vi "ControlProgram5.2.vi"() -> ()   [LabVIEW 2016]
uses:
  <vilib>/Utility/error.llb/DialogType.ctl
  <vilib>/Utility/miscctls.llb/LVPoint32TypeDef.ctl
  <vilib>/DAQmx/write.llb/DAQmx Write (Digital Bool 1Line 1Point).vi
  <vilib>/DAQmx/create/channels.llb/DAQmx Create Channel (DO-Digital Output).vi
  <vilib>/platform/TimedLoop/XDataNode/XDataNode.xnode
  <vilib>/Platform/TimedLoop/XDataNode/nitl_modes.ctl
  <vilib>/Platform/TimedLoop/XDataNode/XDNodeRunTimeDep.lvlib
  <vilib>/Platform/TimedLoop/XDataNode/wakeup.ctl
  <vilib>/Platform/TimedLoop/XDataNode/timing_clust.ctl
  <vilib>/DAQmx/create/channels.llb/DAQmx Create Channel (AI-Voltage-Basic).vi
  <vilib>/DAQmx/create/channels.llb/DAQmx Create Channel (AO-Voltage-Basic).vi
  <vilib>/DAQmx/write.llb/DAQmx Write (Analog 1D DBL NChan 1Samp).vi
  <resource>/objmgr/daqmx.rc
  <vilib>/Analysis/NI_AALBase.lvlib
  <vilib>/Analysis/baseanly.llb/Mean (DBL).vi
  <vilib>/Instr/_visa.llb/VISA Configure Serial Port (Instr).vi
  <vilib>/DAQmx/read.llb/DAQmx Read (Analog 2D DBL NChan NSamp).vi
  <vilib>/Utility/inputDevices.llb/closeMouse.vi
  <vilib>/Utility/inputDevices.llb/mouseAcquire.vi
  <vilib>/DAQmx/configure/timing.llb/DAQmx Timing (Sample Clock).vi
panel:
  in  "dt":dbl
  out "Flush Sample Start Time":u32
  out "Sample flush time (s)":dbl=100.0
  in  "Inject Sample":bool
  out "Chart Freq (Hz)":dbl
  out "Waveform Chart 3":dbl[][](graph)
  out "Cal values":T1={"AX alpha"=672.9952101249002, "BX alpha"=822.8320399167465, "AX kappa"=0.3432739170419873, "BX kappa"=0.22087046979741862, "AX offset"=-0.002065833400375715, "BX offset"=0.010483360643544744, "AY alpha"=702.0654168010462, "BY alpha"=773.6701766674906, "AY kappa"=0.33643150106915, "BY kappa"=0.2444549177225145, "AY offset"=-0.1177594339643395, "BY offset"=0.06470506082263472}
  in  "Inject Pump 1":bool
  in  "Inject Pump 2":bool
  in  "Tab Control 2":T2(tab)
  in  "Force FB script":bool
  in  "Got ADig bead":bool
  in  "Move Cap. 2 (ADig Top)":bool
  in  "Dump beads":bool
  in  "Got DNA bead":bool
  in  "Flow on\ncap 2?":bool=TRUE
  in  "Flow on\ncap 1?":bool=TRUE
  in  "Flow on\ndump?":bool=TRUE
  in  "Delta after tether":dbl=3.1
  in  "TA Cancel Save?":bool
  in  "Min fish\ndelta (V)":dbl=2.8 min=0.0 max=10.0 step=0.1
  in  "Max fish\ndelta (V)":dbl=3.8 min=0.0 max=10.0 step=0.1
  in  "Fish Speed (ms)":i32=3000
  in  "Wait (ms)":i32=1500
  in  "# attempts":dbl=10.0
  in  "Cutoff force (pN)":dbl=5.0
  in  "Raster after\n tether?":bool=TRUE
  out "Tether":bool
  out "Attempt #":i32
  in  "Flow on\nwhile fish?":bool=TRUE
  in  "Flow on\nafter raster?":bool=TRUE
  in  "Cal @ Delta (V)":dbl=5.0
  in  "Cal stage position":i32=3
  in  "Conv Y (nm/V)":dbl=505.0
  in  "Conv X (nm/V)":dbl=892.0
  out "Cal Final Sampling Rate":dbl
  in  "Cal Averaging":i32=1
  in  "Wait before dip (s)":dbl=3.0
  in  "Start dipping after?":bool
  in  "Start trap delta (V)":dbl=3.85
  in  "Cancel dwell":bool
  in  "Pause dwell":bool
  in  "Return position":dbl=3.0
  in  "Dip duration":dbl=15.0
  in  "Dip position":dbl=4.0
  in  "Dip":bool
  out "Dip time":i32
  in  "Stop":bool=TRUE
  in  "?":T3(tab)=enum."Mouse control"
  in  "Save N sets":bool
  in  "N sets":i32=200
  in  "Cal sets to save":i32=500
  in  "Reset data stream":bool
  out "Buffer Overflow":bool
  out "Stage moving":bool
  in  "Comment":string="wtUvrD 0.5 uM ATP"
  in  "Raster scan":bool
  out "Saving":bool
  in  "Save cal":bool
  in  "Save Data":bool
  in  "Stop saving":bool
  out "Calibrating":bool
  out "Progress":dbl(slide) scale=0.0..100.0
  in  "Read Cal":bool
  in  "Fish":bool
  in  "Averaging Number":i32=1250
  out "Final Sampling Rate":dbl=100.0
  in  "Trap position":cluster{"X":dbl, "Y":dbl}={"X"=1.6, "Y"=4.95}
  in  "Trap delta":dbl=5.1 min=0.0 max=10.0 step=0.1
  in  "Fixed X":dbl=1.6
  in  "Fixed Y":dbl=0.7
  in  "Shutter 1 (B)":bool
  in  "Shutter 2 (A)":bool
  in  "Pulling direction":bool=TRUE
  out "Raster scanning...":bool
  out "Current file name":path
  in  "AX alpha":dbl format="%#_3p"
  in  "BX alpha":dbl format="%#_3g"
  in  "AX kappa":dbl format="%#_3g"
  in  "BX kappa":dbl format="%#_3g"
  in  "AX offset":dbl format="%#_3g"
  in  "BX offset":dbl format="%#_3g"
  in  "AY alpha":dbl format="%#_3g"
  in  "BY alpha":dbl format="%#_3g"
  in  "AY kappa":dbl format="%#_3g"
  in  "BY kappa":dbl format="%#_3g"
  in  "AY offset":dbl format="%#_3g"
  in  "BY offset":dbl format="%#_3g"
  out "Buffer status":u8(slide) scale=0.0..100.0
  in  "dump spot":string="Dump beads spot"
  in  "up flow spot":string="Upper flow spot"
  in  "low flow spot":string="Lower flow spot"
  in  "up cap":string="Upper capillary (ADig beads)"
  in  "bottom cap":string="Lower capillary (DNA beads)"
  in  "Move to Position 5":bool
  in  "Set Position 5":bool
  in  "Saved stage positions":dbl[][](array[numeric])=[[1.0, 0.0, 0.0, 0.0], [2.0, 0.28481, -2.63158, -0.02256], [3.0, 1.27978, -0.73974, 0.0], [4.0, 1.27978, -2.1978, 0.0], [5.0, 0.03306, -2.63158, -0.02256]]
  in  "Set Position 2":bool
  in  "Move to Position 2":bool
  in  "Set Position 1":bool
  in  "Move to Position 1":bool
  in  "Set Position 4":bool
  in  "Move to Position 4":bool
  in  "Set Position 3":bool
  in  "Move to Position 3":bool
  out "Stage error":errorcluster
  in  "Clear Volume":bool
  out "Sample Flush Meter":u8(slide) scale=0.0..100.0
  out "Flushing Sample":bool
  in  "Flush Sample":bool
  in  "Normal \nRate (ul/hr)  3":dbl=100.0
  in  "Normal \nVolume (ul) 3":dbl=300.0
  in  "Normal \nVolume (ul) 2":dbl
  in  "Normal \nRate (ul/hr)":dbl
  in  "Normal \nVolume (ul)":dbl
  in  "Flush\nRate (ul/min)":dbl
  in  "Flush\nVolume (ul)":dbl
  in  "Flush \nRate (ul/min)  2":dbl
  in  "Flush Pump 2":bool
  in  "Flush\nVolume (ul)  2":dbl
  in  "Flush Pump 1":bool
  in  "Normal \nRate (ul/hr)  2":dbl
  in  "Write Wait":i32=1000
  in  "Flush \nRate (ul/min)  3":dbl=100.0
  in  "Flush\nVolume (ul)  3":dbl=100.0
  out "error out":errorcluster
  in  "Use Mouse to Move Trap?":bool
  in  "Pause Mouse/Mirror Connection":bool
  out "Reference Voltage":cluster{dbl, dbl}={0.0, -0.0}
  out "Saved voltage":cluster{dbl, dbl}
  out "Real Coordinates":cluster{"Horizontal":i32, "Vertical":i32}={"Horizontal"=145, "Vertical"=-1746}
  out "CoordinatesMousePressed":T4
  out "Sum error":dbl(knob) scale=-0.2..0.2
  out "Trap sep":waveform(dbl)[](graph)
  in  "Set reading to\nsetpoint":bool
  in  "Offset Y (nm)":dbl format="%0.2f"
  in  "Offset X (nm)":dbl format="%0.2f"
  in  "Remove offsets":bool
  in  "Force Feedback":bool
  out "Feedback Output Voltage 2":cluster{dbl, dbl} {"?" format="%#_4g"; "?" format="%#_4g"}
  in  "Max value X":dbl=10.0 format="%.1f"
  in  "Min value X":dbl format="%0.1f"
  in  "Max value Y":dbl=10.0 format="%.1f"
  in  "Min value Y":dbl format="%.1g"
  in  "Offset":cluster{"Off Y":dbl, "Off X":dbl}={"Off Y"=1.5, "Off X"=0.17}
  in  "Setpoint voltage":cluster{"SP Y":dbl, "SP X":dbl}={"SP Y"=0.6, "SP X"=0.0}
  in  "Feedback const":T5={"Ki_B_Y"=0.5, "Ki_B_X"=0.0, "Kp Y"=1.0, "Kp X"=0.0}
  out "Mean Trap Pos X 2 (nm)":dbl format="%0.2f"
  out "Mean Trp Pos Y 2 (nm)":dbl format="%0.2f"
  out "T2 X RMS (A)":dbl format="%0.2f"
  out "T2 Y RMS (A)":dbl format="%0.2f"
  in  "Save scans":bool=TRUE
  in  "# scans":i32=1
  in  "Speed (ms)":i32=10000
  in  "Min delta":dbl=3.2
  in  "Load param":bool
  in  "Max delta":dbl=4.1
  in  "Scan Parameters":T6(array[cluster])=[{"Label"="Offset", "Max delta 2"=3.8, "Min delta 2"=2.4, "Speed (ms) 2"=10000, "# scans 2"=1}]
  in  "Trap delta\nafter":dbl=3.6
  in  "Stop raster":bool
  out "Scan Range (nm)":dbl
  out "Scan Speed (nm/s)":dbl
  out "Continue to display?":bool
  out "Video Error":errorcluster
  in  "# Samples/channel (in)":i32=40000 format="%.2f"
  out "Buffer size\n(Samples/channel)":u32
  out "DAQ rate\n(Samples/s)":dbl format="%#_6p"
  out "# Samples/channel":i32=1250
  out "# Samples/channel/s":dbl
  out "AvailSampPerChan":u32
  out "Data update period (s/set)":dbl format="%#_6p"
  out "AvailSampPerChan 2":u32
  in  "PC samp per channel":i32=1000
  in  "Sampling Rate":dbl=125000.0 format="%0.0p"
  in  "DAQ Rate2":dbl=1000000.0 format="%#_6p"
  out "Data period (s)":dbl format="%#_6p"
  in  "Tether break\nforce (pN)":dbl=1.0
  in  "Path":path=path "D:/data"
  in  "Save file index":dbl
  out "Mirror task":refnum<k21>
  in  "HWP1":string="Half waveplate 1: differential trap power"
  in  "HWP0":string="Half waveplate 0: total trap power"
  in  "Move 1":bool
  in  "\"Degrees\" 1":dbl
  in  "Move 0":bool
  in  "\"Degrees\" 0":dbl
  out "Chamber":T7(plugin-control)
  out "Deflection":T4
  in  "Sampling Rate":dbl=125000.0 format="%0.2f"
  in  "Averaging Number":i32=12500
  in  "DAQ Rate":dbl=1000000.0
  out "Final Sampling Rate":dbl
  in  "Tab Control":T8(tab)
  in  "Downsamp\nfact":dbl=250.0
  out "Bead sep":waveform(dbl)[](graph)
  out "Force (pN)":waveform(dbl)[](graph)
  out "Mean force (pN)":dbl format="%0.2f"
  out "Force noise (pN)":dbl format="%0.2f"
  out "Mean Bead Sep\n(nm)":dbl format="%0.2f"
  out "Bead Sep Noise\n(A)":dbl format="%0.2f"
  out "Saved Trap Pos":dbl[][](graph)
  out "PSD 2":cluster{dbl[], dbl[]}(graph)
  out "PSD 1":cluster{dbl[], dbl[]}(graph)
  out "PSD 1 Sum":dbl(slide) scale=0.0..10.0
  out "PSD 2 Sum":dbl(slide) scale=0.0..10.0
  in  "Start":bool
  out "All signals":waveform(dbl)[](graph)
  # "Bead Calibration"
  # "X"
  # "Y"
  # "Pump #1 Controls"
  # "Pump #2 Controls"
  # "Sample Pump Controls"
  # "Retract the pumps manually. Change it back to INFUSE when you're done. Suck it up, don't whine."
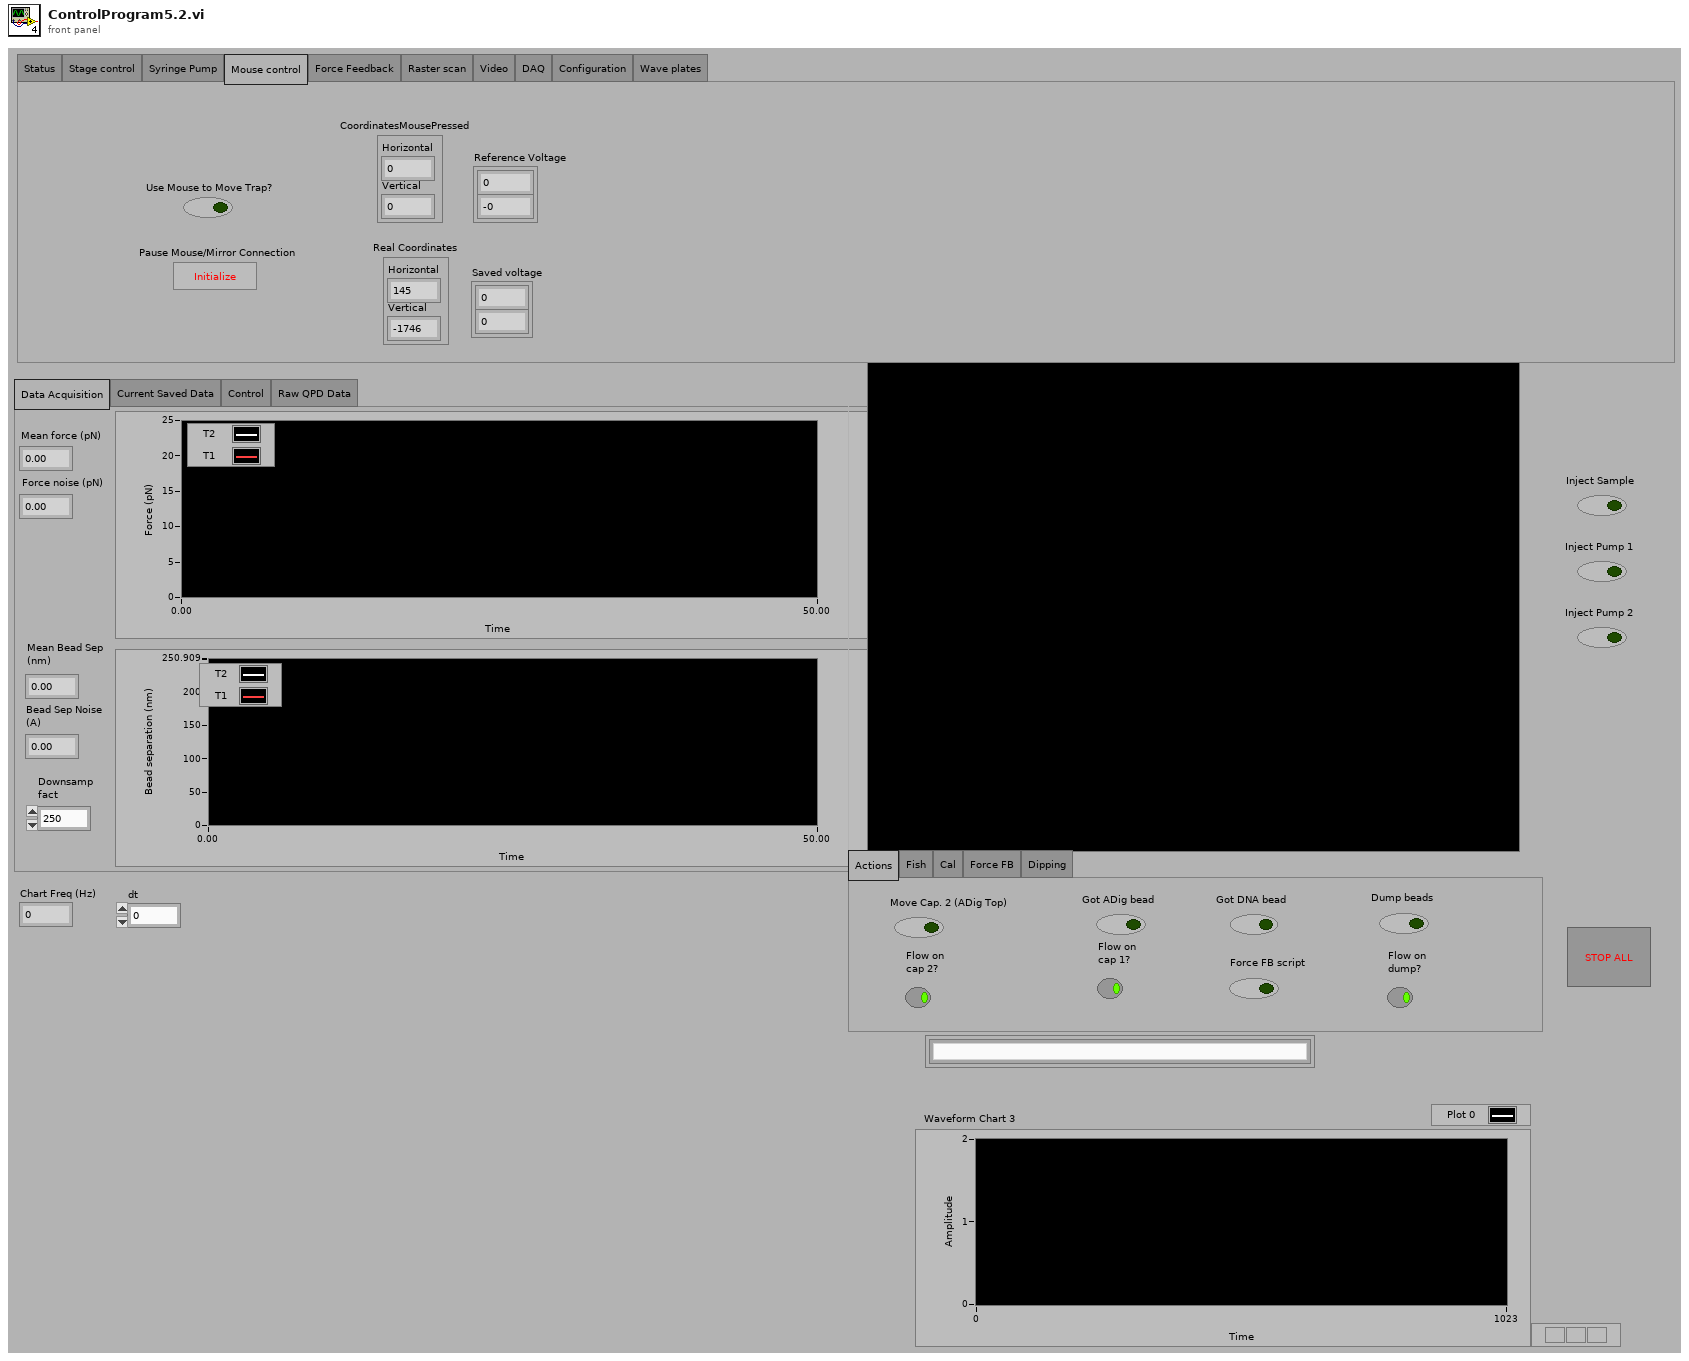
[diagram p1: front panel]
types:
  T1 = cluster{"AX alpha":dbl, "BX alpha":dbl, "AX kappa":dbl, "BX kappa":dbl, "AX offset":dbl, "BX offset":dbl, "AY alpha":dbl, "BY alpha":dbl, "AY kappa":dbl, "BY kappa":dbl, "AY offset":dbl, "BY offset":dbl}
  T2 = enum32{"Actions", "Fish", "Cal", "Force FB", "Dipping"}
  T3 = enum32{"Status", "Stage control", "Syringe Pump", "Mouse control", "Force Feedback", "Raster scan", "Video", "DAQ", "Configuration", "Wave plates"}
  T4 = typedef "LVPoint32TypeDef.ctl" = cluster{"Horizontal":i32, "Vertical":i32}
  T5 = cluster{"Ki_B_Y":dbl, "Ki_B_X":dbl, "Kp Y":dbl, "Kp X":dbl}
  T6 = cluster{"Label":string, "Max delta 2":dbl, "Min delta 2":dbl, "Speed (ms) 2":i32, "# scans 2":i32}[]
  T7 = typedef "IMAQ Image.ctl" = refnum<image>
  T8 = enum32{"Data Acquisition", "Current Saved Data", "Control", "Raw QPD Data"}
  T9 = enum16{"open", "replace", "create", "open or create", "replace or create", "replace or create with confirmation"}
  T10 = enum16{"big-endian, network order", "native, host order", "little-endian"}
  T11 = cluster{string, string, string, string, string, string, string, string}
  T12 = typedef "XDNodeRunTimeDep.lvlib/timing_clust.ctl" = cluster{"Expected End [f-1]":u64, "Actual End [f-1]":u64, "Finished Late? [f-1]":bool, "Expected End [i-1]":u64, "Actual End [i-1]":u64, "Finished Late? [i-1]":bool, "Expected Start [i]":u64, "Actual Start [i]":u64, "Expected Start [f]":u64, "Actual Start [f]":u64, "Source Name":string, "Structure Name":string, "Period":i64, "Deadline":i64, "Offset":i64, "Start":i64, "Priority":i32, "Timeout":i32, "Mode":T13, "Wakeup Reason":T14, "Error":errorcluster, "Source Type":string, "Secondary Source Type":string, "Global End Time":u64, "Global Start Time":u64, "Frame Duration":u64, "Iteration Duration":u64, "Assigned CPU":i32, "I/O Scan Engine Mode":u32}
  T13 = typedef "XDNodeRunTimeDep.lvlib/nitl_modes.ctl" = enum32{"No Change", "Process missed periods, maintain original phase", "Discard missed periods, maintain original phase", "Process missed periods, ignore original phase", "Discard missed periods, ignore original phase"}
  T14 = typedef "XDNodeRunTimeDep.lvlib/wakeup.ctl" = enum32{"Normal", "Aborted", "Asynchronous wakeup", "Timing source error", "Timed loop error", "Timeout"}
  T15 = typedef "DialogType.ctl" = u16
  T16 = cluster{"button 1":bool, "button 2":bool, "button 3":bool, "button 4":bool}
  T17 = cluster{"[0]":dbl, "[1]":dbl, "[2]":dbl, "[3]":dbl, "[4]":dbl, "[5]":dbl, "[6]":dbl, "[7]":dbl, "[8]":dbl, "[9]":dbl, "[10]":dbl, "[11]":dbl}
  T18 = cluster{"Label":string, "Max delta 2":dbl, "Min delta 2":dbl, "Speed (ms) 2":i32, "# scans 2":i32}
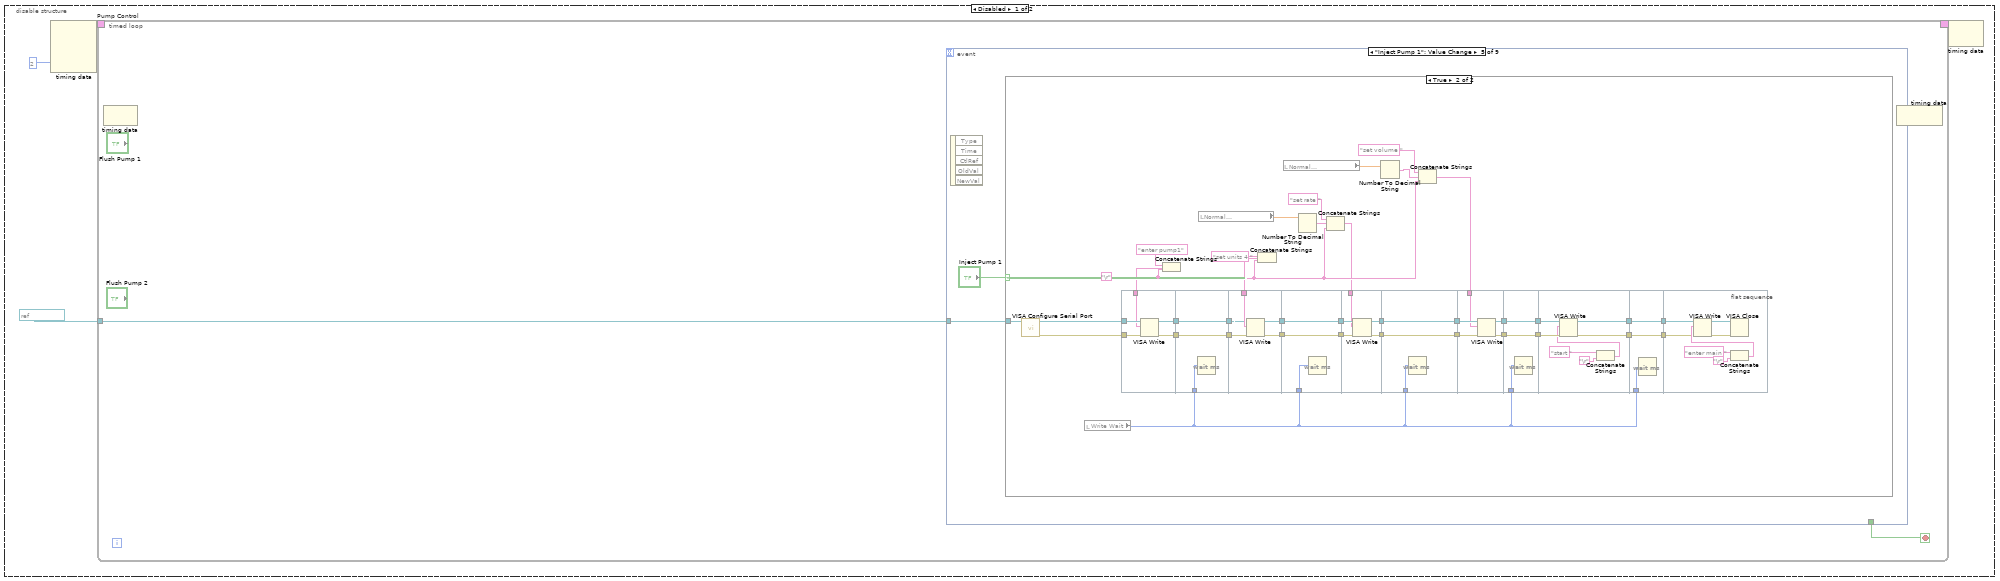
[diagram p2: hidden frame]
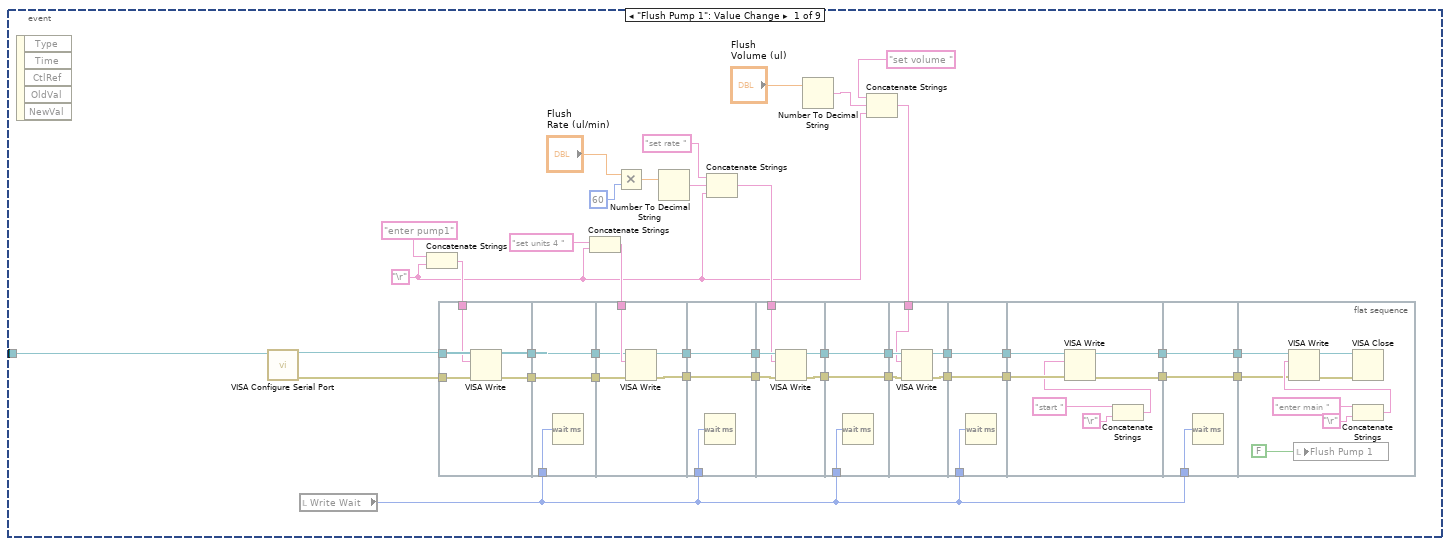
[diagram p3: hidden frame]
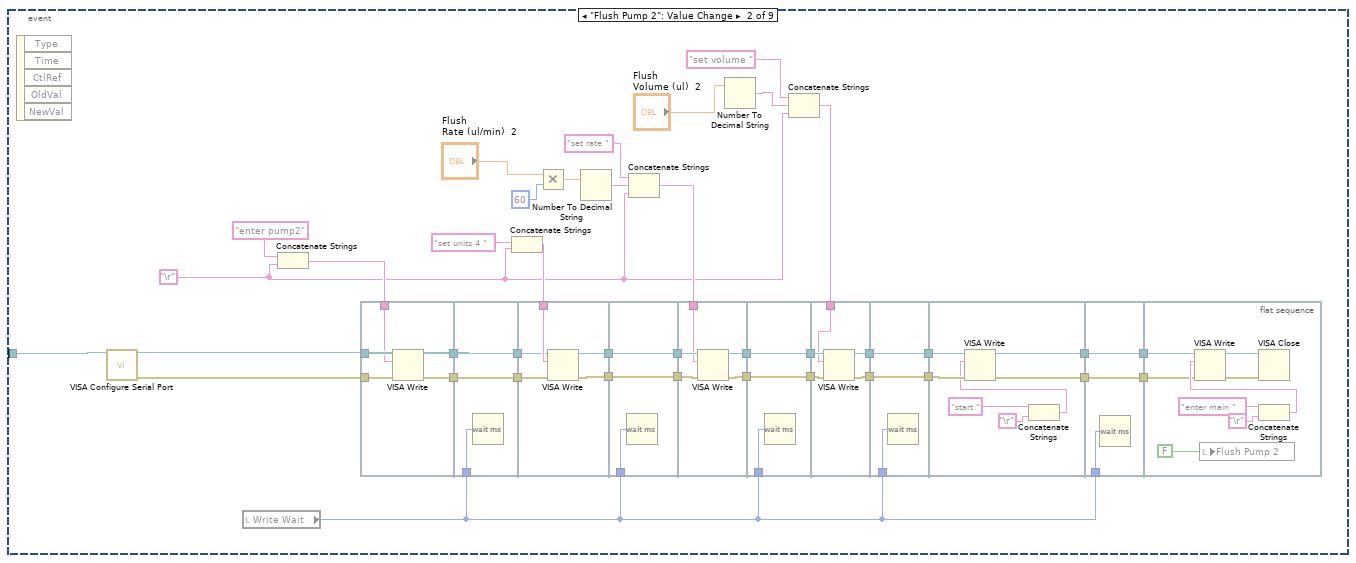
[diagram p4: hidden frame]
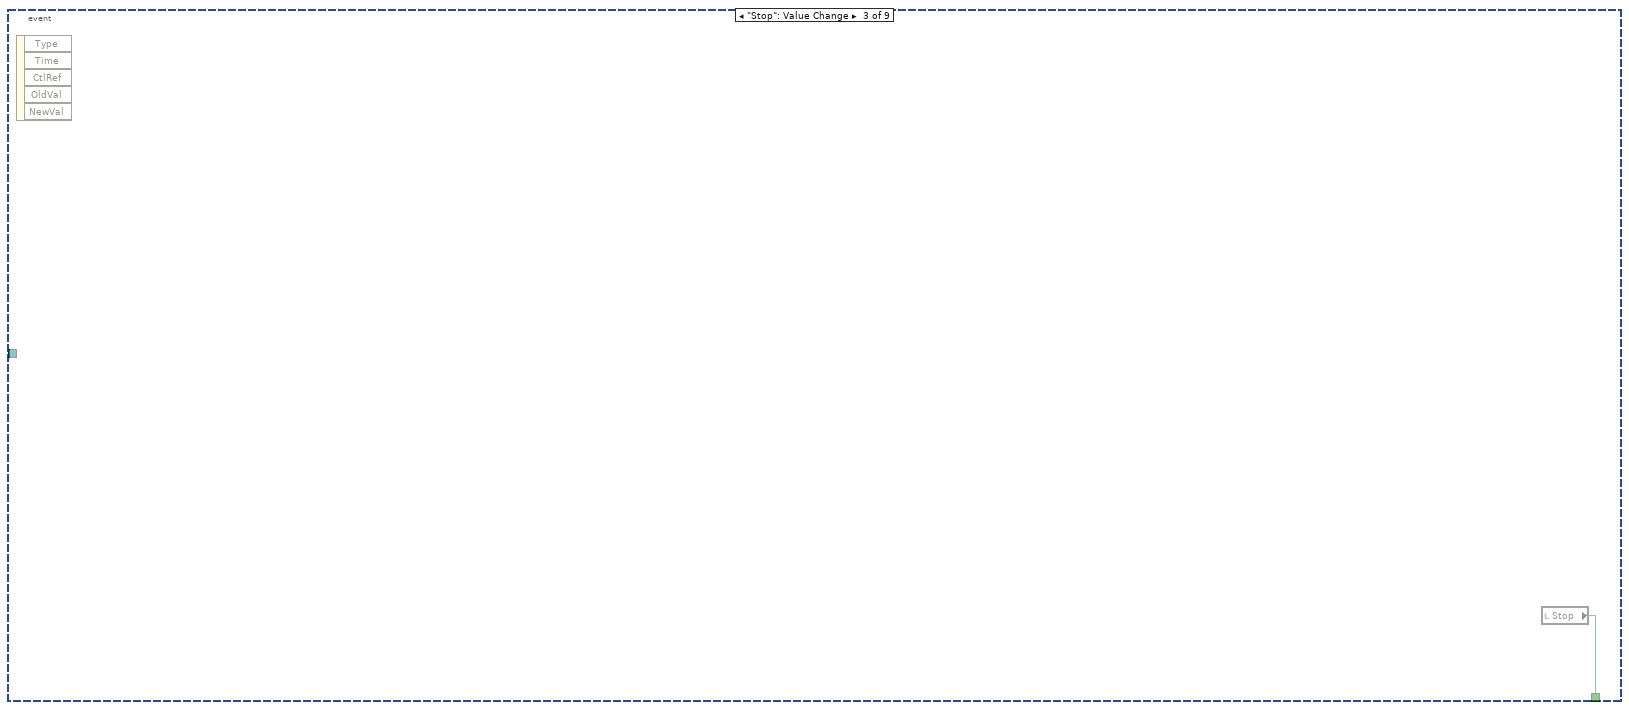
[diagram p5: hidden frame]
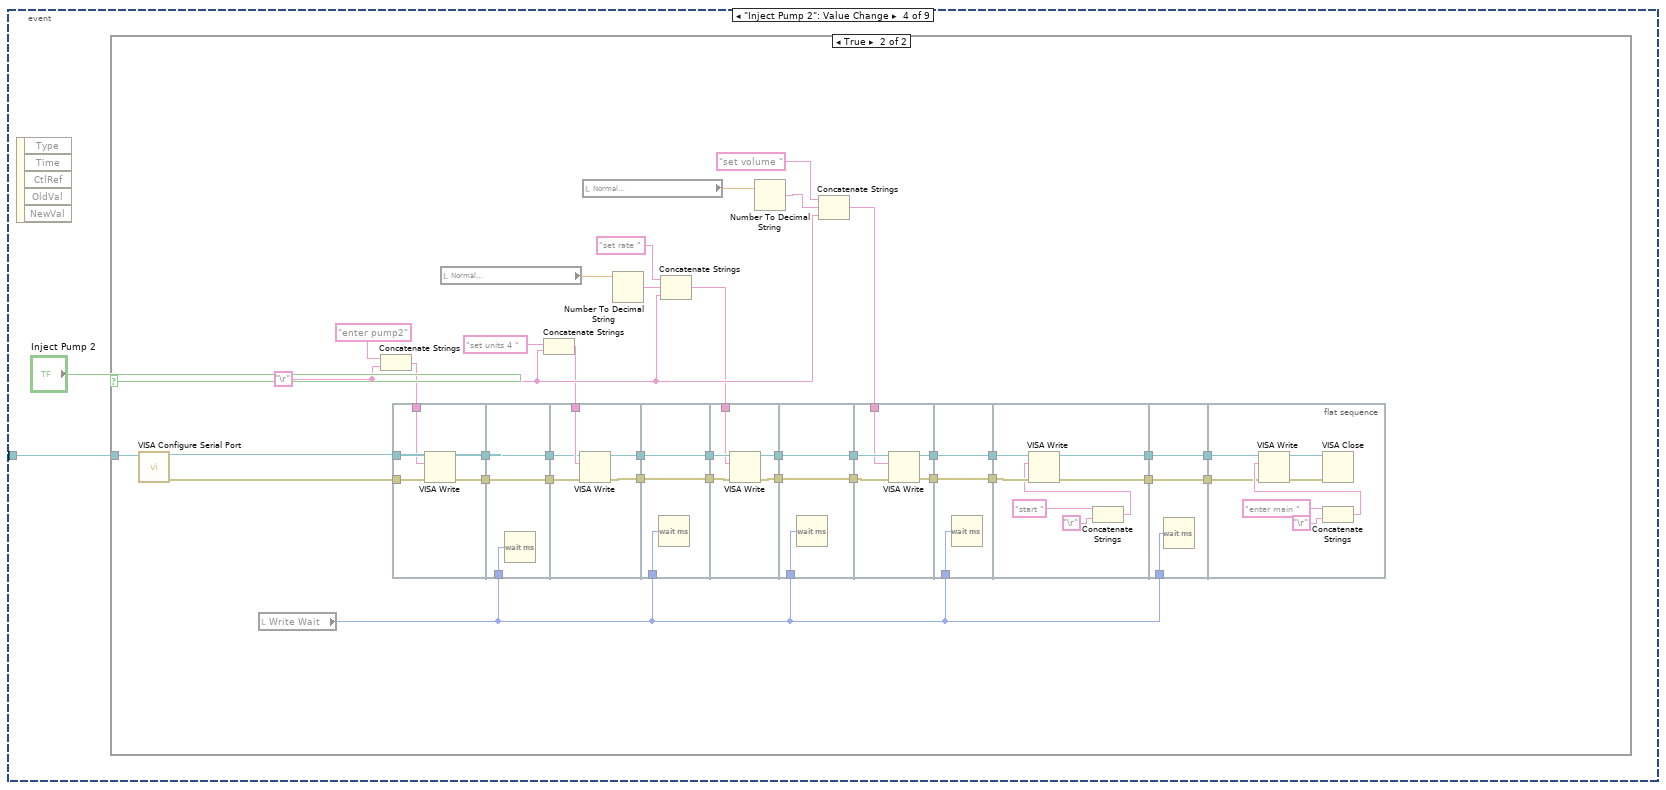
[diagram p6: hidden frame]
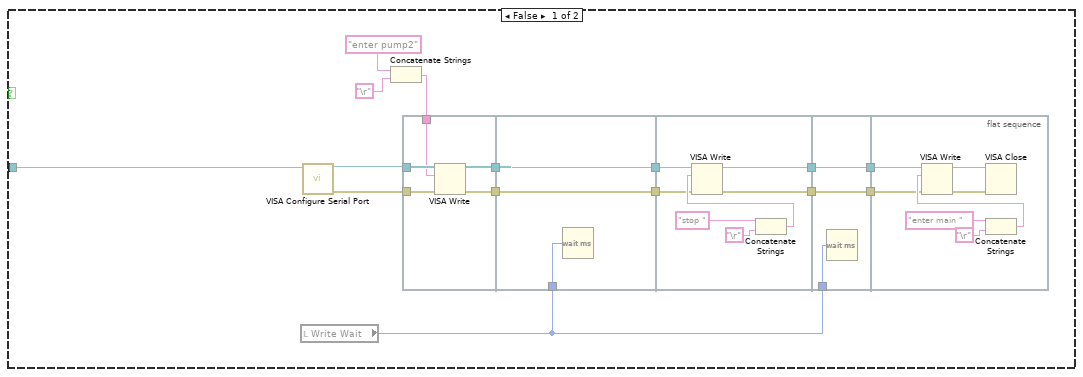
[diagram p7: hidden frame]
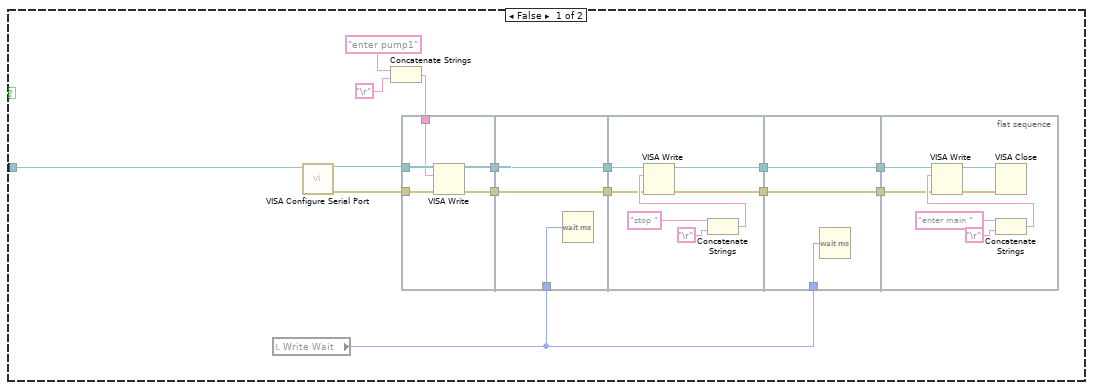
[diagram p8: hidden frame]
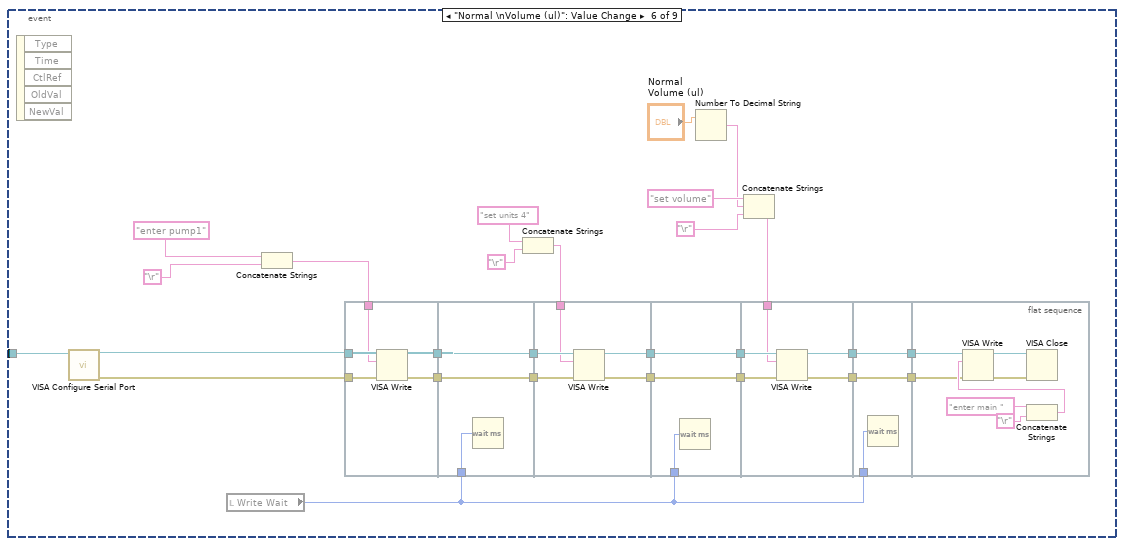
[diagram p9: hidden frame]
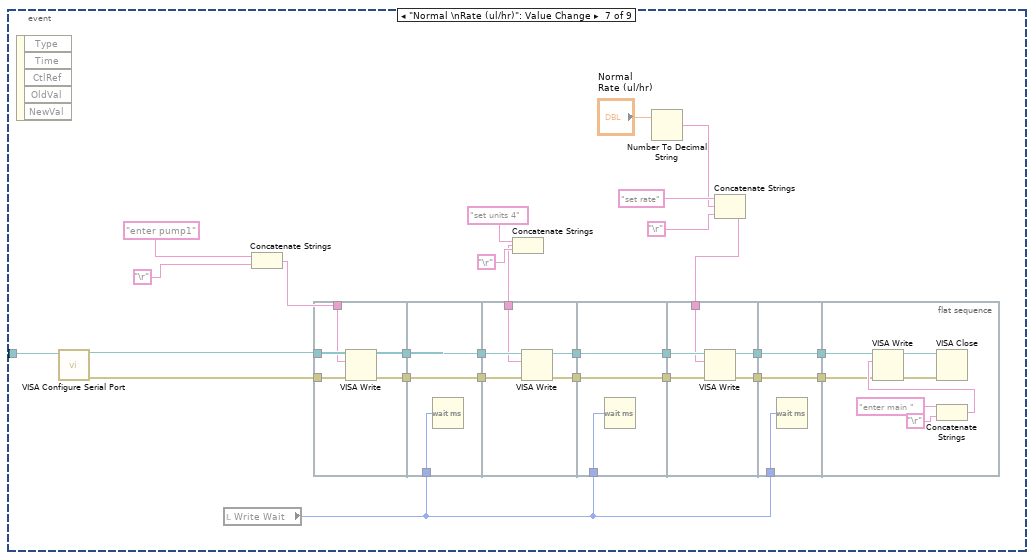
[diagram p10: hidden frame]
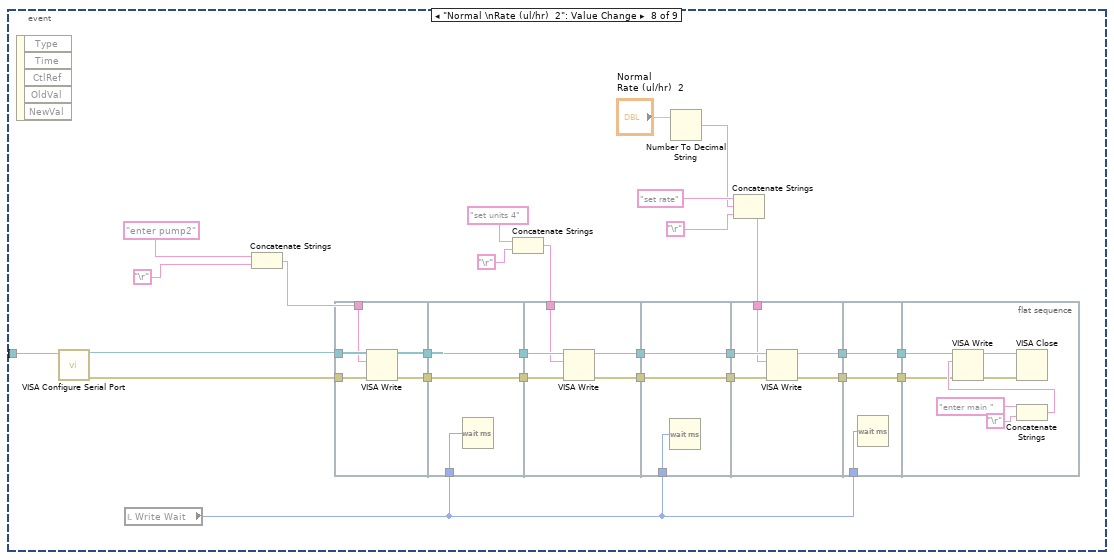
[diagram p11: hidden frame]
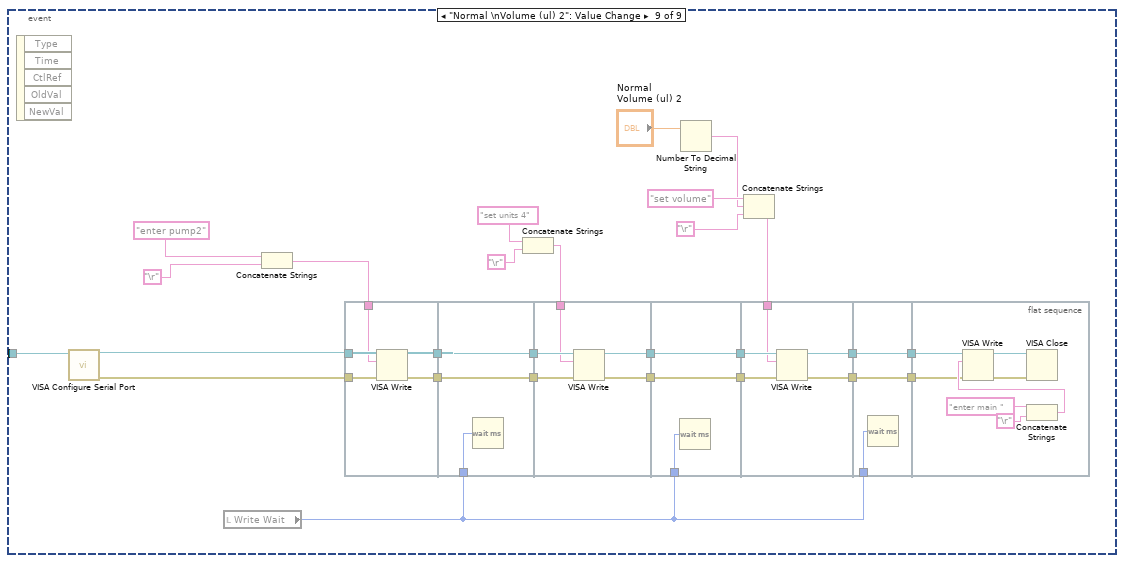
[diagram p12: hidden frame]
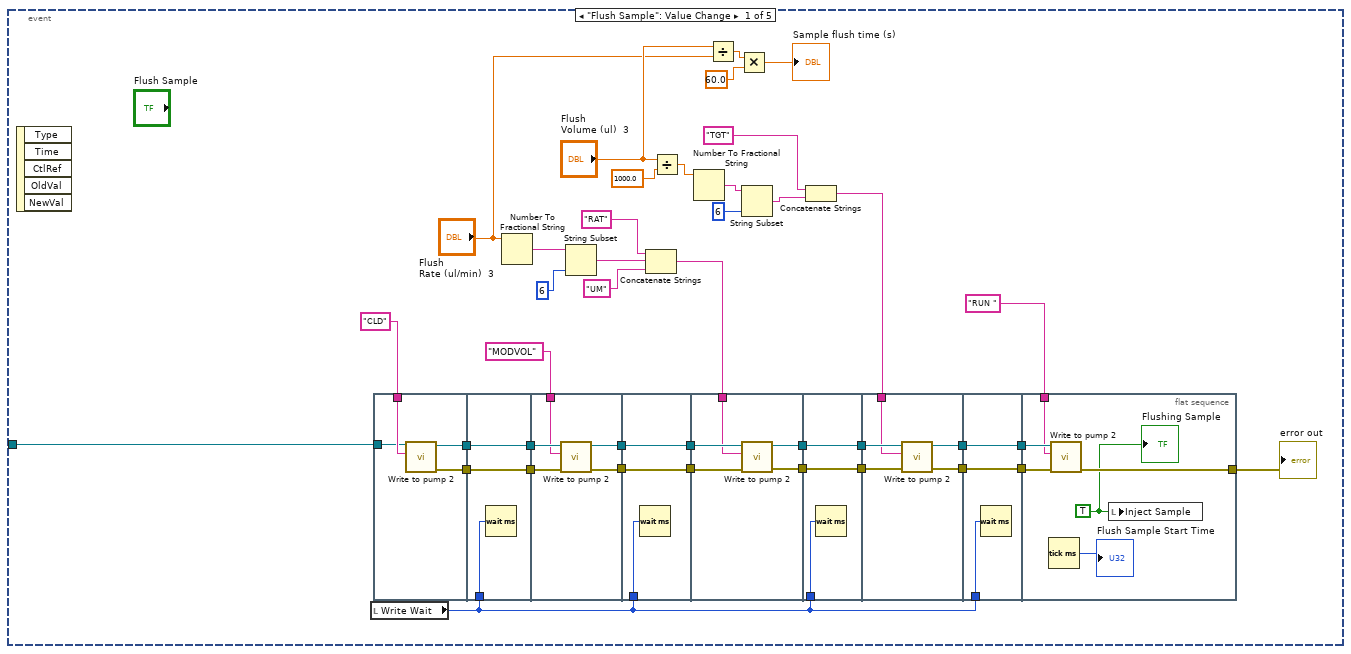
[diagram p13: hidden frame]
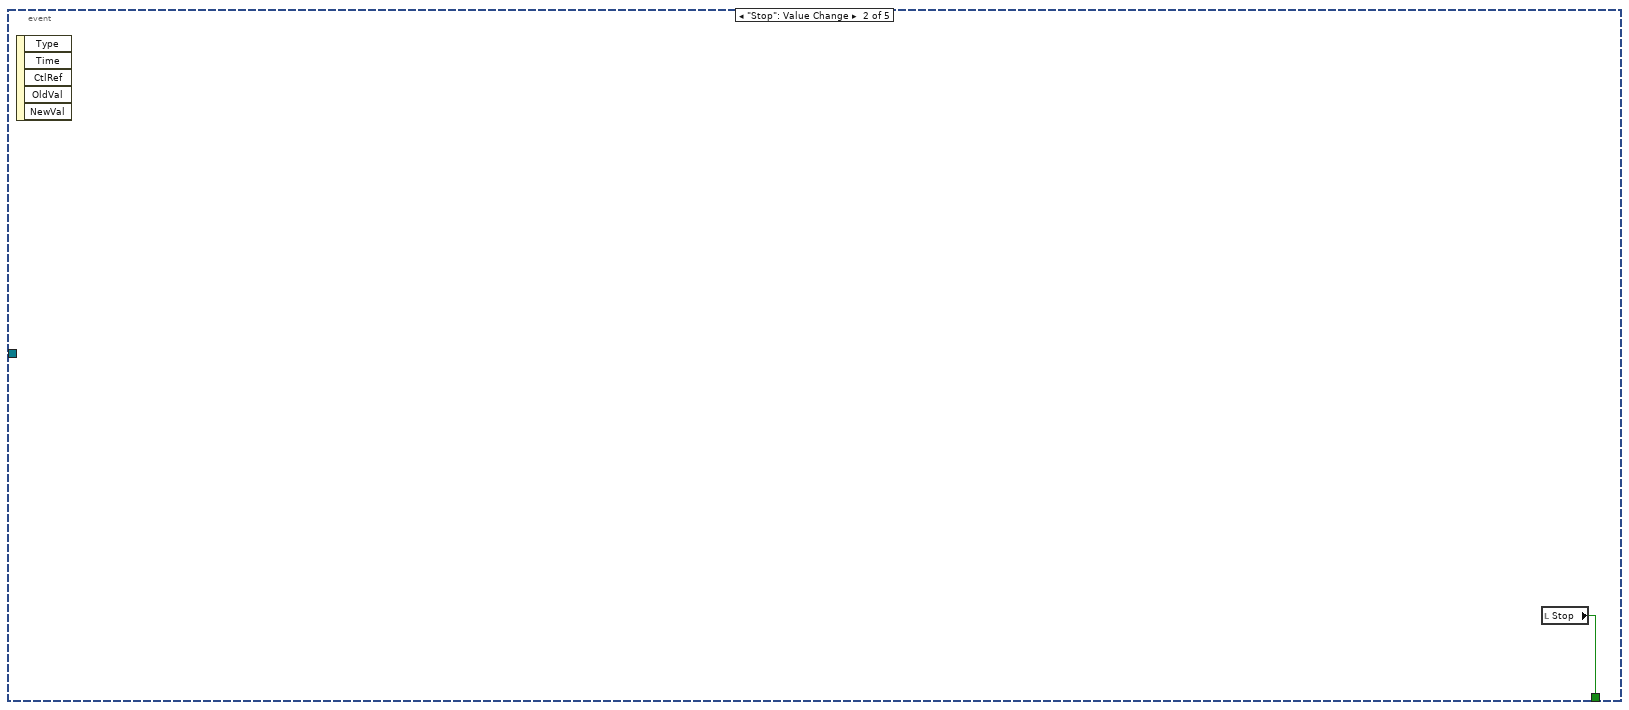
[diagram p14: hidden frame]
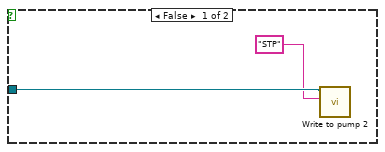
[diagram p15: hidden frame]
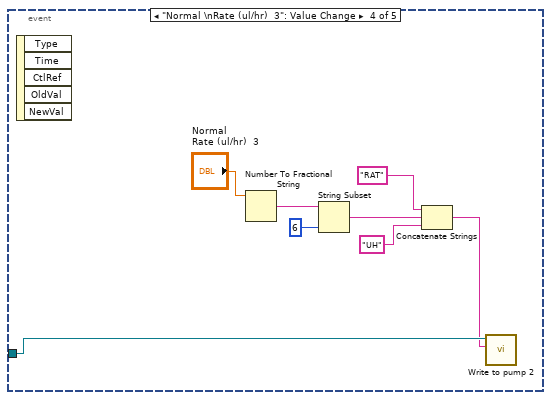
[diagram p16: hidden frame]
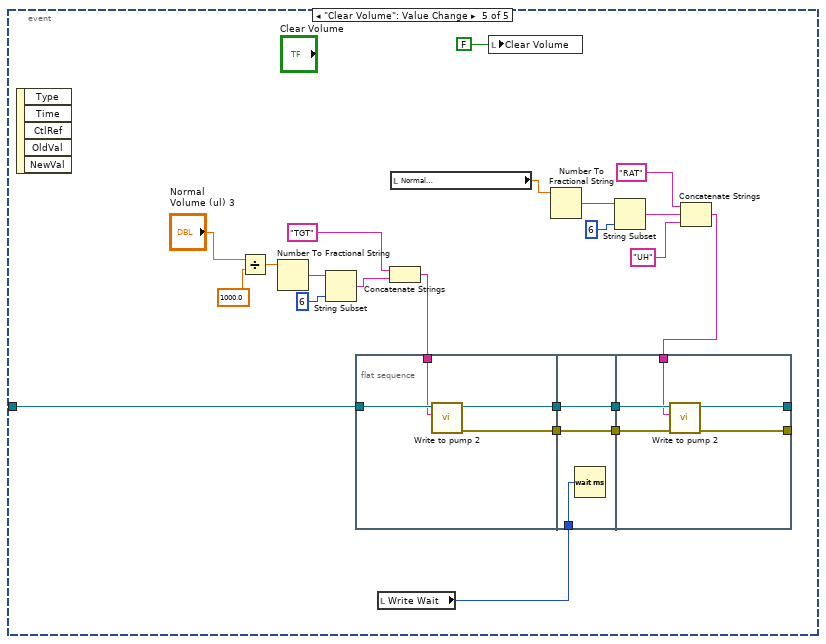
[diagram p17: hidden frame]
diagram:
  w42 = 10.0 ("Minimum Value")
  w43 = -10.0 ("Minimum Value")
  w45 = -2.0 ("Minimum Value")
  w46 = 2.0 ("Maximum Value")
  w71 = 10123 items=["Finite Samples"=10178, "Continuous Samples"=10123] ("sample mode")
  w92 = tag "Dev1/port2/line1"  # Shutter 2
  w95 = tag "Dev1/port1/line4"  # Shutter 1
  # "Create channels for movable mirror"
  # "Create channels for detectors"
  n1 = call-poly <vilib>:"DAQmx Create Virtual Channel.vi"("maximum value"=w46, "minimum value"=w45, "physical channels"=tag "Dev1/ai0" ("Physical Channel")) -> ("task out"=w47:refnum<k21>, "error out"=w70:errorcluster)  [unwired: 11 in]
  n2 = call-poly <vilib>:"DAQmx Create Virtual Channel.vi"("task in"=w47, "maximum value"=w46, "minimum value"=w45, "physical channels"=tag "Dev1/ai1", "error in"=w70) -> ("task out"=w68:refnum<k21>, "error out"=w67:errorcluster)  [unwired: 9 in]
  n3 = call-poly <vilib>:"DAQmx Create Virtual Channel.vi"("task in"=w68, "maximum value"=w46, "minimum value"=w45, "physical channels"=tag "Dev1/ai2", "error in"=w67) -> ("task out"=w59:refnum<k21>, "error out"=w58:errorcluster)  [unwired: 9 in]
  n4 = call-poly <vilib>:"DAQmx Create Virtual Channel.vi"("task in"=w59, "maximum value"=w46, "minimum value"=w45, "physical channels"=tag "Dev1/ai3" ("Physical Channel"), "error in"=w58) -> ("task out"=w44:refnum<k21>, "error out"=w64:errorcluster)  [unwired: 9 in]
  n5 = call-poly <vilib>:"DAQmx Create Virtual Channel.vi"("task in"=w44, "maximum value"=w42, "minimum value"=w43, "physical channels"=tag "Dev1/ai4", "error in"=w64) -> ("task out"=w62:refnum<k21>, "error out"=w61:errorcluster)  [unwired: 9 in]
  n6 = call-poly <vilib>:"DAQmx Create Virtual Channel.vi"("task in"=w62, "maximum value"=w42, "minimum value"=w43, "physical channels"=tag "Dev1/ai5", "error in"=w61) -> ("task out"=w57:refnum<k21>, "error out"=w56:errorcluster)  [unwired: 9 in]
  n7 = call-poly <vilib>:"DAQmx Create Virtual Channel.vi"("task in"=w57, "maximum value"=w42, "minimum value"=w43, "physical channels"=tag "Dev1/ai6", "error in"=w56) -> ("task out"=w51:refnum<k21>, "error out"=w49:errorcluster)  [unwired: 9 in]
  n8 = call-poly <vilib>:"DAQmx Create Virtual Channel.vi"("task in"=w51, "maximum value"=w42, "minimum value"=w43, "physical channels"=tag "Dev1/ai7", "error in"=w49) -> ("task out"=w50:refnum<k21>, "error out"=w48:errorcluster)  [unwired: 9 in]
  n9 = call-poly <vilib>:"DAQmx Timing.vi"("task/channels in"=w50, "sample mode"=w71, "samples per channel"="PC samp per channel", "rate"="Sampling Rate", "error in"=w48) -> ("task out"=w54:refnum<k21>, "error out"=w53:errorcluster)  [unwired: 9 in]
  n10 = call-poly <vilib>:"DAQmx Create Virtual Channel.vi"("maximum value"="Max value Y", "minimum value"="Min value Y", "physical channels"=tag "Dev1/ao1" ("Trap X Axis")) -> ("task out"=w39:refnum<k21>, "error out"=w41:errorcluster)  [unwired: 11 in]
  n11 = property class="DAQmx Timing"(reference=w54, error in=w53, "More:AI Convert:Rate"="DAQ Rate2") -> (reference out=w6:refnum<k21>, error out=w5:errorcluster, "SampClk.Rate"=→"DAQ rate\n(Samples/s)":dbl)
  n12 = call-poly <vilib>:"DAQmx Create Virtual Channel.vi"("task in"=w39, "maximum value"="Max value X", "minimum value"="Min value X", "physical channels"=tag "Dev1/ao0" ("Trap Y Axis"), "error in"=w41) -> ("task out"=w30:refnum<k21>, "error out"=w29:errorcluster)  [unwired: 9 in]
  "Mirror task" <- w30
  n13 = property class="DAQmx Buffer"(reference=w6, error in=w5) -> (reference out=w3:refnum<k21>, error out=w2:errorcluster, "Input.OnbrdBufSize"=→"Buffer size\n(Samples/channel)":u32)
  n14 = call <vilib>:"DAQmx Start Task.vi"("task/channels in"=w3, "error in"=w2) -> ("task out"=w31:refnum<k21>)  [unwired: 12 in, 1 out]
  n15 = while {
    tunnel: [w415] -> w77
    tunnel: [w307] -> w78
    tunnel: [w423] -> w76
    tunnel: [w420] -> w73
    tunnel: w31 -> [w120]
    tunnel: w30 -> [w416]
    tunnel: w29 -> [w421]
    stop <- w420 stop-if-true
    w151 = "NI_ChannelName" ("name")
    w227 = -1
    # "Rewire everything"
    # "Invert these because changed\nfrom PSD to QPD"
    # "Trap Y"
    # "Trap X"
    # "Convert to\npN"
    # "Convert to\nnm"
    # "Subtract\noffset"
    # "Normalize by\nsum"
    # "B sum"
    # "BX"
    # "BY"
    # "AX"
    # "AY"
    # "A sum"
    # "Close files when done saving"
    n16 = property class="DAQmx Read"(reference=w120) -> (reference out=w119:refnum<k21>, "AvailSampPerChan"=→"AvailSampPerChan 2":u32)  [unwired: 1 in, 1 out]
    n17 = local read "Averaging Number"() -> (w115:i32)
    n18 = local read "Averaging Number"() -> (w121:i32)
    "# Samples/channel" <- w121
    n19 = local read "Sampling Rate"() -> (w419:dbl)
    n20 = call-poly <vilib>:"DAQmx Read.vi"("task/channels in"=w119, "number of samples per channel"=w115, "timeout"=10.0) -> ("task out"=w306:refnum<k21>, "data"=w116:dbl[][], "error out"=w230:errorcluster)  [unwired: 10 in]
    n21 = Unbundle By Name(w230) -> ("status"=w355:bool)
    n22 = Divide(x=w419, y="Cal Averaging") -> (x/y=→"Cal Final Sampling Rate":dbl)
    n23 = Divide(x=w419, y=w121) -> (x/y=→"Final Sampling Rate" →"# Samples/channel/s":dbl)
    n24 = case shown="True" w355 {
      frame False {
      }
      frame True {
        n25 = call <vilib>:"Beep.vi"() -> ()  [unwired: 12 in]
        "Buffer Overflow" <- TRUE
      }
    }
    n26 = local read "Buffer size\n(Samples/channel)"() -> (w302:u32)
    n27 = property class="DAQmx Read"(reference=w306) -> (reference out=w305:refnum<k21>, "AvailSampPerChan"=w303:u32)  [unwired: 1 in, 1 out]
    "AvailSampPerChan" <- w303
    n28 = local read "Cal values"() -> (w347:T1)
    n29 = Index Array(array=w116, index (row)=4) -> (element=w219:dbl[])  [unwired: 1 in]
    n30 = Index Array(array=w116, index (row)=0) -> (element=w229:dbl[])  [unwired: 1 in]
    n31 = Index Array(array=w116, index (row)=2) -> (element=w224:dbl[])  [unwired: 1 in]
    n32 = Index Array(array=w116, index (row)=1) -> (element=w228:dbl[])  [unwired: 1 in]
    n33 = Index Array(array=w116, index (row)=3) -> (element=w222:dbl[])  [unwired: 1 in]
    n34 = Index Array(array=w116, index (row)=6) -> (element=w221:dbl[])  [unwired: 1 in]
    n35 = Index Array(array=w116, index (row)=7) -> (element=w220:dbl[])  [unwired: 1 in]
    n36 = Index Array(array=w116, index (row)=5) -> (element=w218:dbl[])  [unwired: 1 in]
    n37 = Divide(x=w303, y=w302) -> (x/y=→"Buffer status":dbl)
    n38 = Unbundle(w347) -> ("AX alpha"=w335:dbl, "BX alpha"=w331:dbl, "AX kappa"=w327:dbl, "BX kappa"=w323:dbl, "AX offset"=w341:dbl, "BX offset"=w339:dbl, "AY alpha"=w338:dbl, "BY alpha"=w333:dbl, "AY kappa"=w329:dbl, "BY kappa"=w325:dbl, "AY offset"=w345:dbl, "BY offset"=w343:dbl)
    n39 = Multiply(x=w228, y=w227) -> (x*y=w223:dbl[])
    n40 = Multiply(x=w229, y=w227) -> (x*y=w225:dbl[])
    n41 = local write "AX alpha"(w335) -> ()
    n42 = local write "BY offset"(w343) -> ()
    n43 = Build Array(w225, w224, w223, w222, w221, w220, w219, w218) -> (w148:dbl[][])
    n44 = local write "BX alpha"(w331) -> ()
    n45 = case shown="True" "Reset data stream" {
      selector: "Reset data stream" -> [_ w466]
      tunnel: w305 -> [w458 w464]
      tunnel: [w458 w462] -> w307
      tunnel: w230 -> [w457 w461]
      tunnel: [w457 w459] -> _
      frame False {
      }
      frame True {
        n46 = Not(x=w466) -> (.not. x?=w465:bool)
        n47 = call <vilib>:"DAQmx Stop Task.vi"("task/channels in"=w464, "error in"=w461) -> ("task out"=w463:refnum<k21>, "error out"=w460:errorcluster)  [unwired: 12 in]
        n48 = local write "Reset data stream"(w465) -> ()
        n49 = local write "Buffer Overflow"(w465) -> ()
        n50 = call <vilib>:"DAQmx Start Task.vi"("task/channels in"=w463, "error in"=w460) -> ("task out"=w462:refnum<k21>, "error out"=w459:errorcluster)  [unwired: 12 in]
      }
    }
    n51 = call-poly <vilib>:"Mean.vi"("X"=w218) -> ("mean"=w361:dbl)  [unwired: 1 out]
    n52 = local write "AY offset"(w345) -> ()
    n53 = call-poly <vilib>:"Mean.vi"("X"=w219) -> ("mean"=w362:dbl)  [unwired: 1 out]
    n54 = call-poly <vilib>:"Mean.vi"("X"=w224) -> ("mean"=w368:dbl)  [unwired: 1 out]
    n55 = call-poly <vilib>:"Mean.vi"("X"=w222) -> ("mean"=w366:dbl)  [unwired: 1 out]
    n56 = call-poly <vilib>:"Mean.vi"("X"=w221) -> ("mean"=w365:dbl)  [unwired: 1 out]
    n57 = call-poly <vilib>:"Mean.vi"("X"=w220) -> ("mean"=w364:dbl)  [unwired: 1 out]
    n58 = local read "Averaging Number"() -> (w114:i32)
    n59 = local write "BY kappa"(w325) -> ()
    n60 = local write "AX kappa"(w327) -> ()
    n61 = call-poly <vilib>:"Mean.vi"("X"=w223) -> ("mean"=w367:dbl)  [unwired: 1 out]
    n62 = local write "AY kappa"(w329) -> ()
    n63 = call-poly <vilib>:"Mean.vi"("X"=w225) -> ("mean"=w369:dbl)  [unwired: 1 out]
    n64 = local read "DAQ rate\n(Samples/s)"() -> (w126:dbl)
    n65 = Build Array(w362, w361) -> (w360:dbl[])
    n66 = local write "BX kappa"(w323) -> ()
    n67 = local write "BY alpha"(w333) -> ()
    n68 = local write "AX offset"(w341) -> ()
    n69 = local write "BX offset"(w339) -> ()
    n70 = local write "AY alpha"(w338) -> ()
    n71 = Build Array(w369, w368, w367, w366, w365, w364) -> (w358:dbl[])
    n72 = Divide(x=w114, y=w126) -> (x/y=w123:dbl)
    "Data update period (s/set)" <- w123
    n73 = Reciprocal(x=w126) -> (1/x=w127:dbl)
    "Data period (s)" <- w127
    n74 = Divide(x=w369, y=w365) -> (x/y=w399:dbl)
    n75 = Divide(x=w368, y=w365) -> (x/y=w400:dbl)
    n76 = Divide(x=w367, y=w364) -> (x/y=w407:dbl)
    n77 = Divide(x=w366, y=w364) -> (x/y=w408:dbl)
    n78 = Subtract(x=w399, y="AY offset") -> (x-y=w381:dbl)
    n79 = Subtract(x=w400, y="AX offset") -> (x-y=w382:dbl)
    n80 = Subtract(x=w407, y="BY offset") -> (x-y=w380:dbl)
    n81 = Subtract(x=w408, y="BX offset") -> (x-y=w383:dbl)
    n82 = Subtract(x=w407, y=w399) -> (x-y=w397:dbl)
    n83 = Subtract(x=w408, y=w400) -> (x-y=w398:dbl)
    n84 = feedback #1(0.0) -> (w301:dbl)
    n85 = Multiply(x="Downsamp\nfact", y=w127) -> (x*y=w128:dbl)
    n86 = Multiply(x=w381, y="AY alpha") -> (x*y=w315:dbl)
    n87 = Multiply(x=w382, y="AX alpha") -> (x*y=w313:dbl)
    n88 = Multiply(x=w383, y="BX alpha") -> (x*y=w314:dbl)
    n89 = Multiply(x=w380, y="BY alpha") -> (x*y=w316:dbl)
    n90 = Add(x=w123, y=w301) -> (x+y=w299:dbl)
    n91 = feedback-in #1(w299) -> ()
    n92 = Square(x=w315) -> (x^2=w391:dbl)
    n93 = Square(x=w313) -> (x^2=w392:dbl)
    n94 = Square(x=w316) -> (x^2=w393:dbl)
    n95 = Square(x=w314) -> (x^2=w394:dbl)
    n96 = Bundle(w397, w398) -> (w117:cluster{dbl, dbl})  [unwired: 1 in]
    n97 = case shown="True" "Set reading to\nsetpoint" {
      tunnel: w117 -> [_ w455]
      frame False {
      }
      frame True {
        n98 = local write "Set reading to\nsetpoint"(FALSE ("Set reading to\nsetpoint")) -> ()
        n99 = local read "Trap position"() -> (w454:cluster{"X":dbl, "Y":dbl})
        n100 = property on="Setpoint voltage" class="Clust (strict)"("Val(Sgnl)"=w455) -> ()  [unwired: 2 in, 2 out]
        n101 = Unbundle(w454) -> ("X"=w453:dbl, "Y"=w452:dbl)
        n102 = Bundle("Y"=w452, "X"=w453) -> (w451:cluster{"Y":dbl, "X":dbl})  [unwired: 1 in]
        n103 = property on="Offset" class="Clust (strict)"("Val(Sgnl)"=w451) -> ()  [unwired: 2 in, 2 out]
      }
    }
    n104 = Reciprocal(x=w128) -> (1/x=→"Chart Freq (Hz)":dbl)
    n105 = To Time Stamp(1:w299) -> (0:w298:timestamp)
    n106 = Add(x=w391, y=w392) -> (x+y=w395:dbl)
    n107 = Add(x=w393, y=w394) -> (x+y=w406:dbl)
    n108 = Multiply(x=w313, y="AX kappa") -> (x*y=w309:dbl)
    n109 = Bundle("A y", "A x", "B y", "B x", "A sum", "B sum", "Trap x", "Trap y") -> (w289:T11)  [unwired: 1 in]
    n110 = Multiply(x=w314, y="BX kappa") -> (x*y=w310:dbl)
    n111 = Square Root(x=w395) -> (sqrt(x)=w411:dbl)
    n112 = Square Root(x=w406) -> (sqrt(x)=w410:dbl)
    n113 = Multiply(x=w315, y="AY kappa") -> (x*y=w311:dbl)
    n114 = Multiply(x=w316, y="BY kappa") -> (x*y=w312:dbl)
    n115 = Subtract(x=w361, y="Fixed Y") -> (x-y=w396:dbl)
    n116 = Subtract(x=w362, y="Fixed X") -> (x-y=w401:dbl)
    n117 = Cluster To Array(cluster=w289) -> (array=w288:string[])
    n118 = for {
      tunnel: w148 -> [w443] mode=indexing
      tunnel: w128 -> [_]
      tunnel: "Downsamp\nfact" -> [w448]
      tunnel: [w446] -> w204 mode=indexing
      tunnel: w298 -> [w450]
      tunnel: w288 -> [w445] mode=indexing
      tunnel: "NI_ChannelName" ("name") -> [w444]
      n119 = call "Downsample 1D array.vi"("Ave N"=w448, "Arrray In"=w443) -> ("Array Out"=w449:dbl[])  [unwired: 9 in]
      n120 = Bundle By Name("Y"=w449, "dt"="dt", "t0"=w450) -> (w447:waveform(dbl))  [unwired: 1 in]
      n121 = Set Waveform Attribute(5:w445, 6:w444, 7:w447) -> (3:w446:waveform(dbl))  [unwired: 1 in, 2 out]
    }
    "All signals" <- w204
    n122 = Square(x=w311) -> (x^2=w384:dbl)
    n123 = Square(x=w309) -> (x^2=w385:dbl)
    n124 = Square(x=w312) -> (x^2=w386:dbl)
    n125 = Square(x=w310) -> (x^2=w387:dbl)
    n126 = Add(x=w384, y=w385) -> (x+y=w388:dbl)
    n127 = Add(x=w386, y=w387) -> (x+y=w389:dbl)
    n128 = Multiply(x=w396, y="Conv Y (nm/V)") -> (x*y=w318:dbl)
    n129 = Multiply(x=w401, y="Conv X (nm/V)") -> (x*y=w319:dbl)
    n130 = feedback #2() -> (w356:cluster{"B_Y":dbl, "B_X":dbl})  [unwired: 1 in]
    n131 = case shown="True" "Force Feedback" {
      tunnel: [w746 w762] -> w415
      tunnel: [w745 w761] -> w423
      tunnel: w117 -> [_ w760]
      tunnel: [cluster{"B_Y":dbl, "B_X":dbl} {"B_Y"=0.0, "B_X"=0.0} ("Sum error past") w752] -> w357
      tunnel: w356 -> [_ w759]
      tunnel: w416 -> [w746 w755]
      tunnel: w421 -> [w745 w754]
      frame False {
        # "Force feedback"
      }
      frame True {
        n132 = call "ForceFeedback2.vi"("PSD/Mirror Voltages"=w760, "Sum error"=w759, "task/channels in"=w755, "error in"=w754, "Desired voltage"="Setpoint voltage", "Feedback const"="Feedback const", "offset"="Offset") -> ("task out"=w762:refnum<k21>, "Sum error past"=w752:cluster{"B_Y":dbl, "B_X":dbl}, "Output Voltage"=→"Feedback Output Voltage 2":cluster{dbl, dbl}, "error out"=w761:errorcluster)  [unwired: 8 in, 1 out]
        n133 = local read "Pulling direction"() -> (w751:bool)
        n134 = Unbundle(w752) -> ("B_Y"=w749:dbl, "B_X"=w748:dbl)
        n135 = Select(t=w749, s=w751, f=w748) -> (s? t:f=→"Sum error":dbl)
      }
    }
    n136 = feedback-in #2(w357) -> ()
    n137 = Square Root(x=w388) -> (sqrt(x)=w317:dbl)
    n138 = Square Root(x=w389) -> (sqrt(x)=w412:dbl)
    n139 = Add(x=w317, y=w412) -> (x+y=w390:dbl)
    n140 = Build Array(w399, w400, w407, w408, w365, w364, w317, w412, w411, w410, w319, w318) -> ()  [unwired: 1 out]
    n141 = Divide(x=w390, y=2.0) -> (x/y=w354:dbl)
    n142 = Index Array(array=w204, index=6) -> (element=w153:waveform(dbl))
    n143 = Index Array(array=w204, index=7) -> (element=w155:waveform(dbl))
    n144 = local read "Fixed X"() -> (w208:dbl)
    n145 = local read "Fixed Y"() -> (w210:dbl)
    n146 = Unbundle By Name(w153) -> ("Y"=w212:dbl[])
    n147 = Unbundle By Name(w155) -> ("Y"=w211:dbl[])
    n148 = Index Array(array=w204, index=0) -> (element=w161:waveform(dbl))
    n149 = Index Array(array=w204, index=1) -> (element=w285:waveform(dbl))
    n150 = Index Array(array=w204, index=4) -> (element=w279:waveform(dbl))
    n151 = Subtract(x=w212, y=w208) -> (x-y=w209:dbl[])
    n152 = Subtract(x=w211, y=w210) -> (x-y=w206:dbl[])
    n153 = Unbundle By Name(w161) -> ("Y"=w277:dbl[])
    n154 = Unbundle By Name(w285) -> ("Y"=w276:dbl[])
    n155 = Unbundle By Name(w279) -> ("Y"=w275:dbl[])
    n156 = Index Array(array=w204, index=5) -> (element=w278:waveform(dbl))
    n157 = local read "Conv X (nm/V)"() -> (w207:dbl)
    n158 = local read "Conv Y (nm/V)"() -> (w205:dbl)
    n159 = Index Array(array=w204, index=2) -> (element=w158:waveform(dbl))
    n160 = Index Array(array=w204, index=3) -> (element=w282:waveform(dbl))
    n161 = Set Waveform Attribute(5:"T2 X", 6:w151, 7:w153) -> (3:w152:waveform(dbl))  [unwired: 1 in, 2 out]
    n162 = Set Waveform Attribute(5:"T2 Y", 6:w151, 7:w155) -> (3:w154:waveform(dbl))  [unwired: 1 in, 2 out]
    n163 = Unbundle By Name(w278) -> ("Y"=w272:dbl[])
    n164 = Unbundle By Name(w158) -> ("Y"=w274:dbl[])
    n165 = Unbundle By Name(w282) -> ("Y"=w273:dbl[])
    n166 = local read "Saving"() -> (w320:bool)
    n167 = local read "Tether"() -> (w321:bool)
    n168 = Divide(x=w277, y=w275) -> (x/y=w176:dbl[])
    n169 = Divide(x=w276, y=w275) -> (x/y=w174:dbl[])
    n170 = local read "AY offset"() -> (w263:dbl)
    n171 = local read "AX offset"() -> (w261:dbl)
    n172 = Multiply(x=w209, y=w207) -> (x*y=w145:dbl[])
    n173 = Multiply(x=w206, y=w205) -> (x*y=w147:dbl[])
    n174 = Less?(x=w354, y="Tether break\nforce (pN)") -> (x < y?=w352:bool)
    n175 = Divide(x=w273, y=w272) -> (x/y=w175:dbl[])
    n176 = Subtract(x=w174, y=w261) -> (x-y=w264:dbl[])
    n177 = local read "BY offset"() -> (w268:dbl)
    n178 = local read "BX offset"() -> (w271:dbl)
    n179 = Subtract(x=w176, y=w263) -> (x-y=w265:dbl[])
    n180 = Divide(x=w274, y=w272) -> (x/y=w177:dbl[])
    n181 = local read "AY alpha"() -> (w262:dbl)
    n182 = local read "AX alpha"() -> (w260:dbl)
    n183 = Compound Arithmetic op=AND(w320, w321, w352) -> (w351:bool)
    n184 = call-poly <vilib>:"Mean.vi"("X"=w147) -> ("mean"=w187:dbl)  [unwired: 1 out]
    "Mean Trp Pos Y 2 (nm)" <- w187
    n185 = Subtract(x=w177, y=w176) -> (x-y=w173:dbl[])
    n186 = Subtract(x=w175, y=w174) -> (x-y=w172:dbl[])
    n187 = Subtract(x=w145, y="Offset X (nm)") -> (x-y=w144:dbl[])
    n188 = Subtract(x=w147, y="Offset Y (nm)") -> (x-y=w146:dbl[])
    n189 = Subtract(x=w177, y=w268) -> (x-y=w270:dbl[])
    n190 = Subtract(x=w175, y=w271) -> (x-y=w269:dbl[])
    n191 = Subtract(x=w187, y=w147) -> (x-y=w186:dbl[])
    n192 = call-poly <vilib>:"Mean.vi"("X"=w145) -> ("mean"=w191:dbl)  [unwired: 1 out]
    "Mean Trap Pos X 2 (nm)" <- w191
    n193 = Build Array(w173, w172) -> (w170:dbl[][])
    n194 = Index Array(array=w170, index (row)=0) -> (element=w168:dbl[])  [unwired: 1 in]
    n195 = Index Array(array=w170, index (row)=1) -> (element=w167:dbl[])  [unwired: 1 in]
    n196 = call-poly <vilib>:"Mean.vi"("X"=w168) -> ("mean"=w166:dbl)  [unwired: 1 out]
    n197 = call-poly <vilib>:"Mean.vi"("X"=w167) -> ("mean"=w165:dbl)  [unwired: 1 out]
    n198 = Bundle("mean"=w166, "mean"=w165) -> ()  [unwired: 1 in, 1 out]
    n199 = local read "BY alpha"() -> (w267:dbl)
    n200 = local read "BX alpha"() -> (w266:dbl)
    n201 = Multiply(x=w265, y=w262) -> (x*y=w253:dbl[])
    n202 = Multiply(x=w264, y=w260) -> (x*y=w252:dbl[])
    n203 = Square(x=w186) -> (x^2=w185:dbl[])
    n204 = Subtract(x=w191, y=w145) -> (x-y=w190:dbl[])
    n205 = Bundle By Name(cluster=w154, "Y"=w146) -> (w202:waveform(dbl))
    n206 = case shown="True" w351 {
      selector: w351 -> [_ w469]
      frame False {
      }
      frame True {
        n207 = call <vilib>:"Beep.vi"() -> ()  [unwired: 12 in]
        n208 = Not(x=w469) -> (.not. x?=w467:bool)
        n209 = local write "Tether"(w467) -> ()
        n210 = local write "Force Feedback"(w467) -> ()
        n211 = property on="Stop saving" class="Bool (strict)"("Val(Sgnl)"="TA Cancel Save?") -> ()  [unwired: 2 in, 2 out]
      }
    }
    n212 = Bundle By Name(cluster=w152, "Y"=w144) -> (w203:waveform(dbl))
    n213 = Square(x=w190) -> (x^2=w189:dbl[])
    n214 = call-poly <vilib>:"Mean.vi"("X"=w185) -> ("mean"=w184:dbl)  [unwired: 1 out]
    n215 = Square(x=w253) -> (x^2=w259:dbl[])
    n216 = Multiply(x=w270, y=w267) -> (x*y=w251:dbl[])
    n217 = Square(x=w252) -> (x^2=w258:dbl[])
    n218 = Multiply(x=w269, y=w266) -> (x*y=w250:dbl[])
    n219 = call-poly <vilib>:"Mean.vi"("X"=w189) -> ("mean"=w188:dbl)  [unwired: 1 out]
    n220 = Build Array(w203, w202) -> (w108:waveform(dbl)[])
    "Trap sep" <- w108
    n221 = local read "Flushing Sample"() -> (w113:bool)
    n222 = Square Root(x=w184) -> (sqrt(x)=w183:dbl)
    n223 = Square(x=w251) -> (x^2=w257:dbl[])
    n224 = Square(x=w250) -> (x^2=w256:dbl[])
    n225 = Add(x=w259, y=w258) -> (x+y=w255:dbl[])
    n226 = Square Root(x=w188) -> (sqrt(x)=w181:dbl)
    n227 = Multiply(x=w183, y=10) -> (x*y=→"T2 Y RMS (A)":dbl)
    n228 = Square Root(x=w255) -> (sqrt(x)=w140:dbl[])
    n229 = Add(x=w257, y=w256) -> (x+y=w254:dbl[])
    n230 = Set Waveform Attribute(5:"T2", 6:"NI_ChannelName" ("name"), 7:w161) -> (3:w160:waveform(dbl))  [unwired: 1 in, 2 out]
    n231 = Set Waveform Attribute(5:"T1", 6:"NI_ChannelName" ("name"), 7:w158) -> (3:w157:waveform(dbl))  [unwired: 1 in, 2 out]
    n232 = Square Root(x=w254) -> (sqrt(x)=w139:dbl[])
    n233 = Multiply(x=w181, y=10) -> (x*y=→"T2 X RMS (A)":dbl)
    n234 = Bundle By Name(cluster=w160, "Y"=w140) -> (w164:waveform(dbl))
    n235 = case shown="True" w113 {
      frame False {
      }
      frame True {
        n236 = local read "Flush Sample Start Time"() -> (w434:u32)
        n237 = local read "Sample flush time (s)"() -> (w427:dbl)
        n238 = Tick Count (ms)() -> (millisecond timer value=w435:u32)
        n239 = Subtract(x=w435, y=w434) -> (x-y=w425:u32)
        n240 = Multiply(x=u32 1000, y=w427) -> (x*y=w426:dbl)
        n241 = Divide(x=w425, y=w426) -> (x/y=w430:dbl)
        n242 = Greater?(x=w425, y=w426) -> (0:w433:bool)
        n243 = Not(x=w433) -> (.not. x?=w432:bool)
        n244 = Boolean To (0,1)(Boolean=w432) -> (0, 1=w431:i16)
        n245 = Compound Arithmetic op=MULTIPLY(w431, w430, 100.0 ("value")) -> (→"Sample Flush Meter":dbl)
        n246 = case shown="True" w433 {
          frame False {
          }
          frame True {
            w437 = FALSE ("Inject Sample")
            n247 = property on="Clear Volume" class="Bool (strict)"("Val(Sgnl)"=TRUE ("Value (Signaling)")) -> ()  [unwired: 2 in, 2 out]
            n248 = local write "Inject Sample"(w437) -> ()
            n249 = local write "Flushing Sample"(w437) -> ()
          }
        }
      }
    }
    n250 = Bundle By Name(cluster=w157, "Y"=w139) -> (w232:waveform(dbl))
    n251 = Add(x=w140, y=w139) -> (x+y=w138:dbl[])
    n252 = case shown="True" "Remove offsets" {
      selector: "Remove offsets" -> [_ w440]
      frame False {
      }
      frame True {
        n253 = local read "Mean Trp Pos Y 2 (nm)"() -> (w438:dbl)
        n254 = Not(x=w440) -> (.not. x?=w441:bool)
        n255 = local read "Mean Trap Pos X 2 (nm)"() -> (w439:dbl)
        n256 = local write "Remove offsets"(w441) -> ()
        n257 = local write "Offset Y (nm)"(w438) -> ()
        n258 = local write "Offset X (nm)"(w439) -> ()
      }
    }
    n259 = Build Array(w164, w232) -> (→"Bead sep":waveform(dbl)[])
    n260 = local read "AY kappa"() -> (w249:dbl)
    n261 = local read "AX kappa"() -> (w248:dbl)
    n262 = Divide(x=w138, y=2) -> (x/y=w136:dbl[])
    n263 = local read "BX kappa"() -> (w246:dbl)
    n264 = local read "BY kappa"() -> (w247:dbl)
    n265 = call-poly <vilib>:"Mean.vi"("X"=w136) -> ("mean"=w135:dbl)  [unwired: 1 out]
    "Mean Bead Sep\n(nm)" <- w135
    n266 = local read "Calibrating"() -> (w413:bool)
    n267 = Multiply(x=w253, y=w249) -> (x*y=w242:dbl[])
    n268 = Multiply(x=w252, y=w248) -> (x*y=w243:dbl[])
    n269 = Square(x=w242) -> (x^2=w241:dbl[])
    n270 = Square(x=w243) -> (x^2=w240:dbl[])
    n271 = Subtract(x=w136, y=w135) -> (x-y=w134:dbl[])
    n272 = Multiply(x=w251, y=w247) -> (x*y=w244:dbl[])
    n273 = Multiply(x=w250, y=w246) -> (x*y=w245:dbl[])
    n274 = Add(x=w241, y=w240) -> (x+y=w237:dbl[])
    n275 = Square(x=w134) -> (x^2=w133:dbl[])
    n276 = Square Root(x=w237) -> (sqrt(x)=w201:dbl[])
    n277 = Square(x=w244) -> (x^2=w239:dbl[])
    n278 = Square(x=w245) -> (x^2=w238:dbl[])
    n279 = call-poly <vilib>:"Mean.vi"("X"=w133) -> ("mean"=w132:dbl)  [unwired: 1 out]
    n280 = Add(x=w239, y=w238) -> (x+y=w236:dbl[])
    n281 = Bundle By Name(cluster=w160, "Y"=w201) -> (w235:waveform(dbl))
    n282 = local read "Saving"() -> (w350:bool)
    n283 = Or(x=w413, y=w350) -> ()  [unwired: 1 out]
    n284 = Square Root(x=w132) -> (sqrt(x)=w131:dbl)
    n285 = Square Root(x=w236) -> (sqrt(x)=w200:dbl[])
    n286 = And(x="Save scans", y="Raster scan") -> (x .and. y?=w111:bool)
    n287 = Multiply(x=10, y=w131) -> (x*y=→"Bead Sep Noise\n(A)":dbl)
    n288 = Bundle By Name(cluster=w157, "Y"=w200) -> (w234:waveform(dbl))
    n289 = Add(x=w201, y=w200) -> (x+y=w199:dbl[])
    n290 = Build Array(w235, w234) -> (→"Force (pN)":waveform(dbl)[])
    n291 = flat-sequence {
      tunnel: w413 -> [w507]
      tunnel: w350 -> [_]
      tunnel: w413 -> [_]
      tunnel: w350 -> [_]
      tunnel: w148 -> [w491]
      tunnel: [w491] -> w371
      tunnel: w230 -> [w490]
      tunnel: [w490] -> w370
      tunnel: w358 -> [w489]
      tunnel: [w489] -> w363
      tunnel: w360 -> [w488]
      tunnel: [w488] -> w359
      tunnel: [w485] -> w349
      tunnel: [w482] -> w348
      tunnel: [w479] -> w217
      tunnel: [w478] -> w216
      tunnel: [w475] -> w215
      tunnel: w111 -> [w472]
      tunnel: ["Save Data"] -> w109
      tunnel: w371 -> [w658]
      tunnel: w370 -> [w657]
      tunnel: w363 -> [_]
      tunnel: w359 -> [_]
      tunnel: w349 -> [w656]
      tunnel: w348 -> [w655]
      tunnel: w217 -> [w654]
      tunnel: w216 -> [w653]
      tunnel: w215 -> [w652]
      tunnel: w109 -> [w650]
      tunnel: w108 -> [w649]
      frame #0 {
        w502 = 0.0
        # "1: old trap\n0: fleezers"
        # "Create files if saving data"
        n292 = local read "Save N sets"() -> (w474:bool)
        n293 = local read "Sampling Rate"() -> (w505:dbl)
        n294 = Or(x=w474, y="Save Data") -> (x .or. y?=w473:bool)
        n295 = Build Array(w473, "Save cal", w472) -> (w493:bool[])
        n296 = Compound Arithmetic op=OR("Save Data", "Save cal", w472) -> (w495:bool)
        n297 = Boolean Array To Number(Boolean array=w493) -> (number=w492:u32)
        n298 = local read "Trap position"() -> (w501:cluster{"X":dbl, "Y":dbl})
        n299 = Unbundle(w501) -> ("X"=w499:dbl, "Y"=w500:dbl)
        n300 = Build Array(w502, w502, w500, w499, w502, w502) -> (w498:dbl[])
        n301 = feedback #3(refnum<k0> refnum) -> (w483:refnum<file>)
        n302 = feedback #4() -> (w480:dbl)  [unwired: 1 in]
        n303 = feedback #5(FALSE) -> (w476:bool)
        n304 = feedback #6(0) -> (w496:i32)
        n305 = feedback #7(refnum<k0> refnum) -> (w486:refnum<file>)
        n306 = case shown="True" w495 {
          tunnel: w507 -> [_ _]
          tunnel: 9 -> [_ w549]
          tunnel: w505 -> [_ w548]
          tunnel: 6 -> [_ w547]
          tunnel: 5 -> [_ w546]
          tunnel: w498 -> [_ w545]
          tunnel: [w512 1] -> w479
          tunnel: w496 -> [w513 _]
          tunnel: w492 -> [_ w520]
          tunnel: [w511 w518] -> w485
          tunnel: w486 -> [w511 _]
          tunnel: [w510 w517] -> w482
          tunnel: w483 -> [w510 _]
          tunnel: 1.0 -> [_ w516]
          tunnel: [w509 w515] -> w478
          tunnel: w480 -> [w509 _]
          tunnel: [w508 w514] -> w475
          tunnel: w476 -> [w508 _]
          frame False {
            n307 = Increment(x=w513) -> (x+1=w512:i32)
          }
          frame True {
            w521 = FALSE ("Save Data")
            w527 = FALSE
            w528 = T10."big-endian, network order" ("byte order (0:big-endian, network order)")
            n308 = local write "Save cal"(w521) -> ()
            n309 = local write "Save Data"(w521) -> ()
            n310 = case shown="4" w520 {
              tunnel: w549 -> [w595 w613 w648]
              tunnel: w548 -> [w594 w612 w647]
              tunnel: w547 -> [w593 w610 w643]
              tunnel: w546 -> [w592 w609 w642]
              tunnel: w545 -> [w590 w606 w639]
              tunnel: [w589 w605 w625] -> w542
              tunnel: [w591 w602 w624] -> w514
              tunnel: ["Averaging Number" 200 w622] -> _
              tunnel: w516 -> [w577 w597 w621]
              tunnel: [w573 "Cal sets to save" w616] -> w515
              frame 1, Default {
                w591 = TRUE
                w578 = 0.0
                # "Time trace"
                n311 = local read "Averaging Number"() -> (w588:i32)
                n312 = Boolean To (0,1)(Boolean=w591) -> (0, 1=w583:i16)
                n313 = Increment(x=w583) -> (x+1=w582:i16)
                n314 = Divide(x=w594, y=w588) -> (x/y=w587:dbl)
                n315 = To Double Precision Float(number=w582) -> (double precision float=w581:dbl)
                n316 = Reciprocal(x=w587) -> (1/x=w586:dbl)
                n317 = Build Array(w595, w594, w586, w593, w592, 0 ("f")) -> (w585:dbl[])
                n318 = Build Array(w581, w577, w578, w578, w578) -> (w584:dbl[])
                n319 = Build Array (concatenate)(w585, w590, w584) -> (w589:dbl[])
                n320 = Select(t="N sets", s="Save N sets", f=2147483647) -> (s? t:f=w573:i32)
              }
              frame 2 {
                w602 = FALSE
                w600 = 0.0
                # "Calibration file"
                n321 = Reciprocal(x=w612) -> (1/x=w611:dbl)
                n322 = Boolean To (0,1)(Boolean=w602) -> (0, 1=w604:i16)
                n323 = To Double Precision Float(number=w604) -> (double precision float=w603:dbl)
                n324 = Build Array(w613, w611, w611, w610, w609, 1) -> (w607:dbl[])
                n325 = Build Array(w603, w597, w600, w600, w600) -> (w601:dbl[])
                n326 = Build Array (concatenate)(w607, w606, w601) -> (w605:dbl[])
                "Calibrating" <- TRUE ("Calibrating")
              }
              frame 4 {
                w623 = 0
                w635 = 0.0
                w624 = TRUE
                # "Not using nsteps yet"
                # "FX curve"
                n327 = local read "Averaging Number"() -> (w646:i32)
                n328 = Boolean To (0,1)(Boolean=w624) -> (0, 1=w638:i16)
                n329 = Increment(x=w638) -> (x+1=w637:i16)
                n330 = local write "Raster scan"(FALSE ("Raster scan")) -> ()
                n331 = To Double Precision Float(number=w637) -> (double precision float=w636:dbl)
                n332 = Divide(x=w647, y=w646) -> (x/y=w645:dbl)
                n333 = Reciprocal(x=w645) -> (1/x=w644:dbl)
                n334 = Build Array(w636, w621, w635, w635, w635) -> (w634:dbl[])
                n335 = Build Array(w648, w647, w644, w643, w642, 2) -> (w640:dbl[])
                n336 = local read "Data update period (s/set)"() -> (w619:dbl)
                n337 = local read "Pulling direction"() -> (w632:bool)
                n338 = local read "Max delta"() -> (w630:dbl)
                n339 = local read "Min delta"() -> (w629:dbl)
                n340 = local read "# scans"() -> (w627:i32)
                n341 = local read "Speed (ms)"() -> (w620:i32)
                n342 = Subtract(x=w630, y=w629) -> (x-y=w628:dbl)
                n343 = Not(x=w632) -> (.not. x?=w631:bool)
                n344 = local read "Averaging Number"() -> (w622:i32)
                n345 = Boolean To (0,1)(Boolean=w631) -> (0, 1=w633:i16)
                n346 = Multiply(x=750.0, y=w619) -> (x*y=w617:dbl)
                n347 = Build Array(w633, w628, w623, w623, w627) -> (w626:dbl[])
                n348 = Divide(x=w620, y=w617) -> (x/y=w615:dbl)
                n349 = Build Array (concatenate)(w640, w639, w634, w626) -> (w625:dbl[])
                n350 = Round Toward +Infinity(x=w615) -> (ceil(x): smallest int >= x=w616:dbl)
              }
            }
            n351 = call "CreateSaveFile.vi"("Index In"="Save file index", "Ext"=".dat", "Insert"="", "Directory"="Path") -> ("Path Out"=w526:path)  [unwired: 6 in, 1 out]
            "Current file name" <- w526
            n352 = Open/Create/Replace File(file path (use dialog)=w526, operation (0:open)=T9."create", access (0:read/write)=enum16{"read/write", "read-only", "write-only"}."write-only") -> (refnum out=w535:refnum<file>, error out=w536:errorcluster)  [unwired: 3 in, 1 out]
            n353 = Array Size(array=w542) -> (size(s)=w544:i32)
            n354 = case shown="True" w514 {
              tunnel: w526 -> [_ w572]
              tunnel: [refnum<k0> refnum w551] -> w517
              frame False {
              }
              frame True {
                w558 = 0.0
                n355 = Path To String(path=w572) -> (string=w568:string)
                n356 = Build Array(w558, w558, w558, w558, w558, w558, w558, w558) -> (w555:dbl[])
                n357 = String Length(string=w568) -> (length=w571:i32)
                n358 = Array Size(array=w555) -> (size(s)=w557:i32)
                n359 = Subtract(x=w571, y=4) -> (x-y=w569:i32)
                n360 = To Double Precision Float(number=w557) -> (double precision float=w556:dbl)
                n361 = String Subset(string=w568, length (rest)=w569) -> (substring=w567:string)  [unwired: 1 in]
                n362 = Build Array (concatenate)(w556, w555) -> (w554:dbl[])
                n363 = Concatenate Strings(w567, "_pos.dat" ("string")) -> (w565:string)
                n364 = String To Path(string=w565) -> (path=w564:path)
                n365 = Open/Create/Replace File(file path (use dialog)=w564, operation (0:open)=T9."create", access (0:read/write)=enum16{"read/write", "read-only", "write-only"}."write-only") -> (refnum out=w560:refnum<file>, error out=w561:errorcluster)  [unwired: 3 in, 1 out]
                n366 = Deny Access(4:w561, 7:w560) -> (3:w559:refnum<file>)  [unwired: 1 in, 1 out]
                n367 = Write to Binary File(file (use dialog)=w559, data=w554, 5:FALSE ("prepend array or string size? (T)"), 9:T10."big-endian, network order" ("byte order (0:big-endian, network order)")) -> (refnum out=w551:refnum<file>)  [unwired: 2 in, 2 out]
              }
            }
            n368 = Deny Access(4:w536, 7:w535) -> (0:w525:errorcluster, 3:w534:refnum<file>)  [unwired: 1 in]
            n369 = String Length(string="Comment") -> (length=w541:i32)
            n370 = To Double Precision Float(number=w544) -> (double precision float=w543:dbl)
            n371 = To Double Precision Float(number=w541) -> (double precision float=w540:dbl)
            n372 = Build Array (concatenate)(w543, w542, w540) -> (w531:dbl[])
            n373 = Write to Binary File(file (use dialog)=w534, data=w531, error in=w525, 5:w527, 9:w528) -> (refnum out=w530:refnum<file>, error out=w524:errorcluster)  [unwired: 1 in, 1 out]
            n374 = Write to Binary File(file (use dialog)=w530, data="Comment", error in=w524, 5:w527, 9:w528) -> (refnum out=w518:refnum<file>)  [unwired: 1 in, 2 out]
            "Saving" <- TRUE
          }
        }
        n375 = feedback-in #3(w482) -> ()
        n376 = feedback-in #4(w478) -> ()
        n377 = feedback-in #5(w475) -> ()
        n378 = feedback-in #6(w479) -> ()
        n379 = feedback-in #7(w485) -> ()
      }
      frame #1 {
        n380 = local read "Saving"() -> (w651:bool)
        n381 = case shown="True" w651 {
          tunnel: w658 -> [_ w677]
          tunnel: w657 -> [_ w676]
          tunnel: w656 -> [_ w675]
          tunnel: w655 -> [_ w674]
          tunnel: w654 -> [_ w664]
          tunnel: w653 -> [_ w665]
          tunnel: w652 -> [_ w668]
          tunnel: w650 -> [_ w660]
          tunnel: w649 -> [_ w659]
          frame False {
            (unwired) FALSE ("Calibrating")
          }
          frame True {
            n382 = local read "Stop"() -> (w672:bool)
            n383 = Less Or Equal?(x=w664, y=w665) -> (x <= y?=w673:bool)
            n384 = Divide(x=w664, y=w665) -> (x/y=w663:dbl)
            n385 = Or(x=w672, y="Stop saving") -> (x .or. y?=w671:bool)
            n386 = Not(x=w671) -> (.not. x?=w670:bool)
            n387 = Multiply(x=100.0, y=w663) -> (x*y=w662:dbl)
            n388 = And(x=w673, y=w670) -> (x .and. y?=w669:bool)
            n389 = case shown="True" w669 {
              tunnel: w675 -> [w682 w691]
              tunnel: w676 -> [_ w690]
              tunnel: w677 -> [_ w689]
              tunnel: w674 -> [w681 w688]
              tunnel: w668 -> [w679 _]
              tunnel: [0.0 ("Progress") w687] -> w667
              tunnel: w662 -> [_ w687]
              tunnel: w660 -> [_ w684]
              tunnel: w659 -> [_ w685]
              frame False {
                w680 = FALSE
                n390 = Close File(refnum=w682) -> ()  [unwired: 1 in, 2 out]
                n391 = case shown="True" w679 {
                  tunnel: w681 -> [_ w683]
                  frame False {
                  }
                  frame True {
                    n392 = Close File(refnum=w683) -> ()  [unwired: 1 in, 2 out]
                  }
                }
                n393 = call <vilib>:"Beep.vi"() -> ()  [unwired: 12 in]
                n394 = local write "Saving"(w680) -> ()
                n395 = local write "Stop saving"(w680) -> ()
                n396 = local write "Calibrating"(w680) -> ()
              }
              frame True {
                n397 = local read "Calibrating"() -> (w686:bool)
                n398 = case shown="False" w686 {
                  tunnel: w691 -> [w728 w744]
                  tunnel: w690 -> [_ w743]
                  tunnel: w689 -> [w715 w737]
                  tunnel: w688 -> [w714 _]
                  tunnel: w685 -> [w706 _]
                  tunnel: w684 -> [w698 _]
                  frame False {
                    n399 = local read "Averaging Number"() -> (w722:i32)
                    n400 = Array Subset(array=w715, index (row)=0 ("index"), length (row)=6 ("length")) -> (w711:dbl[][])  [unwired: 2 in]
                    n401 = Array Subset(array=w715, index (row)=6 ("index"), length (row)=2 ("length")) -> (w710:dbl[][])  [unwired: 2 in]
                    n402 = Array Size(array=w710) -> (size(s)=w721:i32[])
                    n403 = Array Size(array=w711) -> (size(s)=w718:i32[])
                    n404 = Index Array(array=w706, index=0) -> (element=w703:waveform(dbl))
                    n405 = Index Array(array=w706, index=1) -> (element=w702:waveform(dbl))
                    n406 = for {
                      tunnel: w711 -> [w732] mode=indexing
                      tunnel: w722 -> [w734]
                      tunnel: [w733] -> w709 mode=indexing
                      n407 = call "Downsample 1D array.vi"("Ave N"=w734, "Arrray In"=w732) -> ("Array Out"=w733:dbl[])  [unwired: 9 in]
                    }
                    n408 = Unbundle By Name(w703) -> ("Y"=w701:dbl[])
                    n409 = Unbundle By Name(w702) -> ("Y"=w697:dbl[])
                    n410 = Multiply Array Elements(1:w718) -> (0:w717:i32)
                    n411 = for {
                      tunnel: w710 -> [w731] mode=indexing
                      tunnel: w722 -> [w730]
                      tunnel: [w729] -> w713 mode=indexing
                      n412 = call "Downsample 1D array.vi"("Ave N"=w730, "Arrray In"=w731) -> ("Array Out"=w729:dbl[])  [unwired: 9 in]
                    }
                    n413 = Multiply Array Elements(1:w721) -> (0:w720:i32)
                    n414 = feedback #8(w701) -> (w700:dbl[])
                    n415 = Build Array (concatenate)(w700, w701) -> (w699:dbl[])
                    n416 = Select(t=w701, s=w698, f=w699) -> (s? t:f=w694:dbl[])
                    n417 = feedback-in #8(w694) -> ()
                    n418 = feedback #9(w697) -> (w696:dbl[])
                    n419 = Build Array (concatenate)(w696, w697) -> (w695:dbl[])
                    n420 = Select(t=w697, s=w698, f=w695) -> (s? t:f=w693:dbl[])
                    n421 = feedback-in #9(w693) -> ()
                    n422 = Divide(x=w717, y=w722) -> (x/y=w723:dbl)
                    n423 = Divide(x=w720, y=w722) -> (x/y=w719:dbl)
                    n424 = Transpose 2D Array(2D array=w709) -> (transposed array=w708:dbl[][])
                    n425 = Build Array(w694, w693) -> (→"Saved Trap Pos":dbl[][])
                    n426 = Transpose 2D Array(2D array=w713) -> (transposed array=w707:dbl[][])
                    "Waveform Chart 3" <- w707
                    n427 = Reshape Array(w708, w723) -> (w712:dbl[])
                    n428 = Reshape Array(w707, w719) -> (w716:dbl[])
                    n429 = call <vilib>:"Write File+ [SGL].vi"("1D array"=w716, "refnum"=w714) -> ()  [unwired: 7 in, 3 out]
                    n430 = call <vilib>:"Write File+ [SGL].vi"("1D array"=w712, "refnum"=w728) -> ()  [unwired: 7 in, 3 out]
                  }
                  frame True {
                    n431 = Array Subset(array=w737, index (row)=0 ("index"), length (row)=6 ("length")) -> (w735:dbl[][])  [unwired: 2 in]
                    n432 = Transpose 2D Array(2D array=w735) -> (transposed array=w741:dbl[][])
                    n433 = Array Size(array=w735) -> (size(s)=w736:i32[])
                    n434 = Multiply Array Elements(1:w736) -> (0:w742:i32)
                    n435 = Reshape Array(w741, w742) -> (w740:dbl[])
                    n436 = call <vilib>:"Write File+ [SGL].vi"("1D array"=w740, "error in (no error)"=w743, "refnum"=w744) -> ()  [unwired: 6 in, 3 out]
                  }
                }
              }
            }
            "Progress" <- w667
          }
        }
      }
    }
    n437 = Divide(x=w199, y=2) -> (x/y=w196:dbl[])
    n438 = call-poly <vilib>:"Mean.vi"("X"=w196) -> ("mean"=w197:dbl)  [unwired: 1 out]
    "Mean force (pN)" <- w197
    n439 = Subtract(x=w197, y=w196) -> (x-y=w195:dbl[])
    n440 = Square(x=w195) -> (x^2=w194:dbl[])
    n441 = call-poly <vilib>:"Mean.vi"("X"=w194) -> ("mean"=w193:dbl)  [unwired: 1 out]
    n442 = Square Root(x=w193) -> (sqrt(x)=→"Force noise (pN)":dbl)
    n443 = local read "Stop"() -> (w420:bool)
  }
  n444 = local write "Progress"(u8 0 ("Progress")) -> ()
  n445 = local write "Calibrating"(FALSE ("Calibrating")) -> ()
  n446 = call "InitializeChamberImage.vi"() -> ("error out"=w101:errorcluster, "IMAQ Session Out"=w102:refnum<k11>, "Display Out"=w103:T7, "Acquired Image"=w9:T7)  [unwired: 8 in]
  n447 = node-c288(i64 10 ("Period"), 2 ("Processor")) -> (w15:T12)  [unwired: 2 in]
  n448 = timed-loop {
    tunnel: w103 -> [w772]
    tunnel: w102 -> [w771]
    tunnel: w101 -> [w770]
    tunnel: [w768] -> w100
    tunnel: [w767] -> w99
    timing: w15 -> [_]
    timing-out: [_] -> w14
    i -> [w769]
    stop <- w763 continue-if-true
    n449 = node-c288() -> ()  [unwired: 1 in, 1 out]
    n450 = call <vilib>:"IMAQ Copy Acquired Buffer.vi"("IMAQ Session In"=w771, "Image In"=w772, "Buffer Number"=w769, "error in (no error)"=w770) -> ("IMAQ Session Out"=w768:refnum<k11>, "Image Out"=→"Chamber":T7, "error out"=w767:errorcluster)  [unwired: 7 in, 2 out]
    "Video Error" <- w767
    n451 = local read "Stop"() -> (w765:bool)
    n452 = Unbundle By Name(w767) -> ("status"=w766:bool)
    n453 = Not Or(1:w765, 2:w766) -> (0:w763:bool)
    "Continue to display?" <- w763
    n454 = node-c288() -> ()  [unwired: 1 in, 1 out]
  }
  n455 = node-c288(w14) -> ()  [unwired: 1 out]
  n456 = call <vilib>:"IMAQ Close.vi"("error in (no error)"=w99, "IMAQ Session In"=w100) -> ("error out"=w107:errorcluster)  [unwired: 9 in]
  n457 = call "IMAQ Dispose"("error in (no error)"=w107) -> ("error out"=w106:errorcluster)  [unwired: 5 in]
  n458 = call-poly "VISA Configure Serial Port"("VISA resource name"=refnum<visa-resource-name> "COM3") -> ("VISA resource name out"=w21:refnum<visa-resource-name>, "error out"=w20:errorcluster)  [unwired: 13 in]
  n459 = node-c288(i64 100 ("Period"), 2 ("Processor")) -> (w23:T12)  [unwired: 2 in]
  n460 = call "IMAQ Dispose"("Image"=w9, "error in (no error)"=w106) -> ("error out"=w105:errorcluster)  [unwired: 4 in]
  n461 = timed-loop {
    timing: w23 -> [_]
    timing-out: [_] -> w22
    tunnel: w21 -> [w775]
    tunnel: w20 -> [w777]
    tunnel: [w775] -> w19
    stop <- w776 stop-if-true
    n462 = node-c288() -> ()  [unwired: 1 in, 1 out]
    n463 = event shown="[6] \"Dip\": Value Change" {
      selector: _ -> [_ _ _ _ _ _ _ _ _ _ _]
      dyn-events: _ -> [_ _ _ _ _ _ _ _ _ _ _]
      timeout: _ -> [_ _ _ _ _ _ _ _ _ _ _]
      tunnel: w775 -> [w784 w821 w841 w858 w875 w894 w914 _ _ _ _]
      tunnel: w777 -> [w783 w820 w840 w857 w874 w893 w913 _ _ _ _]
      tunnel: [_ _ _ _ _ _ _ _ _ _ w967] -> w776
      event "Got DNA bead": Value Change {
        n464 = event-data() -> ()  [unwired: 1 in, 5 out]
        n465 = flat-sequence {
          tunnel: w784 -> [w787]
          tunnel: w783 -> [w785]
          tunnel: [w801] -> w782
          tunnel: w782 -> [w804]
          tunnel: [w804] -> w781
          tunnel: w781 -> [w806]
          tunnel: [w806] -> w780
          tunnel: w780 -> [w810]
          tunnel: [w810] -> w779
          tunnel: w779 -> [w812]
          tunnel: [w812] -> w778
          tunnel: w778 -> [w814]
          frame #0 {
            n466 = local read "Saved stage positions"() -> (w788:dbl[][])
            n467 = disable-structure shown="Disabled" {
              frame Disabled {
                n468 = property on="Inject Pump 2" class="Bool (strict)"("Val(Sgnl)"=FALSE ("Inject Pump 2")) -> ()  [unwired: 2 in, 2 out]
              }
              frame Enabled {
              }
            }
            n469 = local write "Stage moving"(TRUE ("Stage moving")) -> ()
            n470 = property on="Trap delta" class="DigNum (strict)"("Val(Sgnl)"="Cal @ Delta (V)") -> ()  [unwired: 2 in, 2 out]
            n471 = call "move to saved stage position.vi"("error in"=w785, "Stage VISA resource name in"=w787, "Position"="Cal stage position", "Saved Stage Positions"=w788) -> ()  [unwired: 2 out]
          }
          frame #1 {
            n472 = local write "Stage moving"(FALSE ("Stage moving")) -> ()
            n473 = property on="Inject Sample" class="Bool (strict)"("Val(Sgnl)"=FALSE ("Value (Signaling)")) -> ()  [unwired: 2 in, 2 out]
            n474 = call <vilib>:"Beep.vi"() -> ()  [unwired: 12 in]
          }
          frame #2 {
            n475 = Wait (ms)(milliseconds to wait=u32 1000) -> ()  [unwired: 1 out]
          }
          frame #3 {
            n476 = property on="Save cal" class="Bool (strict)"("Val(Sgnl)"=TRUE ("Value (Signaling)")) -> ()  [unwired: 2 in, 2 out]
          }
          frame #4 {
            n477 = Wait (ms)(milliseconds to wait=u32 2000) -> ()  [unwired: 1 out]
          }
          frame #5 {
            n478 = while {
              stop <- w798 stop-if-true
              n479 = local read "Saving"() -> (w799:bool)
              n480 = Not(x=w799) -> (.not. x?=w798:bool)
              n481 = Wait (ms)(milliseconds to wait=u32 100) -> ()  [unwired: 1 out]
            }
          }
          frame #6 {
            n482 = Wait (ms)(milliseconds to wait=u32 2000) -> ()  [unwired: 1 out]
          }
          frame #7 {
            # "Only continue if there is no buffer\noverflow error"
            n483 = local read "Buffer Overflow"() -> (w802:bool)
            n484 = Not(x=w802) -> (.not. x?=w801:bool)
            n485 = case shown="True" w801 {
              frame False {
              }
              frame True {
                n486 = property on="Raster scan" class="Bool (strict)"("Val(Sgnl)"=TRUE ("Value (Signaling)")) -> ()  [unwired: 2 in, 2 out]
              }
            }
          }
          frame #8 {
            n487 = case shown="True" w804 {
              frame False {
              }
              frame True {
                n488 = Wait (ms)(milliseconds to wait=u32 2000) -> ()  [unwired: 1 out]
              }
            }
          }
          frame #9 {
            n489 = case shown="True" w806 {
              frame False {
              }
              frame True {
                n490 = while {
                  stop <- w808 stop-if-true
                  n491 = local read "Saving"() -> (w809:bool)
                  n492 = Not(x=w809) -> (.not. x?=w808:bool)
                  n493 = Wait (ms)(milliseconds to wait=u32 100) -> ()  [unwired: 1 out]
                }
              }
            }
          }
          frame #10 {
            n494 = case shown="True" w810 {
              frame False {
              }
              frame True {
                n495 = property on="Read Cal" class="Bool (strict)"("Val(Sgnl)"=TRUE ("Value (Signaling)")) -> ()  [unwired: 2 in, 2 out]
              }
            }
          }
          frame #11 {
            n496 = case shown="True" w812 {
              frame False {
              }
              frame True {
                n497 = Wait (ms)(milliseconds to wait=u32 1000) -> ()  [unwired: 1 out]
              }
            }
          }
          frame #12 {
            n498 = case shown="True" w814 {
              frame False {
              }
              frame True {
                n499 = property on="Fish" class="Bool (strict)"("Val(Sgnl)"=TRUE ("Value (Signaling)")) -> ()  [unwired: 2 in, 2 out]
                n500 = case shown="True" "Flow on\nwhile fish?" {
                  frame False {
                  }
                  frame True {
                    n501 = property on="Inject Sample" class="Bool (strict)"("Val(Sgnl)"=TRUE ("Value (Signaling)")) -> ()  [unwired: 2 in, 2 out]
                  }
                }
              }
            }
          }
        }
      }
      event "Dump beads": Value Change {
        n502 = event-data() -> ()  [unwired: 1 in, 5 out]
        n503 = flat-sequence {
          tunnel: w820 -> [w824]
          tunnel: w821 -> [w825]
          tunnel: [w825] -> w819
          tunnel: [w824] -> w818
          tunnel: w819 -> [w828]
          tunnel: w818 -> [w827]
          frame #0 {
            w822 = FALSE ("Fish")
            n504 = local read "Saving"() -> (w823:bool)
            n505 = local write "Pause dwell"(w822) -> ()
            n506 = local write "Force Feedback"(w822) -> ()
            n507 = local write "Dump beads"(w822) -> ()
            n508 = property on="Stop saving" class="Bool (strict)"("Val(Sgnl)"=w823) -> ()  [unwired: 2 in, 2 out]
            n509 = local write "Fish"(w822) -> ()
          }
          frame #1 {
            n510 = local read "Saved stage positions"() -> (w830:dbl[][])
            n511 = case shown="True" "Flow on\ndump?" {
              frame False {
              }
              frame True {
                n512 = property on="Inject Sample" class="Bool (strict)"("Val(Sgnl)"=TRUE ("Value (Signaling)")) -> ()  [unwired: 2 in, 2 out]
              }
            }
            n513 = local write "Stage moving"(TRUE ("Stage moving")) -> ()
            n514 = call "move to saved stage position.vi"("error in"=w827, "Stage VISA resource name in"=w828, "Position"=5, "Saved Stage Positions"=w830) -> ()  [unwired: 2 out]
          }
          frame #2 {
            n515 = local read "Shutter 1 (B)"() -> (w835:bool)
            n516 = local read "Shutter 2 (A)"() -> (w834:bool)
            n517 = call <vilib>:"Beep.vi"() -> ()  [unwired: 12 in]
            n518 = case shown="True" w835 {
              frame False {
              }
              frame True {
                n519 = property on="Shutter 1 (B)" class="Bool (strict)"("Val(Sgnl)"=FALSE ("Value (Signaling)")) -> ()  [unwired: 2 in, 2 out]
              }
            }
            n520 = case shown="True" w834 {
              frame False {
              }
              frame True {
                n521 = property on="Shutter 2 (A)" class="Bool (strict)"("Val(Sgnl)"=FALSE) -> ()  [unwired: 2 in, 2 out]
              }
            }
            n522 = local write "Stage moving"(FALSE ("Stage moving")) -> ()
            n523 = local write "Tether"(FALSE ("Tether")) -> ()
          }
          frame #3 {
            n524 = property on="Move Cap. 2 (ADig Top)" class="Bool (strict)"("Val(Sgnl)"=TRUE ("Value (Signaling)")) -> ()  [unwired: 2 in, 2 out]
          }
        }
      }
      event "Move Cap. 2 (ADig Top)": Value Change {
        n525 = event-data() -> ()  [unwired: 1 in, 5 out]
        n526 = flat-sequence {
          tunnel: w841 -> [w845]
          tunnel: w840 -> [w844]
          frame #0 {
            n527 = local read "Saved stage positions"() -> (w843:dbl[][])
            n528 = case shown="True" "Flow on\ncap 2?" {
              frame False {
              }
              frame True {
                n529 = property on="Inject Sample" class="Bool (strict)"("Val(Sgnl)"=TRUE ("Value (Signaling)")) -> ()  [unwired: 2 in, 2 out]
              }
            }
            n530 = local write "Move Cap. 2 (ADig Top)"(FALSE ("Move Cap. 2 (ADig Top)")) -> ()
            n531 = local write "Stage moving"(TRUE ("Stage moving")) -> ()
            n532 = call "move to saved stage position.vi"("error in"=w844, "Stage VISA resource name in"=w845, "Position"=2, "Saved Stage Positions"=w843) -> ()  [unwired: 2 out]
          }
          frame #1 {
            # "Make sure you don't reverse\nwhich is ON and OFF"
            n533 = local read "Cal @ Delta (V)"() -> (w852:dbl)
            n534 = local write "Stage moving"(FALSE ("Stage moving")) -> ()
            n535 = call <vilib>:"Beep.vi"() -> ()  [unwired: 12 in]
            n536 = property on="Trap delta" class="DigNum (strict)"("Val(Sgnl)"=w852) -> ()  [unwired: 2 in, 2 out]
            n537 = disable-structure shown="Disabled" {
              frame Disabled {
                n538 = property on="Inject Pump 1" class="Bool (strict)"("Val(Sgnl)"=TRUE ("Inject Pump 2")) -> ()  [unwired: 2 in, 2 out]
              }
              frame Enabled {
              }
            }
            n539 = local read "Shutter 2 (A)"() -> (w851:bool)
            n540 = case shown="False" w851 {
              frame False {
                n541 = property on="Shutter 2 (A)" class="Bool (strict)"("Val(Sgnl)"=TRUE ("Value (Signaling)")) -> ()  [unwired: 2 in, 2 out]
              }
              frame True {
              }
            }
            n542 = property on="Inject Sample" class="Bool (strict)"("Val(Sgnl)"=FALSE ("Value (Signaling)")) -> ()  [unwired: 2 in, 2 out]
          }
        }
      }
      event "Got ADig bead": Value Change {
        n543 = event-data() -> ()  [unwired: 1 in, 5 out]
        n544 = flat-sequence {
          tunnel: w858 -> [w862]
          tunnel: w857 -> [w861]
          frame #0 {
            n545 = local read "Saved stage positions"() -> (w864:dbl[][])
            n546 = property on="Inject Pump 1" class="Bool (strict)"("Val(Sgnl)"=FALSE ("Inject Pump 2")) -> ()  [unwired: 2 in, 2 out]
            n547 = case shown="True" "Flow on\ncap 1?" {
              frame False {
              }
              frame True {
                n548 = property on="Inject Sample" class="Bool (strict)"("Val(Sgnl)"=TRUE ("Value (Signaling)")) -> ()  [unwired: 2 in, 2 out]
              }
            }
            n549 = local write "Stage moving"(TRUE ("Stage moving")) -> ()
            n550 = call "move to saved stage position.vi"("error in"=w861, "Stage VISA resource name in"=w862, "Position"=1, "Saved Stage Positions"=w864) -> ()  [unwired: 2 out]
          }
          frame #1 {
            n551 = local read "Shutter 1 (B)"() -> (w868:bool)
            n552 = disable-structure shown="Disabled" {
              frame Disabled {
                n553 = property on="Inject Pump 2" class="Bool (strict)"("Val(Sgnl)"=TRUE ("Inject Pump 2")) -> ()  [unwired: 2 in, 2 out]
              }
              frame Enabled {
              }
            }
            n554 = local write "Stage moving"(FALSE ("Stage moving")) -> ()
            n555 = case shown="False" w868 {
              frame False {
                n556 = property on="Shutter 1 (B)" class="Bool (strict)"("Val(Sgnl)"=TRUE ("Value (Signaling)")) -> ()  [unwired: 2 in, 2 out]
              }
              frame True {
              }
            }
            n557 = property on="Inject Sample" class="Bool (strict)"("Val(Sgnl)"=FALSE ("Value (Signaling)")) -> ()  [unwired: 2 in, 2 out]
            n558 = call <vilib>:"Beep.vi"() -> ()  [unwired: 12 in]
          }
        }
        n559 = local write "Got ADig bead"(FALSE ("Got ADig bead")) -> ()
      }
      event "Set Position 1", "Set Position 2", "Set Position 3", "Set Position 4", "Set Position 5": Value Change {
        n560 = event-data() -> ()  [unwired: 1 in, 5 out]
        n561 = Build Array("Set Position 1", "Set Position 2", "Set Position 3", "Set Position 4", "Set Position 5") -> (w887:bool[])
        n562 = Boolean Array To Number(Boolean array=w887) -> (number=w886:u32)
        n563 = call "Read Stage Position.vi"("error in"=w874, "VISA resource name in"=w875) -> ("Current Position"=w872:cluster{dbl, dbl, dbl}, "error out"=→"Stage error":errorcluster)  [unwired: 1 in, 1 out]
        n564 = Logarithm Base 2(1:w886) -> (0:w880:dbl)
        n565 = Cluster To Array(cluster=w872) -> (array=w882:dbl[])
        n566 = Increment(x=w880) -> (x+1=w883:dbl)
        n567 = Build Array (concatenate)(w883, w882) -> (w881:dbl[])
        n568 = Replace Array Subset(array="Saved stage positions", new element=w881, index (row)=w880) -> (w884:dbl[][])  [unwired: 1 in]
        n569 = local write "Saved stage positions"(w884) -> ()
      }
      event "Move to Position 2", "Move to Position 4", "Move to Position 3", "Move to Position 5", "Move to Position 1": Value Change {
        n570 = event-data() -> ()  [unwired: 1 in, 5 out]
        n571 = Build Array("Move to Position 1", "Move to Position 2", "Move to Position 3", "Move to Position 4", "Move to Position 5") -> (w897:bool[])
        n572 = Boolean Array To Number(Boolean array=w897) -> (number=w896:u32)
        n573 = Logarithm Base 2(1:w896) -> (0:w895:dbl)
        n574 = flat-sequence {
          tunnel: w895 -> [w902]
          tunnel: w894 -> [w901]
          tunnel: w893 -> [w900]
          frame #0 {
            n575 = local read "Saved stage positions"() -> (w903:dbl[][])
            n576 = Increment(x=w902) -> (x+1=w899:dbl)
            n577 = call "move to saved stage position.vi"("error in"=w900, "Stage VISA resource name in"=w901, "Position"=w899, "Saved Stage Positions"=w903) -> ()  [unwired: 2 out]
            "Stage moving" <- TRUE ("Stage moving")
          }
          frame #1 {
            n578 = call <vilib>:"Beep.vi"() -> ()  [unwired: 12 in]
            n579 = local write "Stage moving"(FALSE ("Stage moving")) -> ()
          }
        }
      }
      event "Dip": Value Change {
        n580 = event-data() -> ()  [unwired: 1 in, 5 out]
        n581 = local write "Dip"(FALSE ("Dip")) -> ()
        n582 = flat-sequence {
          tunnel: w914 -> [w916]
          tunnel: w913 -> [w915]
          tunnel: [w917] -> w911
          tunnel: [w916] -> w909
          tunnel: [w915] -> w907
          tunnel: [w925] -> w912
          tunnel: w911 -> [w925]
          tunnel: [w924] -> w910
          tunnel: w909 -> [w924]
          tunnel: [w923] -> w908
          tunnel: w907 -> [w923]
          tunnel: w912 -> [w944]
          tunnel: w910 -> [w943]
          tunnel: w908 -> [w942]
          frame #0 {
            n583 = local read "Saved stage positions"() -> (w917:dbl[][])
            n584 = local write "Stage moving"(TRUE) -> ()
            n585 = call "move to saved stage position.vi"("error in"=w915, "Stage VISA resource name in"=w916, "Position"="Dip position", "Saved Stage Positions"=w917) -> ()  [unwired: 2 out]
          }
          frame #1 {
            n586 = node-c288() -> (w922:T12)  [unwired: 4 in]
            n587 = timed-loop {
              timing: w922 -> [_]
              timing-out: [_] -> w921
              i -> [w935]
              stop <- w926 stop-if-true
              n588 = node-c288() -> ()  [unwired: 1 in, 1 out]
              n589 = Greater Or Equal?(x=w935, y="Dip duration") -> (x >= y?=w931:bool)
              n590 = local read "Dump beads"() -> (w928:bool)
              n591 = Or(x=w931, y="Cancel dwell") -> (x .or. y?=w929:bool)
              n592 = Not(x="Pause dwell") -> (.not. x?=w932:bool)
              n593 = node-c288() -> ()  [unwired: 1 in, 1 out]
              n594 = And(x=w932, y=w929) -> (x .and. y?=w927:bool)
              n595 = Or(x=w927, y=w928) -> (x .or. y?=w926:bool)
              "Dip time" <- w935
            }
            n596 = local write "Stage moving"(FALSE ("Stage moving")) -> ()
            n597 = node-c288(w921) -> ()  [unwired: 1 out]
          }
          frame #2 {
            n598 = local write "Cancel dwell"(FALSE ("Cancel dwell")) -> ()
            n599 = call "move to saved stage position.vi"("error in"=w942, "Stage VISA resource name in"=w943, "Position"="Return position", "Saved Stage Positions"=w944) -> ()  [unwired: 2 out]
          }
          frame #3 {
            n600 = local write "Stage moving"(FALSE ("Stage moving")) -> ()
          }
        }
      }
      event "Force FB script": Value Change {
        n601 = event-data() -> ()  [unwired: 1 in, 5 out]
        n602 = flat-sequence {
          frame #0 {
            n603 = disable-structure shown="Disabled" {
              frame Disabled {
                n604 = local read "# Samples/channel"() -> (w948:i32)
                n605 = local write "# Samples/channel (in)"(w948) -> ()
              }
              frame Enabled {
              }
            }
            n606 = local write "Force FB script"(FALSE ("Force FB script")) -> ()
            n607 = property on="Trap delta" class="DigNum (strict)"("Val(Sgnl)"="Start trap delta (V)") -> ()  [unwired: 2 in, 2 out]
          }
          frame #1 {
            n608 = Wait (ms)(milliseconds to wait=u32 500) -> ()  [unwired: 1 out]
          }
          frame #2 {
            n609 = property on="Set reading to\nsetpoint" class="Bool (strict)"("Val(Sgnl)"=TRUE ("Value (Signaling)")) -> ()  [unwired: 2 in, 2 out]
          }
          frame #3 {
            n610 = Wait (ms)(milliseconds to wait=u32 300) -> ()  [unwired: 1 out]
          }
          frame #4 {
            n611 = local write "Force Feedback"(TRUE ("Force Feedback")) -> ()
            n612 = property on="Tabs" class="TabCtl (strict)"("Val(Sgnl)"=T3."Force Feedback" ("Value (Signaling)")) -> ()  [unwired: 2 in, 2 out]
          }
          frame #5 {
            n613 = property on="Save Data" class="Bool (strict)"("Val(Sgnl)"=TRUE ("Value (Signaling)")) -> ()  [unwired: 2 in, 2 out]
          }
          frame #6 {
            n614 = Multiply(x="Wait before dip (s)", y=1000) -> (x*y=w955:dbl)
            n615 = Wait (ms)(milliseconds to wait=w955) -> ()  [unwired: 1 out]
          }
          frame #7 {
            n616 = case shown="True" "Start dipping after?" {
              selector: "Start dipping after?" -> [_ w960]
              frame False {
              }
              frame True {
                n617 = property on="Dip" class="Bool (strict)"("Val(Sgnl)"=w960) -> ()  [unwired: 2 in, 2 out]
              }
            }
            n618 = property on="Remove offsets" class="Bool (strict)"("Val(Sgnl)"=TRUE ("Value (Signaling)")) -> ()  [unwired: 2 in, 2 out]
          }
        }
      }
      event "Move 0": Value Change {
        n619 = event-data() -> ()  [unwired: 1 in, 5 out]
        n620 = local write "Move 0"(FALSE) -> ()
        n621 = call "HalfWavePlate.vi"("Degrees"="\"Degrees\" 0", "Motor"=0) -> ()  [unwired: 1 in]
      }
      event "Move 1": Value Change {
        n622 = event-data() -> ()  [unwired: 1 in, 5 out]
        n623 = local write "Move 1"(FALSE) -> ()
        n624 = call "HalfWavePlate.vi"("Degrees"="\"Degrees\" 1", "Motor"=1) -> ()  [unwired: 1 in]
      }
      event "Stop": Value Change {
        n625 = event-data() -> ()  [unwired: 1 in, 5 out]
        n626 = local read "Stop"() -> (w967:bool)
      }
    }
    n627 = node-c288() -> ()  [unwired: 1 in, 1 out]
  }
  n628 = call <vilib>:"Simple Error Handler.vi"("error in (no error)"=w105) -> ()  [unwired: 4 in, 5 out]
  n629 = node-c288(2 ("Processor")) -> (w75:T12)  [unwired: 3 in]
  n630 = node-c288(2 ("Processor")) -> (w27:T12)  [unwired: 3 in]
  n631 = timed-loop {
    timing: w75 -> [_]
    timing-out: [_] -> w74
    stop <- w970 stop-if-true
    n632 = node-c288() -> ()  [unwired: 1 in, 1 out]
    n633 = case shown="\"Current Saved Data\"" "Tab Control" {
      frame "Control" {
        n634 = case shown="True" "Start" {
          frame False {
          }
          frame True {
            w983 = T15 3 items=["no dialog", "OK message", "continue or stop message", "OK message + warnings", "continue/stop + warnings"] ("type of dialog (OK msg:1)")
            n635 = call "InitializeAcquireFF.vi"("DAQ Rate"="DAQ Rate", "Averaging Number"="Averaging Number", "Sampling Rate"="Sampling Rate") -> ("error out"=w977:errorcluster, "task out"=w976:refnum<k21>, "Final Sampling Rate"=→"Final Sampling Rate":dbl)  [unwired: 4 in, 2 out]
            n636 = while {
              tunnel: [w995] -> w982
              tunnel: [w994] -> w975
              tunnel: "Averaging Number" -> [w993]
              tunnel: w977 -> [w992]
              tunnel: w976 -> [w990]
              stop <- w991 continue-if-true
              n637 = call "Acquire2_QPD.vi"("task/channels in"=w990, "Save Data?"=FALSE ("Take Data?"), "Averaging Number"=w993, "error in"=w992) -> ("PSD 1"=→"PSD 1":cluster{dbl[], dbl[]}, "PSD 1 Sum"=→"PSD 1 Sum":dbl, "PSD 2"=→"PSD 2":cluster{dbl[], dbl[]}, "PSD 2 Sum"=→"PSD 2 Sum":dbl, "task out"=w995:refnum<k21>, "error out"=w994:errorcluster)  [unwired: 14 in, 4 out]
              n638 = local read "Start"() -> (w991:bool)
            }
            n639 = call <vilib>:"DAQmx Clear Task.vi"("task in"=w982, "error in"=w975) -> ("error out"=w984:errorcluster)  [unwired: 13 in]
            n640 = call <vilib>:"Simple Error Handler.vi"("type of dialog (OK msg:1)"=w983, "error in (no error)"=w984) -> ()  [unwired: 3 in, 5 out]
          }
        }
      }
      frame "Current Saved Data" {
      }
      frame "Data Acquisition" {
      }
      frame "Raw QPD Data" {
      }
    }
    n641 = local read "Stop"() -> (w970:bool)
    n642 = node-c288() -> ()  [unwired: 1 in, 1 out]
  }
  n643 = call-poly <vilib>:"DAQmx Create Virtual Channel.vi"("lines"=w92) -> ("task out"=w91:refnum<k21>)  [unwired: 13 in, 1 out]
  n644 = call-poly <vilib>:"DAQmx Create Virtual Channel.vi"("lines"=w95) -> ("task out"=w94:refnum<k21>)  [unwired: 13 in, 1 out]
  n645 = timed-loop {
    timing: w27 -> [_]
    timing-out: [_] -> w26
    stop <- w996 stop-if-true
    n646 = node-c288() -> ()  [unwired: 1 in, 1 out]
    n647 = event shown="[0] \"Pause Mouse/Mirror Connection\": Value Change" {
      selector: _ -> [_ _]
      dyn-events: _ -> [_ _]
      timeout: _ -> [_ _]
      tunnel: [w1089 _] -> w997
      tunnel: [_ w1090] -> w996
      event "Pause Mouse/Mirror Connection": Value Change {
        n648 = event-data() -> ("NewVal"=w1089:bool)  [unwired: 1 in]
      }
      event "Stop": Value Change {
        n649 = event-data() -> ("NewVal"=w1090:bool)  [unwired: 1 in]
      }
    }
    n650 = case shown="True" w997 {
      frame False {
      }
      frame True {
        n651 = call "InitializeMouseControl.vi"() -> ("error out 2"=w1006:errorcluster, "task out"=w1007:refnum<k21>, "error out"=w1009:errorcluster, "device ID"=w1008:refnum<k1>)  [unwired: 8 in]
        n652 = while {
          tunnel: w1009 -> [w1021]
          tunnel: w1008 -> [w1020]
          tunnel: w1007 -> [w1019]
          tunnel: w1006 -> [w1018]
          tunnel: [w1017] -> w1004
          tunnel: [w1016] -> w1003
          tunnel: [w1015] -> w1000
          tunnel: [w1014] -> w1001
          stop <- w1013 stop-if-true
          n653 = case shown="True" "Use Mouse to Move Trap?" {
            tunnel: w1020 -> [w1028 w1051]
            tunnel: w1021 -> [w1027 w1050]
            tunnel: w1019 -> [w1026 w1049]
            tunnel: w1018 -> [w1025 w1048]
            tunnel: [w1028 w1047] -> w1015
            tunnel: [w1027 w1046] -> w1014
            tunnel: [w1026 w1045] -> w1017
            tunnel: [w1025 w1044] -> w1016
            frame False {
              (unwired) FALSE ("button 1")
            }
            frame True {
              w1039 = 0.0 ("y")
              w1041 = 10
              n654 = local read "Deflection"() -> (w1052:T4)
              n655 = call-poly <vilib>:"Acquire Input Data.vi"("device ID"=w1051, "error in (no error)"=w1050) -> ("device ID"=w1047:refnum<k1>, "button info"=w1065:T16, "error out"=w1046:errorcluster)  [unwired: 14 in, 1 out]
              n656 = Unbundle By Name(w1052) -> ("Horizontal"=w1054:i32, "Vertical"=w1053:i32)
              n657 = local read "Saved voltage"() -> (w1030:cluster{dbl, dbl})
              n658 = Divide(x=w1054, y=30) -> (x/y=w1057:dbl)
              n659 = Divide(x=w1053, y=-20) -> (x/y=w1058:dbl)
              n660 = Unbundle By Name(w1065) -> ("button 1"=w1043:bool, "button 2"=w1059:bool)
              n661 = Bundle(w1057, w1058) -> (w1035:cluster{dbl, dbl})  [unwired: 1 in]
              n662 = local write "Reference Voltage"(w1035) -> ()
              n663 = Add(x=w1035, y=w1030) -> (x+y=w1063:cluster{dbl, dbl})
              n664 = case shown="True" w1043 {
                frame False {
                  n665 = stacked-sequence {
                    frame #0 {
                      n666 = local write "CoordinatesMousePressed"(T4 {"Horizontal"=0, "Vertical"=0} ("Coords when pressed")) -> ()
                      n667 = local write "Deflection"(T4 {"Horizontal"=0, "Vertical"=0} ("deflaction")) -> ()
                    }
                  }
                }
                frame True {
                  n668 = local read "CoordinatesMousePressed"() -> (w1088:T4)
                  n669 = local read "Real Coordinates"() -> (w1087:cluster{"Horizontal":i32, "Vertical":i32})
                  n670 = Subtract(x=w1087, y=w1088) -> (x-y=w1086:T4)
                  n671 = local write "Deflection"(w1086) -> ()
                }
              }
              n672 = Unbundle(w1063) -> (w1040:dbl, w1031:dbl)
              n673 = case shown="True" w1059 {
                frame False {
                }
                frame True {
                  n674 = local read "Reference Voltage"() -> (w1069:cluster{dbl, dbl})
                  n675 = local read "Saved voltage"() -> (w1067:cluster{dbl, dbl})
                  n676 = Add(x=w1069, y=w1067) -> (x+y=→"Saved voltage":cluster{dbl, dbl})
                  n677 = local read "Real Coordinates"() -> (w1068:cluster{"Horizontal":i32, "Vertical":i32})
                  n678 = local write "CoordinatesMousePressed"(w1068) -> ()
                }
              }
              n679 = Less?(x=w1040, y=w1041) -> (x < y?=w1038:bool)
              n680 = Greater?(x=w1040, y=w1039) -> (0:w1037:bool)
              n681 = Greater?(x=w1031, y=w1039) -> (0:w1033:bool)
              n682 = Less?(x=w1031, y=w1041) -> (x < y?=w1034:bool)
              n683 = And(x=w1033, y=w1034) -> (x .and. y?=w1032:bool)
              n684 = And(x=w1038, y=w1037) -> (x .and. y?=w1036:bool)
              n685 = case shown="False" w1032 {
                tunnel: [w1079 w1083] -> w1042
                tunnel: w1031 -> [w1077 w1083]
                frame False {
                  n686 = Greater?(x=w1077, y=10.0) -> (0:w1080:bool)
                  n687 = case shown="True" w1080 {
                    tunnel: [0.0 10.0] -> w1079
                    frame False {
                    }
                    frame True {
                    }
                  }
                }
                frame True {
                }
              }
              n688 = case shown="False" w1036 {
                tunnel: w1040 -> [w1071 w1076]
                tunnel: [w1072 w1076] -> w1064
                frame False {
                  n689 = Greater?(x=w1071, y=10.0) -> (0:w1073:bool)
                  n690 = case shown="True" w1073 {
                    tunnel: [0.0 10.0] -> w1072
                    frame False {
                    }
                    frame True {
                    }
                  }
                }
                frame True {
                }
              }
              n691 = Bundle(w1064, w1042) -> (w1029:cluster{dbl, dbl})  [unwired: 1 in]
              n692 = Cluster To Array(cluster=w1029) -> (array=w1060:dbl[])
              n693 = call-poly <vilib>:"DAQmx Write.vi"("task/channels in"=w1049, "data"=w1060, "error in"=w1048) -> ("task out"=w1062:refnum<k21>, "error out"=w1061:errorcluster)  [unwired: 10 in, 1 out]
              n694 = call <vilib>:"DAQmx Is Task Done.vi"("task/channels in"=w1062, "error in"=w1061) -> ("task out"=w1045:refnum<k21>, "error out"=w1044:errorcluster)  [unwired: 11 in, 1 out]
            }
          }
          n695 = event shown="[0] \"Pane\": Mouse Move" {
            selector: _ -> [_ _ _]
            dyn-events: _ -> [_ _ _]
            timeout: _ -> [_ _ _]
            event Mouse Move {
              n696 = event-data() -> ("Coords"=w1023:T4)  [unwired: 1 in]
              n697 = local write "Real Coordinates"(w1023) -> ()
            }
            event Mouse Down {
              n698 = event-data() -> ("Coords"=w1024:T4)  [unwired: 1 in]
              n699 = local write "CoordinatesMousePressed"(w1024) -> ()
            }
            event "Pause Mouse/Mirror Connection": Value Change {
              n700 = event-data() -> ()  [unwired: 1 in, 3 out]
            }
          }
          n701 = local read "Stop"() -> (w1010:bool)
          n702 = Not(x="Pause Mouse/Mirror Connection") -> (.not. x?=w1011:bool)
          n703 = Or(x=w1011, y=w1010) -> (x .or. y?=w1013:bool)
        }
        n704 = call <vilib>:"DAQmx Clear Task.vi"("task in"=w1004, "error in"=w1003) -> ("error out"=w1005:errorcluster)  [unwired: 13 in]
        n705 = call <vilib>:"Simple Error Handler.vi"("error in (no error)"=w1005) -> ()  [unwired: 4 in, 5 out]
        n706 = call-poly <vilib>:"Close Input Device.vi"("error in (no error)"=w1001, "device ID"=w1000) -> ("error out"=w1002:errorcluster)  [unwired: 8 in]
        n707 = call <vilib>:"Simple Error Handler.vi"("error in (no error)"=w1002) -> ()  [unwired: 4 in, 5 out]
      }
    }
    n708 = node-c288() -> ()  [unwired: 1 in, 1 out]
  }
  n709 = node-c288(i64 100 ("Period")) -> (w89:T12)  [unwired: 3 in]
  n710 = timed-loop {
    tunnel: w91 -> [w1093]
    tunnel: [w1092] -> w90
    tunnel: w94 -> [w1095]
    tunnel: [w1094] -> w93
    timing: w89 -> [_]
    timing-out: [_] -> w88
    stop <- w1091 stop-if-true
    n711 = node-c288() -> ()  [unwired: 1 in, 1 out]
    n712 = event shown="[1] \"Shutter 2 (A)\": Value Change" {
      selector: _ -> [_ _ _]
      dyn-events: _ -> [_ _ _]
      timeout: _ -> [_ _ _]
      tunnel: w1095 -> [w1099 _ _]
      tunnel: [w1098 _ _] -> w1094
      tunnel: w1093 -> [_ w1119 _]
      tunnel: [_ w1117 _] -> w1092
      tunnel: [_ _ w1136] -> w1091
      event "Shutter 1 (B)": Value Change {
        n713 = event-data() -> ()  [unwired: 1 in, 1 out]
        n714 = flat-sequence {
          tunnel: [w1105] -> w1102
          tunnel: w1099 -> [w1104]
          tunnel: [w1109] -> w1101
          tunnel: [w1112] -> w1100
          tunnel: w1102 -> [w1107]
          tunnel: w1101 -> [w1116]
          tunnel: w1100 -> [w1114]
          tunnel: [w1113] -> w1098
          frame #0 {
            n715 = call-poly <vilib>:"DAQmx Write.vi"("task/channels in"=w1104, "data"=FALSE) -> ("task out"=w1105:refnum<k21>)  [unwired: 11 in, 2 out]
            n716 = Wait (ms)(milliseconds to wait=100) -> ()  [unwired: 1 out]
          }
          frame #1 {
            n717 = Or(x="Shutter 1 (B)", y=TRUE) -> (x .or. y?=w1109:bool)
            n718 = call-poly <vilib>:"DAQmx Write.vi"("task/channels in"=w1107, "data"=w1109) -> ("task out"=w1112:refnum<k21>)  [unwired: 11 in, 2 out]
            n719 = Wait (ms)(milliseconds to wait=100) -> ()  [unwired: 1 out]
          }
          frame #2 {
            n720 = Not(x=w1116) -> (.not. x?=w1115:bool)
            n721 = call-poly <vilib>:"DAQmx Write.vi"("task/channels in"=w1114, "data"=w1115) -> ("task out"=w1113:refnum<k21>)  [unwired: 11 in, 2 out]
          }
        }
      }
      event "Shutter 2 (A)": Value Change {
        n722 = event-data() -> ()  [unwired: 1 in, 1 out]
        n723 = flat-sequence {
          tunnel: w1119 -> [w1124]
          tunnel: [w1123] -> w1118
          tunnel: [w1128] -> w1121
          tunnel: [w1131] -> w1120
          tunnel: w1118 -> [w1126]
          tunnel: w1121 -> [w1135]
          tunnel: w1120 -> [w1133]
          tunnel: [w1132] -> w1117
          frame #0 {
            n724 = call-poly <vilib>:"DAQmx Write.vi"("task/channels in"=w1124, "data"=FALSE) -> ("task out"=w1123:refnum<k21>)  [unwired: 11 in, 2 out]
            n725 = Wait (ms)(milliseconds to wait=100) -> ()  [unwired: 1 out]
          }
          frame #1 {
            n726 = Or(x="Shutter 2 (A)", y=TRUE) -> (x .or. y?=w1128:bool)
            n727 = call-poly <vilib>:"DAQmx Write.vi"("task/channels in"=w1126, "data"=w1128) -> ("task out"=w1131:refnum<k21>)  [unwired: 11 in, 2 out]
            n728 = Wait (ms)(milliseconds to wait=100) -> ()  [unwired: 1 out]
          }
          frame #2 {
            n729 = Not(x=w1135) -> (.not. x?=w1134:bool)
            n730 = call-poly <vilib>:"DAQmx Write.vi"("task/channels in"=w1133, "data"=w1134) -> ("task out"=w1132:refnum<k21>)  [unwired: 11 in, 2 out]
          }
        }
      }
      event "Stop": Value Change {
        n731 = event-data() -> ("NewVal"=w1136:bool)  [unwired: 1 in, 5 out]
      }
    }
    n732 = node-c288() -> ()  [unwired: 1 in, 1 out]
  }
  n733 = node-c288(w88) -> ()  [unwired: 1 out]
  n734 = node-c288(w74) -> ()  [unwired: 1 out]
  n735 = call <vilib>:"DAQmx Clear Task.vi"("task in"=w90) -> ()  [unwired: 14 in, 1 out]
  n736 = call <vilib>:"DAQmx Clear Task.vi"("task in"=w93) -> ()  [unwired: 14 in, 1 out]
  n737 = node-c288(w26) -> ()  [unwired: 1 out]
  n738 = node-c288(w22) -> ()  [unwired: 1 out]
  n739 = disable-structure shown="Enabled" {
    frame Disabled {
      n740 = node-c288(2 ("Processor")) -> (w1140:T12)  [unwired: 3 in]
      n741 = timed-loop "Pump Control" {
        timing: w1140 -> [_]
        timing-out: [_] -> w1139
        tunnel: refnum<visa-resource-name> "COM6" ("VISA resource name") -> [w1142]
        stop <- w1141 stop-if-true
        n742 = node-c288() -> ()  [unwired: 1 in, 1 out]
        n743 = event shown="[4] \"Inject Pump 1\": Value Change" {
          selector: _ -> [_ _ _ _ _ _ _ _ _]
          dyn-events: _ -> [_ _ _ _ _ _ _ _ _]
          timeout: _ -> [_ _ _ _ _ _ _ _ _]
          tunnel: w1142 -> [w1150 w1246 _ w1322 w1450 w1593 w1638 w1696 w1755]
          tunnel: [_ _ w1321 _ _ _ _ _ _] -> w1141
          event "Flush Pump 1": Value Change {
            w1151 = "\r"
            n744 = event-data() -> ()  [unwired: 1 in, 5 out]
            n745 = call-poly "VISA Configure Serial Port"("VISA resource name"=w1150) -> ("VISA resource name out"=w1164:refnum<visa-resource-name>, "error out"=w1165:errorcluster)  [unwired: 13 in]
            n746 = local read "Write Wait"() -> (w1143:i32)
            n747 = Concatenate Strings("enter pump1", w1151) -> (w1152:string)
            n748 = flat-sequence {
              tunnel: w1165 -> [w1184]
              tunnel: w1164 -> [w1186]
              tunnel: [w1185] -> w1181
              tunnel: [w1183] -> w1180
              tunnel: w1152 -> [w1182]
              tunnel: w1181 -> [w1189]
              tunnel: [w1189] -> w1179
              tunnel: w1180 -> [w1188]
              tunnel: [w1188] -> w1178
              tunnel: w1143 -> [w1187]
              tunnel: [w1194] -> w1177
              tunnel: w1157 -> [w1193]
              tunnel: [w1190] -> w1176
              tunnel: w1179 -> [w1192]
              tunnel: w1178 -> [w1191]
              tunnel: w1177 -> [w1197]
              tunnel: [w1197] -> w1175
              tunnel: [w1196] -> w1174
              tunnel: w1176 -> [w1196]
              tunnel: w1143 -> [w1195]
              tunnel: w1175 -> [w1202]
              tunnel: [w1201] -> w1173
              tunnel: w1160 -> [w1200]
              tunnel: w1174 -> [w1199]
              tunnel: [w1198] -> w1172
              tunnel: w1173 -> [w1205]
              tunnel: [w1205] -> w1171
              tunnel: [w1204] -> w1170
              tunnel: w1172 -> [w1204]
              tunnel: w1143 -> [w1203]
              tunnel: w1171 -> [w1210]
              tunnel: [w1209] -> w1169
              tunnel: w1163 -> [w1208]
              tunnel: w1170 -> [w1207]
              tunnel: [w1206] -> w1168
              tunnel: [w1213] -> w1167
              tunnel: w1169 -> [w1213]
              tunnel: [w1212] -> w1166
              tunnel: w1168 -> [w1212]
              tunnel: w1143 -> [w1211]
              tunnel: w1167 -> [w1218]
              tunnel: w1166 -> [w1215]
              tunnel: [w1217] -> w1146
              tunnel: [w1216] -> w1144
              tunnel: [w1223] -> w1147
              tunnel: w1146 -> [w1223]
              tunnel: [w1222] -> w1145
              tunnel: w1144 -> [w1222]
              tunnel: w1143 -> [w1221]
              tunnel: w1147 -> [w1225]
              tunnel: w1145 -> [w1224]
              frame #0 {
                n749 = VISA Write(VISA resource name=w1186, write buffer=w1182, error in (no error)=w1184) -> (VISA resource name out=w1185:refnum<visa-resource-name>, error out=w1183:errorcluster)  [unwired: 1 out]
              }
              frame #1 {
                n750 = Wait (ms)(milliseconds to wait=w1187) -> ()  [unwired: 1 out]
              }
              frame #2 {
                n751 = VISA Write(VISA resource name=w1192, write buffer=w1193, error in (no error)=w1191) -> (VISA resource name out=w1194:refnum<visa-resource-name>, error out=w1190:errorcluster)  [unwired: 1 out]
              }
              frame #3 {
                n752 = Wait (ms)(milliseconds to wait=w1195) -> ()  [unwired: 1 out]
              }
              frame #4 {
                n753 = VISA Write(VISA resource name=w1202, write buffer=w1200, error in (no error)=w1199) -> (VISA resource name out=w1201:refnum<visa-resource-name>, error out=w1198:errorcluster)  [unwired: 1 out]
              }
              frame #5 {
                n754 = Wait (ms)(milliseconds to wait=w1203) -> ()  [unwired: 1 out]
              }
              frame #6 {
                n755 = VISA Write(VISA resource name=w1210, write buffer=w1208, error in (no error)=w1207) -> (VISA resource name out=w1209:refnum<visa-resource-name>, error out=w1206:errorcluster)  [unwired: 1 out]
              }
              frame #7 {
                n756 = Wait (ms)(milliseconds to wait=w1211) -> ()  [unwired: 1 out]
              }
              frame #8 {
                n757 = Concatenate Strings("start ", "\r") -> (w1214:string)
                n758 = VISA Write(VISA resource name=w1218, write buffer=w1214, error in (no error)=w1215) -> (VISA resource name out=w1217:refnum<visa-resource-name>, error out=w1216:errorcluster)  [unwired: 1 out]
              }
              frame #9 {
                n759 = Wait (ms)(milliseconds to wait=w1221) -> ()  [unwired: 1 out]
              }
              frame #10 {
                n760 = local write "Flush Pump 1"(FALSE ("Flush Pump 1")) -> ()
                n761 = Concatenate Strings("enter main ", "\r") -> (w1229:string)
                n762 = VISA Write(VISA resource name=w1225, write buffer=w1229, error in (no error)=w1224) -> (VISA resource name out=w1228:refnum<visa-resource-name>, error out=w1227:errorcluster)  [unwired: 1 out]
                n763 = VISA Close(VISA resource name=w1228, error in (no error)=w1227) -> ()  [unwired: 1 out]
              }
            }
            n764 = Concatenate Strings("set units 4 ", w1151) -> (w1157:string)
            n765 = Multiply(x="Flush\nRate (ul/min)", y=60) -> (x*y=w1155:dbl)
            n766 = Number To Decimal String(number=w1155) -> (decimal integer string=w1158:string)  [unwired: 1 in]
            n767 = Concatenate Strings("set rate ", w1158, w1151) -> (w1160:string)
            n768 = Number To Decimal String(number="Flush\nVolume (ul)") -> (decimal integer string=w1162:string)  [unwired: 1 in]
            n769 = Concatenate Strings("set volume ", w1162, w1151) -> (w1163:string)
          }
          event "Flush Pump 2": Value Change {
            w1237 = "\r"
            n770 = event-data() -> ()  [unwired: 1 in, 5 out]
            n771 = call-poly "VISA Configure Serial Port"("VISA resource name"=w1246) -> ("VISA resource name out"=w1257:refnum<visa-resource-name>, "error out"=w1258:errorcluster)  [unwired: 13 in]
            n772 = local read "Write Wait"() -> (w1232:i32)
            n773 = Concatenate Strings("enter pump2", w1237) -> (w1238:string)
            n774 = flat-sequence {
              tunnel: w1258 -> [w1273]
              tunnel: w1257 -> [w1275]
              tunnel: [w1274] -> w1243
              tunnel: [w1272] -> w1241
              tunnel: w1238 -> [w1271]
              tunnel: w1243 -> [w1278]
              tunnel: [w1278] -> w1242
              tunnel: w1241 -> [w1277]
              tunnel: [w1277] -> w1240
              tunnel: w1232 -> [w1276]
              tunnel: [w1283] -> w1270
              tunnel: w1250 -> [w1282]
              tunnel: [w1279] -> w1269
              tunnel: w1242 -> [w1281]
              tunnel: w1240 -> [w1280]
              tunnel: w1270 -> [w1286]
              tunnel: [w1286] -> w1268
              tunnel: [w1285] -> w1267
              tunnel: w1269 -> [w1285]
              tunnel: w1232 -> [w1284]
              tunnel: w1268 -> [w1291]
              tunnel: [w1290] -> w1266
              tunnel: w1253 -> [w1289]
              tunnel: w1267 -> [w1288]
              tunnel: [w1287] -> w1265
              tunnel: w1266 -> [w1294]
              tunnel: [w1294] -> w1264
              tunnel: [w1293] -> w1263
              tunnel: w1265 -> [w1293]
              tunnel: w1232 -> [w1292]
              tunnel: w1264 -> [w1299]
              tunnel: [w1298] -> w1262
              tunnel: w1256 -> [w1297]
              tunnel: w1263 -> [w1296]
              tunnel: [w1295] -> w1261
              tunnel: [w1302] -> w1260
              tunnel: w1262 -> [w1302]
              tunnel: [w1301] -> w1259
              tunnel: w1261 -> [w1301]
              tunnel: w1232 -> [w1300]
              tunnel: w1260 -> [w1309]
              tunnel: w1259 -> [w1308]
              tunnel: [w1304] -> w1236
              tunnel: [w1303] -> w1234
              tunnel: w1236 -> [w1312]
              tunnel: [w1312] -> w1235
              tunnel: w1234 -> [w1311]
              tunnel: [w1311] -> w1233
              tunnel: w1232 -> [w1310]
              tunnel: w1235 -> [w1316]
              tunnel: w1233 -> [w1315]
              frame #0 {
                n775 = VISA Write(VISA resource name=w1275, write buffer=w1271, error in (no error)=w1273) -> (VISA resource name out=w1274:refnum<visa-resource-name>, error out=w1272:errorcluster)  [unwired: 1 out]
              }
              frame #1 {
                n776 = Wait (ms)(milliseconds to wait=w1276) -> ()  [unwired: 1 out]
              }
              frame #2 {
                n777 = VISA Write(VISA resource name=w1281, write buffer=w1282, error in (no error)=w1280) -> (VISA resource name out=w1283:refnum<visa-resource-name>, error out=w1279:errorcluster)  [unwired: 1 out]
              }
              frame #3 {
                n778 = Wait (ms)(milliseconds to wait=w1284) -> ()  [unwired: 1 out]
              }
              frame #4 {
                n779 = VISA Write(VISA resource name=w1291, write buffer=w1289, error in (no error)=w1288) -> (VISA resource name out=w1290:refnum<visa-resource-name>, error out=w1287:errorcluster)  [unwired: 1 out]
              }
              frame #5 {
                n780 = Wait (ms)(milliseconds to wait=w1292) -> ()  [unwired: 1 out]
              }
              frame #6 {
                n781 = VISA Write(VISA resource name=w1299, write buffer=w1297, error in (no error)=w1296) -> (VISA resource name out=w1298:refnum<visa-resource-name>, error out=w1295:errorcluster)  [unwired: 1 out]
              }
              frame #7 {
                n782 = Wait (ms)(milliseconds to wait=w1300) -> ()  [unwired: 1 out]
              }
              frame #8 {
                n783 = Concatenate Strings("start ", "\r") -> (w1307:string)
                n784 = VISA Write(VISA resource name=w1309, write buffer=w1307, error in (no error)=w1308) -> (VISA resource name out=w1304:refnum<visa-resource-name>, error out=w1303:errorcluster)  [unwired: 1 out]
              }
              frame #9 {
                n785 = Wait (ms)(milliseconds to wait=w1310) -> ()  [unwired: 1 out]
              }
              frame #10 {
                n786 = local write "Flush Pump 2"(FALSE ("Flush Pump 1")) -> ()
                n787 = Concatenate Strings("enter main ", "\r") -> (w1317:string)
                n788 = VISA Write(VISA resource name=w1316, write buffer=w1317, error in (no error)=w1315) -> (VISA resource name out=w1314:refnum<visa-resource-name>, error out=w1313:errorcluster)  [unwired: 1 out]
                n789 = VISA Close(VISA resource name=w1314, error in (no error)=w1313) -> ()  [unwired: 1 out]
              }
            }
            n790 = Concatenate Strings("set units 4 ", w1237) -> (w1250:string)
            n791 = Multiply(x="Flush \nRate (ul/min)  2", y=60) -> (x*y=w1248:dbl)
            n792 = Number To Decimal String(number=w1248) -> (decimal integer string=w1251:string)  [unwired: 1 in]
            n793 = Concatenate Strings("set rate ", w1251, w1237) -> (w1253:string)
            n794 = Number To Decimal String(number="Flush\nVolume (ul)  2") -> (decimal integer string=w1255:string)  [unwired: 1 in]
            n795 = Concatenate Strings("set volume ", w1255, w1237) -> (w1256:string)
          }
          event "Stop": Value Change {
            n796 = event-data() -> ()  [unwired: 1 in, 5 out]
            n797 = local read "Stop"() -> (w1321:bool)
          }
          event "Inject Pump 2": Value Change {
            n798 = event-data() -> ()  [unwired: 1 in, 5 out]
            n799 = case shown="True" "Inject Pump 2" {
              tunnel: w1322 -> [w1325 w1367]
              frame False {
                n800 = local read "Write Wait"() -> (w1324:i32)
                n801 = call-poly "VISA Configure Serial Port"("VISA resource name"=w1325) -> ("VISA resource name out"=w1329:refnum<visa-resource-name>, "error out"=w1330:errorcluster)  [unwired: 13 in]
                n802 = Concatenate Strings("enter pump2", "\r") -> (w1327:string)
                n803 = flat-sequence {
                  tunnel: w1330 -> [w1341]
                  tunnel: w1329 -> [w1343]
                  tunnel: [w1342] -> w1338
                  tunnel: [w1340] -> w1337
                  tunnel: w1327 -> [w1339]
                  tunnel: w1338 -> [w1346]
                  tunnel: w1337 -> [w1345]
                  tunnel: [w1346] -> w1336
                  tunnel: [w1345] -> w1335
                  tunnel: w1324 -> [w1344]
                  tunnel: [w1350] -> w1334
                  tunnel: [w1349] -> w1333
                  tunnel: w1336 -> [w1348]
                  tunnel: w1335 -> [w1347]
                  tunnel: w1334 -> [w1356]
                  tunnel: [w1356] -> w1332
                  tunnel: w1333 -> [w1355]
                  tunnel: [w1355] -> w1331
                  tunnel: w1324 -> [w1354]
                  tunnel: w1332 -> [w1360]
                  tunnel: w1331 -> [w1359]
                  frame #0 {
                    n804 = VISA Write(VISA resource name=w1343, write buffer=w1339, error in (no error)=w1341) -> (VISA resource name out=w1342:refnum<visa-resource-name>, error out=w1340:errorcluster)  [unwired: 1 out]
                  }
                  frame #1 {
                    n805 = Wait (ms)(milliseconds to wait=w1344) -> ()  [unwired: 1 out]
                  }
                  frame #2 {
                    n806 = Concatenate Strings("stop ", "\r") -> (w1353:string)
                    n807 = VISA Write(VISA resource name=w1348, write buffer=w1353, error in (no error)=w1347) -> (VISA resource name out=w1350:refnum<visa-resource-name>, error out=w1349:errorcluster)  [unwired: 1 out]
                  }
                  frame #3 {
                    n808 = Wait (ms)(milliseconds to wait=w1354) -> ()  [unwired: 1 out]
                  }
                  frame #4 {
                    n809 = Concatenate Strings("enter main ", "\r") -> (w1361:string)
                    n810 = VISA Write(VISA resource name=w1360, write buffer=w1361, error in (no error)=w1359) -> (VISA resource name out=w1358:refnum<visa-resource-name>, error out=w1357:errorcluster)  [unwired: 1 out]
                    n811 = VISA Close(VISA resource name=w1358, error in (no error)=w1357) -> ()  [unwired: 1 out]
                  }
                }
              }
              frame True {
                w1380 = "\r"
                n812 = call-poly "VISA Configure Serial Port"("VISA resource name"=w1367) -> ("VISA resource name out"=w1369:refnum<visa-resource-name>, "error out"=w1368:errorcluster)  [unwired: 13 in]
                n813 = local read "Write Wait"() -> (w1364:i32)
                n814 = Concatenate Strings("enter pump2", w1380) -> (w1379:string)
                n815 = flat-sequence {
                  tunnel: w1368 -> [w1403]
                  tunnel: w1369 -> [w1405]
                  tunnel: [w1404] -> w1400
                  tunnel: [w1402] -> w1399
                  tunnel: w1379 -> [w1401]
                  tunnel: w1400 -> [w1408]
                  tunnel: [w1408] -> w1398
                  tunnel: w1399 -> [w1407]
                  tunnel: [w1407] -> w1397
                  tunnel: w1364 -> [w1406]
                  tunnel: [w1413] -> w1396
                  tunnel: w1376 -> [w1412]
                  tunnel: [w1409] -> w1395
                  tunnel: w1398 -> [w1411]
                  tunnel: w1397 -> [w1410]
                  tunnel: w1396 -> [w1416]
                  tunnel: [w1416] -> w1394
                  tunnel: [w1415] -> w1393
                  tunnel: w1395 -> [w1415]
                  tunnel: w1364 -> [w1414]
                  tunnel: w1394 -> [w1421]
                  tunnel: [w1420] -> w1392
                  tunnel: w1373 -> [w1419]
                  tunnel: w1393 -> [w1418]
                  tunnel: [w1417] -> w1391
                  tunnel: w1392 -> [w1424]
                  tunnel: [w1424] -> w1390
                  tunnel: [w1423] -> w1389
                  tunnel: w1391 -> [w1423]
                  tunnel: w1364 -> [w1422]
                  tunnel: w1390 -> [w1429]
                  tunnel: [w1428] -> w1388
                  tunnel: w1370 -> [w1427]
                  tunnel: w1389 -> [w1426]
                  tunnel: [w1425] -> w1387
                  tunnel: [w1432] -> w1386
                  tunnel: w1388 -> [w1432]
                  tunnel: [w1431] -> w1385
                  tunnel: w1387 -> [w1431]
                  tunnel: w1364 -> [w1430]
                  tunnel: w1386 -> [w1439]
                  tunnel: w1385 -> [w1438]
                  tunnel: [w1434] -> w1384
                  tunnel: [w1433] -> w1383
                  tunnel: w1384 -> [w1442]
                  tunnel: [w1442] -> w1382
                  tunnel: w1383 -> [w1441]
                  tunnel: [w1441] -> w1381
                  tunnel: w1364 -> [w1440]
                  tunnel: w1382 -> [w1446]
                  tunnel: w1381 -> [w1445]
                  frame #0 {
                    n816 = VISA Write(VISA resource name=w1405, write buffer=w1401, error in (no error)=w1403) -> (VISA resource name out=w1404:refnum<visa-resource-name>, error out=w1402:errorcluster)  [unwired: 1 out]
                  }
                  frame #1 {
                    n817 = Wait (ms)(milliseconds to wait=w1406) -> ()  [unwired: 1 out]
                  }
                  frame #2 {
                    n818 = VISA Write(VISA resource name=w1411, write buffer=w1412, error in (no error)=w1410) -> (VISA resource name out=w1413:refnum<visa-resource-name>, error out=w1409:errorcluster)  [unwired: 1 out]
                  }
                  frame #3 {
                    n819 = Wait (ms)(milliseconds to wait=w1414) -> ()  [unwired: 1 out]
                  }
                  frame #4 {
                    n820 = VISA Write(VISA resource name=w1421, write buffer=w1419, error in (no error)=w1418) -> (VISA resource name out=w1420:refnum<visa-resource-name>, error out=w1417:errorcluster)  [unwired: 1 out]
                  }
                  frame #5 {
                    n821 = Wait (ms)(milliseconds to wait=w1422) -> ()  [unwired: 1 out]
                  }
                  frame #6 {
                    n822 = VISA Write(VISA resource name=w1429, write buffer=w1427, error in (no error)=w1426) -> (VISA resource name out=w1428:refnum<visa-resource-name>, error out=w1425:errorcluster)  [unwired: 1 out]
                  }
                  frame #7 {
                    n823 = Wait (ms)(milliseconds to wait=w1430) -> ()  [unwired: 1 out]
                  }
                  frame #8 {
                    n824 = Concatenate Strings("start ", "\r") -> (w1437:string)
                    n825 = VISA Write(VISA resource name=w1439, write buffer=w1437, error in (no error)=w1438) -> (VISA resource name out=w1434:refnum<visa-resource-name>, error out=w1433:errorcluster)  [unwired: 1 out]
                  }
                  frame #9 {
                    n826 = Wait (ms)(milliseconds to wait=w1440) -> ()  [unwired: 1 out]
                  }
                  frame #10 {
                    n827 = Concatenate Strings("enter main ", "\r") -> (w1447:string)
                    n828 = VISA Write(VISA resource name=w1446, write buffer=w1447, error in (no error)=w1445) -> (VISA resource name out=w1444:refnum<visa-resource-name>, error out=w1443:errorcluster)  [unwired: 1 out]
                    n829 = VISA Close(VISA resource name=w1444, error in (no error)=w1443) -> ()  [unwired: 1 out]
                  }
                }
                n830 = local read "Normal \nRate (ul/hr)  2"() -> (w1365:dbl)
                n831 = Concatenate Strings("set units 4 ", w1380) -> (w1376:string)
                n832 = local read "Normal \nVolume (ul) 2"() -> (w1366:dbl)
                n833 = Number To Decimal String(number=w1365) -> (decimal integer string=w1375:string)  [unwired: 1 in]
                n834 = Concatenate Strings("set rate ", w1375, w1380) -> (w1373:string)
                n835 = Number To Decimal String(number=w1366) -> (decimal integer string=w1371:string)  [unwired: 1 in]
                n836 = Concatenate Strings("set volume ", w1371, w1380) -> (w1370:string)
              }
            }
          }
          event "Inject Pump 1": Value Change {
            n837 = event-data() -> ()  [unwired: 1 in, 5 out]
            n838 = case shown="True" "Inject Pump 1" {
              tunnel: w1450 -> [w1453 w1495]
              frame False {
                n839 = local read "Write Wait"() -> (w1452:i32)
                n840 = call-poly "VISA Configure Serial Port"("VISA resource name"=w1453) -> ("VISA resource name out"=w1457:refnum<visa-resource-name>, "error out"=w1458:errorcluster)  [unwired: 13 in]
                n841 = Concatenate Strings("enter pump1", "\r") -> (w1455:string)
                n842 = flat-sequence {
                  tunnel: w1458 -> [w1469]
                  tunnel: w1457 -> [w1471]
                  tunnel: [w1470] -> w1466
                  tunnel: [w1468] -> w1465
                  tunnel: w1455 -> [w1467]
                  tunnel: w1466 -> [w1474]
                  tunnel: w1465 -> [w1473]
                  tunnel: [w1474] -> w1464
                  tunnel: [w1473] -> w1463
                  tunnel: w1452 -> [w1472]
                  tunnel: [w1478] -> w1462
                  tunnel: [w1477] -> w1461
                  tunnel: w1464 -> [w1476]
                  tunnel: w1463 -> [w1475]
                  tunnel: w1462 -> [w1484]
                  tunnel: [w1484] -> w1460
                  tunnel: w1461 -> [w1483]
                  tunnel: [w1483] -> w1459
                  tunnel: w1452 -> [w1482]
                  tunnel: w1460 -> [w1488]
                  tunnel: w1459 -> [w1487]
                  frame #0 {
                    n843 = VISA Write(VISA resource name=w1471, write buffer=w1467, error in (no error)=w1469) -> (VISA resource name out=w1470:refnum<visa-resource-name>, error out=w1468:errorcluster)  [unwired: 1 out]
                  }
                  frame #1 {
                    n844 = Wait (ms)(milliseconds to wait=w1472) -> ()  [unwired: 1 out]
                  }
                  frame #2 {
                    n845 = Concatenate Strings("stop ", "\r") -> (w1481:string)
                    n846 = VISA Write(VISA resource name=w1476, write buffer=w1481, error in (no error)=w1475) -> (VISA resource name out=w1478:refnum<visa-resource-name>, error out=w1477:errorcluster)  [unwired: 1 out]
                  }
                  frame #3 {
                    n847 = Wait (ms)(milliseconds to wait=w1482) -> ()  [unwired: 1 out]
                  }
                  frame #4 {
                    n848 = Concatenate Strings("enter main ", "\r") -> (w1489:string)
                    n849 = VISA Write(VISA resource name=w1488, write buffer=w1489, error in (no error)=w1487) -> (VISA resource name out=w1486:refnum<visa-resource-name>, error out=w1485:errorcluster)  [unwired: 1 out]
                    n850 = VISA Close(VISA resource name=w1486, error in (no error)=w1485) -> ()  [unwired: 1 out]
                  }
                }
              }
              frame True {
                w1508 = "\r"
                n851 = call-poly "VISA Configure Serial Port"("VISA resource name"=w1495) -> ("VISA resource name out"=w1497:refnum<visa-resource-name>, "error out"=w1496:errorcluster)  [unwired: 13 in]
                n852 = local read "Write Wait"() -> (w1492:i32)
                n853 = flat-sequence {
                  tunnel: w1496 -> [w1531]
                  tunnel: w1497 -> [w1533]
                  tunnel: [w1532] -> w1528
                  tunnel: [w1530] -> w1527
                  tunnel: w1507 -> [w1529]
                  tunnel: w1528 -> [w1536]
                  tunnel: [w1536] -> w1526
                  tunnel: w1527 -> [w1535]
                  tunnel: [w1535] -> w1525
                  tunnel: w1492 -> [w1534]
                  tunnel: [w1541] -> w1524
                  tunnel: w1504 -> [w1540]
                  tunnel: [w1537] -> w1523
                  tunnel: w1526 -> [w1539]
                  tunnel: w1525 -> [w1538]
                  tunnel: w1524 -> [w1544]
                  tunnel: [w1544] -> w1522
                  tunnel: [w1543] -> w1521
                  tunnel: w1523 -> [w1543]
                  tunnel: w1492 -> [w1542]
                  tunnel: w1522 -> [w1549]
                  tunnel: [w1548] -> w1520
                  tunnel: w1501 -> [w1547]
                  tunnel: w1521 -> [w1546]
                  tunnel: [w1545] -> w1519
                  tunnel: w1520 -> [w1552]
                  tunnel: [w1552] -> w1518
                  tunnel: [w1551] -> w1517
                  tunnel: w1519 -> [w1551]
                  tunnel: w1492 -> [w1550]
                  tunnel: w1518 -> [w1557]
                  tunnel: [w1556] -> w1516
                  tunnel: w1498 -> [w1555]
                  tunnel: w1517 -> [w1554]
                  tunnel: [w1553] -> w1515
                  tunnel: [w1560] -> w1514
                  tunnel: w1516 -> [w1560]
                  tunnel: [w1559] -> w1513
                  tunnel: w1515 -> [w1559]
                  tunnel: w1492 -> [w1558]
                  tunnel: w1514 -> [w1567]
                  tunnel: w1513 -> [w1566]
                  tunnel: [w1562] -> w1512
                  tunnel: [w1561] -> w1511
                  tunnel: w1512 -> [w1570]
                  tunnel: [w1570] -> w1510
                  tunnel: w1511 -> [w1569]
                  tunnel: [w1569] -> w1509
                  tunnel: w1492 -> [w1568]
                  tunnel: w1510 -> [w1574]
                  tunnel: w1509 -> [w1573]
                  frame #0 {
                    n854 = VISA Write(VISA resource name=w1533, write buffer=w1529, error in (no error)=w1531) -> (VISA resource name out=w1532:refnum<visa-resource-name>, error out=w1530:errorcluster)  [unwired: 1 out]
                  }
                  frame #1 {
                    n855 = Wait (ms)(milliseconds to wait=w1534) -> ()  [unwired: 1 out]
                  }
                  frame #2 {
                    n856 = VISA Write(VISA resource name=w1539, write buffer=w1540, error in (no error)=w1538) -> (VISA resource name out=w1541:refnum<visa-resource-name>, error out=w1537:errorcluster)  [unwired: 1 out]
                  }
                  frame #3 {
                    n857 = Wait (ms)(milliseconds to wait=w1542) -> ()  [unwired: 1 out]
                  }
                  frame #4 {
                    n858 = VISA Write(VISA resource name=w1549, write buffer=w1547, error in (no error)=w1546) -> (VISA resource name out=w1548:refnum<visa-resource-name>, error out=w1545:errorcluster)  [unwired: 1 out]
                  }
                  frame #5 {
                    n859 = Wait (ms)(milliseconds to wait=w1550) -> ()  [unwired: 1 out]
                  }
                  frame #6 {
                    n860 = VISA Write(VISA resource name=w1557, write buffer=w1555, error in (no error)=w1554) -> (VISA resource name out=w1556:refnum<visa-resource-name>, error out=w1553:errorcluster)  [unwired: 1 out]
                  }
                  frame #7 {
                    n861 = Wait (ms)(milliseconds to wait=w1558) -> ()  [unwired: 1 out]
                  }
                  frame #8 {
                    n862 = Concatenate Strings("start ", "\r") -> (w1565:string)
                    n863 = VISA Write(VISA resource name=w1567, write buffer=w1565, error in (no error)=w1566) -> (VISA resource name out=w1562:refnum<visa-resource-name>, error out=w1561:errorcluster)  [unwired: 1 out]
                  }
                  frame #9 {
                    n864 = Wait (ms)(milliseconds to wait=w1568) -> ()  [unwired: 1 out]
                  }
                  frame #10 {
                    n865 = Concatenate Strings("enter main ", "\r") -> (w1575:string)
                    n866 = VISA Write(VISA resource name=w1574, write buffer=w1575, error in (no error)=w1573) -> (VISA resource name out=w1572:refnum<visa-resource-name>, error out=w1571:errorcluster)  [unwired: 1 out]
                    n867 = VISA Close(VISA resource name=w1572, error in (no error)=w1571) -> ()  [unwired: 1 out]
                  }
                }
                n868 = Concatenate Strings("enter pump1", w1508) -> (w1507:string)
                n869 = local read "Normal \nRate (ul/hr)"() -> (w1493:dbl)
                n870 = Concatenate Strings("set units 4 ", w1508) -> (w1504:string)
                n871 = local read "Normal \nVolume (ul)"() -> (w1494:dbl)
                n872 = Number To Decimal String(number=w1493) -> (decimal integer string=w1503:string)  [unwired: 1 in]
                n873 = Concatenate Strings("set rate ", w1503, w1508) -> (w1501:string)
                n874 = Number To Decimal String(number=w1494) -> (decimal integer string=w1499:string)  [unwired: 1 in]
                n875 = Concatenate Strings("set volume ", w1499, w1508) -> (w1498:string)
              }
            }
          }
          event "Normal \nVolume (ul)": Value Change {
            n876 = event-data() -> ()  [unwired: 1 in, 5 out]
            n877 = call-poly "VISA Configure Serial Port"("VISA resource name"=w1593) -> ("VISA resource name out"=w1595:refnum<visa-resource-name>, "error out"=w1594:errorcluster)  [unwired: 13 in]
            n878 = local read "Write Wait"() -> (w1578:i32)
            n879 = Concatenate Strings("enter pump1", "\r") -> (w1597:string)
            n880 = flat-sequence {
              tunnel: w1594 -> [w1607]
              tunnel: w1595 -> [w1609]
              tunnel: [w1608] -> w1587
              tunnel: [w1606] -> w1586
              tunnel: w1597 -> [w1605]
              tunnel: w1587 -> [w1612]
              tunnel: [w1612] -> w1585
              tunnel: w1586 -> [w1611]
              tunnel: [w1611] -> w1583
              tunnel: w1578 -> [w1610]
              tunnel: w1585 -> [w1616]
              tunnel: [w1617] -> w1584
              tunnel: w1583 -> [w1615]
              tunnel: [w1614] -> w1582
              tunnel: w1579 -> [w1613]
              tunnel: w1584 -> [w1620]
              tunnel: w1582 -> [w1619]
              tunnel: [w1620] -> w1604
              tunnel: [w1619] -> w1603
              tunnel: w1578 -> [w1618]
              tunnel: [w1625] -> w1602
              tunnel: [w1624] -> w1601
              tunnel: w1604 -> [w1623]
              tunnel: w1603 -> [w1622]
              tunnel: w1588 -> [w1621]
              tunnel: w1602 -> [w1628]
              tunnel: [w1628] -> w1600
              tunnel: w1601 -> [w1627]
              tunnel: [w1627] -> w1599
              tunnel: w1578 -> [w1626]
              tunnel: w1600 -> [w1632]
              tunnel: w1599 -> [w1631]
              frame #0 {
                n881 = VISA Write(VISA resource name=w1609, write buffer=w1605, error in (no error)=w1607) -> (VISA resource name out=w1608:refnum<visa-resource-name>, error out=w1606:errorcluster)  [unwired: 1 out]
              }
              frame #1 {
                n882 = Wait (ms)(milliseconds to wait=w1610) -> ()  [unwired: 1 out]
              }
              frame #2 {
                n883 = VISA Write(VISA resource name=w1616, write buffer=w1613, error in (no error)=w1615) -> (VISA resource name out=w1617:refnum<visa-resource-name>, error out=w1614:errorcluster)  [unwired: 1 out]
              }
              frame #3 {
                n884 = Wait (ms)(milliseconds to wait=w1618) -> ()  [unwired: 1 out]
              }
              frame #4 {
                n885 = VISA Write(VISA resource name=w1623, write buffer=w1621, error in (no error)=w1622) -> (VISA resource name out=w1625:refnum<visa-resource-name>, error out=w1624:errorcluster)  [unwired: 1 out]
              }
              frame #5 {
                n886 = Wait (ms)(milliseconds to wait=w1626) -> ()  [unwired: 1 out]
              }
              frame #6 {
                n887 = Concatenate Strings("enter main ", "\r") -> (w1633:string)
                n888 = VISA Write(VISA resource name=w1632, write buffer=w1633, error in (no error)=w1631) -> (VISA resource name out=w1630:refnum<visa-resource-name>, error out=w1629:errorcluster)  [unwired: 1 out]
                n889 = VISA Close(VISA resource name=w1630, error in (no error)=w1629) -> ()  [unwired: 1 out]
              }
            }
            n890 = Concatenate Strings("set units 4", "\r") -> (w1579:string)
            n891 = Number To Decimal String(number="Normal \nVolume (ul)") -> (decimal integer string=w1590:string)  [unwired: 1 in]
            n892 = Concatenate Strings("set volume", w1590, "\r") -> (w1588:string)
          }
          event "Normal \nRate (ul/hr)": Value Change {
            n893 = event-data() -> ()  [unwired: 1 in, 5 out]
            n894 = call-poly "VISA Configure Serial Port"("VISA resource name"=w1638) -> ("VISA resource name out"=w1646:refnum<visa-resource-name>, "error out"=w1645:errorcluster)  [unwired: 13 in]
            n895 = local read "Write Wait"() -> (w1636:i32)
            n896 = Concatenate Strings("enter pump1", "\r") -> (w1648:string)
            n897 = flat-sequence {
              tunnel: w1645 -> [w1665]
              tunnel: w1646 -> [w1667]
              tunnel: [w1666] -> w1661
              tunnel: [w1664] -> w1660
              tunnel: w1648 -> [w1663]
              tunnel: w1661 -> [w1670]
              tunnel: [w1670] -> w1659
              tunnel: w1660 -> [w1669]
              tunnel: [w1669] -> w1658
              tunnel: w1636 -> [w1668]
              tunnel: w1659 -> [w1674]
              tunnel: [w1675] -> w1657
              tunnel: w1658 -> [w1673]
              tunnel: [w1672] -> w1656
              tunnel: w1639 -> [w1671]
              tunnel: w1657 -> [w1678]
              tunnel: w1656 -> [w1677]
              tunnel: [w1678] -> w1655
              tunnel: [w1677] -> w1654
              tunnel: w1636 -> [w1676]
              tunnel: [w1683] -> w1653
              tunnel: [w1682] -> w1652
              tunnel: w1655 -> [w1681]
              tunnel: w1654 -> [w1680]
              tunnel: w1642 -> [w1679]
              tunnel: w1653 -> [w1686]
              tunnel: [w1686] -> w1651
              tunnel: w1652 -> [w1685]
              tunnel: [w1685] -> w1650
              tunnel: w1636 -> [w1684]
              tunnel: w1651 -> [w1690]
              tunnel: w1650 -> [w1689]
              frame #0 {
                n898 = VISA Write(VISA resource name=w1667, write buffer=w1663, error in (no error)=w1665) -> (VISA resource name out=w1666:refnum<visa-resource-name>, error out=w1664:errorcluster)  [unwired: 1 out]
              }
              frame #1 {
                n899 = Wait (ms)(milliseconds to wait=w1668) -> ()  [unwired: 1 out]
              }
              frame #2 {
                n900 = VISA Write(VISA resource name=w1674, write buffer=w1671, error in (no error)=w1673) -> (VISA resource name out=w1675:refnum<visa-resource-name>, error out=w1672:errorcluster)  [unwired: 1 out]
              }
              frame #3 {
                n901 = Wait (ms)(milliseconds to wait=w1676) -> ()  [unwired: 1 out]
              }
              frame #4 {
                n902 = VISA Write(VISA resource name=w1681, write buffer=w1679, error in (no error)=w1680) -> (VISA resource name out=w1683:refnum<visa-resource-name>, error out=w1682:errorcluster)  [unwired: 1 out]
              }
              frame #5 {
                n903 = Wait (ms)(milliseconds to wait=w1684) -> ()  [unwired: 1 out]
              }
              frame #6 {
                n904 = Concatenate Strings("enter main ", "\r") -> (w1691:string)
                n905 = VISA Write(VISA resource name=w1690, write buffer=w1691, error in (no error)=w1689) -> (VISA resource name out=w1688:refnum<visa-resource-name>, error out=w1687:errorcluster)  [unwired: 1 out]
                n906 = VISA Close(VISA resource name=w1688, error in (no error)=w1687) -> ()  [unwired: 1 out]
              }
            }
            n907 = Concatenate Strings("set units 4", "\r") -> (w1639:string)
            n908 = Number To Decimal String(number="Normal \nRate (ul/hr)") -> (decimal integer string=w1637:string)  [unwired: 1 in]
            n909 = Concatenate Strings("set rate", w1637, "\r") -> (w1642:string)
          }
          event "Normal \nRate (ul/hr)  2": Value Change {
            n910 = event-data() -> ()  [unwired: 1 in, 5 out]
            n911 = call-poly "VISA Configure Serial Port"("VISA resource name"=w1696) -> ("VISA resource name out"=w1704:refnum<visa-resource-name>, "error out"=w1703:errorcluster)  [unwired: 13 in]
            n912 = local read "Write Wait"() -> (w1694:i32)
            n913 = Concatenate Strings("enter pump2", "\r") -> (w1706:string)
            n914 = flat-sequence {
              tunnel: w1703 -> [w1723]
              tunnel: w1704 -> [w1725]
              tunnel: [w1724] -> w1719
              tunnel: [w1722] -> w1718
              tunnel: w1706 -> [w1721]
              tunnel: w1719 -> [w1728]
              tunnel: [w1728] -> w1717
              tunnel: w1718 -> [w1727]
              tunnel: [w1727] -> w1716
              tunnel: w1694 -> [w1726]
              tunnel: w1717 -> [w1732]
              tunnel: [w1733] -> w1715
              tunnel: w1716 -> [w1731]
              tunnel: [w1730] -> w1714
              tunnel: w1697 -> [w1729]
              tunnel: w1715 -> [w1736]
              tunnel: w1714 -> [w1735]
              tunnel: [w1736] -> w1713
              tunnel: [w1735] -> w1712
              tunnel: w1694 -> [w1734]
              tunnel: [w1741] -> w1711
              tunnel: [w1740] -> w1710
              tunnel: w1713 -> [w1739]
              tunnel: w1712 -> [w1738]
              tunnel: w1700 -> [w1737]
              tunnel: w1711 -> [w1744]
              tunnel: [w1744] -> w1709
              tunnel: w1710 -> [w1743]
              tunnel: [w1743] -> w1708
              tunnel: w1694 -> [w1742]
              tunnel: w1709 -> [w1748]
              tunnel: w1708 -> [w1747]
              frame #0 {
                n915 = VISA Write(VISA resource name=w1725, write buffer=w1721, error in (no error)=w1723) -> (VISA resource name out=w1724:refnum<visa-resource-name>, error out=w1722:errorcluster)  [unwired: 1 out]
              }
              frame #1 {
                n916 = Wait (ms)(milliseconds to wait=w1726) -> ()  [unwired: 1 out]
              }
              frame #2 {
                n917 = VISA Write(VISA resource name=w1732, write buffer=w1729, error in (no error)=w1731) -> (VISA resource name out=w1733:refnum<visa-resource-name>, error out=w1730:errorcluster)  [unwired: 1 out]
              }
              frame #3 {
                n918 = Wait (ms)(milliseconds to wait=w1734) -> ()  [unwired: 1 out]
              }
              frame #4 {
                n919 = VISA Write(VISA resource name=w1739, write buffer=w1737, error in (no error)=w1738) -> (VISA resource name out=w1741:refnum<visa-resource-name>, error out=w1740:errorcluster)  [unwired: 1 out]
              }
              frame #5 {
                n920 = Wait (ms)(milliseconds to wait=w1742) -> ()  [unwired: 1 out]
              }
              frame #6 {
                n921 = Concatenate Strings("enter main ", "\r") -> (w1749:string)
                n922 = VISA Write(VISA resource name=w1748, write buffer=w1749, error in (no error)=w1747) -> (VISA resource name out=w1746:refnum<visa-resource-name>, error out=w1745:errorcluster)  [unwired: 1 out]
                n923 = VISA Close(VISA resource name=w1746, error in (no error)=w1745) -> ()  [unwired: 1 out]
              }
            }
            n924 = Concatenate Strings("set units 4", "\r") -> (w1697:string)
            n925 = Number To Decimal String(number="Normal \nRate (ul/hr)  2") -> (decimal integer string=w1695:string)  [unwired: 1 in]
            n926 = Concatenate Strings("set rate", w1695, "\r") -> (w1700:string)
          }
          event "Normal \nVolume (ul) 2": Value Change {
            n927 = event-data() -> ()  [unwired: 1 in, 5 out]
            n928 = call-poly "VISA Configure Serial Port"("VISA resource name"=w1755) -> ("VISA resource name out"=w1759:refnum<visa-resource-name>, "error out"=w1760:errorcluster)  [unwired: 13 in]
            n929 = local read "Write Wait"() -> (w1752:i32)
            n930 = Concatenate Strings("enter pump2", "\r") -> (w1757:string)
            n931 = flat-sequence {
              tunnel: w1760 -> [w1781]
              tunnel: w1759 -> [w1783]
              tunnel: [w1782] -> w1778
              tunnel: [w1780] -> w1777
              tunnel: w1757 -> [w1779]
              tunnel: w1778 -> [w1786]
              tunnel: [w1786] -> w1776
              tunnel: w1777 -> [w1785]
              tunnel: [w1785] -> w1775
              tunnel: w1752 -> [w1784]
              tunnel: w1776 -> [w1790]
              tunnel: [w1791] -> w1774
              tunnel: w1775 -> [w1789]
              tunnel: [w1788] -> w1773
              tunnel: w1766 -> [w1787]
              tunnel: w1774 -> [w1794]
              tunnel: w1773 -> [w1793]
              tunnel: [w1794] -> w1772
              tunnel: [w1793] -> w1771
              tunnel: w1752 -> [w1792]
              tunnel: [w1799] -> w1770
              tunnel: [w1798] -> w1769
              tunnel: w1772 -> [w1797]
              tunnel: w1771 -> [w1796]
              tunnel: w1763 -> [w1795]
              tunnel: w1770 -> [w1802]
              tunnel: [w1802] -> w1768
              tunnel: w1769 -> [w1801]
              tunnel: [w1801] -> w1767
              tunnel: w1752 -> [w1800]
              tunnel: w1768 -> [w1806]
              tunnel: w1767 -> [w1805]
              frame #0 {
                n932 = VISA Write(VISA resource name=w1783, write buffer=w1779, error in (no error)=w1781) -> (VISA resource name out=w1782:refnum<visa-resource-name>, error out=w1780:errorcluster)  [unwired: 1 out]
              }
              frame #1 {
                n933 = Wait (ms)(milliseconds to wait=w1784) -> ()  [unwired: 1 out]
              }
              frame #2 {
                n934 = VISA Write(VISA resource name=w1790, write buffer=w1787, error in (no error)=w1789) -> (VISA resource name out=w1791:refnum<visa-resource-name>, error out=w1788:errorcluster)  [unwired: 1 out]
              }
              frame #3 {
                n935 = Wait (ms)(milliseconds to wait=w1792) -> ()  [unwired: 1 out]
              }
              frame #4 {
                n936 = VISA Write(VISA resource name=w1797, write buffer=w1795, error in (no error)=w1796) -> (VISA resource name out=w1799:refnum<visa-resource-name>, error out=w1798:errorcluster)  [unwired: 1 out]
              }
              frame #5 {
                n937 = Wait (ms)(milliseconds to wait=w1800) -> ()  [unwired: 1 out]
              }
              frame #6 {
                n938 = Concatenate Strings("enter main ", "\r") -> (w1807:string)
                n939 = VISA Write(VISA resource name=w1806, write buffer=w1807, error in (no error)=w1805) -> (VISA resource name out=w1804:refnum<visa-resource-name>, error out=w1803:errorcluster)  [unwired: 1 out]
                n940 = VISA Close(VISA resource name=w1804, error in (no error)=w1803) -> ()  [unwired: 1 out]
              }
            }
            n941 = Concatenate Strings("set units 4", "\r") -> (w1766:string)
            n942 = Number To Decimal String(number="Normal \nVolume (ul) 2") -> (decimal integer string=w1753:string)  [unwired: 1 in]
            n943 = Concatenate Strings("set volume", w1753, "\r") -> (w1763:string)
          }
        }
        n944 = node-c288() -> ()  [unwired: 1 in, 1 out]
      }
      n945 = node-c288(w1139) -> ()  [unwired: 1 out]
    }
    frame Enabled {
      n946 = node-c288(2 ("Processor")) -> (w1819:T12)  [unwired: 3 in]
      n947 = timed-loop "Pump Control" {
        timing: w1819 -> [_]
        timing-out: [_] -> w1818
        tunnel: refnum<visa-resource-name> "COM5" ("VISA resource name") -> [w1821]
        stop <- w1820 stop-if-true
        n948 = node-c288() -> ()  [unwired: 1 in, 1 out]
        n949 = event shown="[2] \"Inject Sample\": Value Change" {
          selector: _ -> [_ _ _ _ _]
          dyn-events: _ -> [_ _ _ _ _]
          timeout: _ -> [_ _ _ _ _]
          tunnel: w1821 -> [w1827 _ w1901 w1928 w1933]
          tunnel: [_ w1899 _ _ _] -> w1820
          event "Flush Sample": Value Change {
            n950 = event-data() -> ()  [unwired: 1 in, 5 out]
            n951 = local read "Write Wait"() -> (w1841:i32)
            n952 = flat-sequence {
              tunnel: [w1865] -> w1861
              tunnel: [w1864] -> w1860
              tunnel: "CLD" -> [w1863]
              tunnel: w1827 -> [w1862]
              tunnel: w1861 -> [w1868]
              tunnel: [w1868] -> w1859
              tunnel: w1860 -> [w1867]
              tunnel: [w1867] -> w1858
              tunnel: w1841 -> [w1866]
              tunnel: [w1873] -> w1857
              tunnel: [w1870] -> w1856
              tunnel: w1859 -> [w1872]
              tunnel: w1858 -> [w1871]
              tunnel: "MODVOL" -> [w1869]
              tunnel: w1857 -> [w1876]
              tunnel: [w1876] -> w1855
              tunnel: [w1875] -> w1854
              tunnel: w1856 -> [w1875]
              tunnel: w1841 -> [w1874]
              tunnel: w1855 -> [w1881]
              tunnel: [w1880] -> w1853
              tunnel: w1843 -> [w1879]
              tunnel: w1854 -> [w1878]
              tunnel: [w1877] -> w1852
              tunnel: w1853 -> [w1884]
              tunnel: [w1884] -> w1851
              tunnel: [w1883] -> w1850
              tunnel: w1852 -> [w1883]
              tunnel: w1841 -> [w1882]
              tunnel: w1851 -> [w1889]
              tunnel: [w1888] -> w1849
              tunnel: w1845 -> [w1887]
              tunnel: w1850 -> [w1886]
              tunnel: [w1885] -> w1848
              tunnel: [w1892] -> w1846
              tunnel: w1849 -> [w1892]
              tunnel: [w1891] -> w1847
              tunnel: w1848 -> [w1891]
              tunnel: w1841 -> [w1890]
              tunnel: w1847 -> [w1897]
              tunnel: w1846 -> [w1898]
              tunnel: [w1896] -> w1836
              tunnel: "RUN " -> [w1895]
              frame #0 {
                n953 = call "Write to pump 2.vi"("String to write"=w1863, "VISA resource name"=w1862) -> ("error out"=w1864:errorcluster, "VISA resource name out"=w1865:refnum<visa-resource-name>)  [unwired: 8 in]
              }
              frame #1 {
                n954 = Wait (ms)(milliseconds to wait=w1866) -> ()  [unwired: 1 out]
              }
              frame #2 {
                n955 = call "Write to pump 2.vi"("error in (no error)"=w1871, "String to write"=w1869, "VISA resource name"=w1872) -> ("error out"=w1870:errorcluster, "VISA resource name out"=w1873:refnum<visa-resource-name>)  [unwired: 7 in]
              }
              frame #3 {
                n956 = Wait (ms)(milliseconds to wait=w1874) -> ()  [unwired: 1 out]
              }
              frame #4 {
                n957 = call "Write to pump 2.vi"("error in (no error)"=w1878, "String to write"=w1879, "VISA resource name"=w1881) -> ("error out"=w1877:errorcluster, "VISA resource name out"=w1880:refnum<visa-resource-name>)  [unwired: 7 in]
              }
              frame #5 {
                n958 = Wait (ms)(milliseconds to wait=w1882) -> ()  [unwired: 1 out]
              }
              frame #6 {
                n959 = call "Write to pump 2.vi"("error in (no error)"=w1886, "String to write"=w1887, "VISA resource name"=w1889) -> ("error out"=w1885:errorcluster, "VISA resource name out"=w1888:refnum<visa-resource-name>)  [unwired: 7 in]
              }
              frame #7 {
                n960 = Wait (ms)(milliseconds to wait=w1890) -> ()  [unwired: 1 out]
              }
              frame #8 {
                w1894 = TRUE ("Inject Pump 3")
                n961 = Tick Count (ms)() -> (millisecond timer value=→"Flush Sample Start Time":u32)
                n962 = call "Write to pump 2.vi"("error in (no error)"=w1897, "String to write"=w1895, "VISA resource name"=w1898) -> ("error out"=w1896:errorcluster)  [unwired: 7 in, 1 out]
                n963 = local write "Inject Sample"(w1894) -> ()
                "Flushing Sample" <- w1894
              }
            }
            n964 = Number To Fractional String(number="Flush \nRate (ul/min)  3") -> (F-format string=w1829:string)  [unwired: 3 in]
            n965 = String Subset(string=w1829, length (rest)=6 ("length (rest)")) -> (substring=w1828:string)  [unwired: 1 in]
            n966 = Concatenate Strings("RAT", w1828, "UM") -> (w1843:string)
            n967 = Divide(x="Flush\nVolume (ul)  3", y=1000.0) -> (x/y=w1834:dbl)
            n968 = Number To Fractional String(number=w1834) -> (F-format string=w1833:string)  [unwired: 3 in]
            n969 = Divide(x="Flush\nVolume (ul)  3", y="Flush \nRate (ul/min)  3") -> (x/y=w1824:dbl)
            n970 = Multiply(x=w1824, y=60.0) -> (x*y=→"Sample flush time (s)":dbl)
            n971 = String Subset(string=w1833, length (rest)=6 ("length (rest)")) -> (substring=w1832:string)  [unwired: 1 in]
            n972 = Concatenate Strings("TGT", w1832) -> (w1845:string)
            "error out" <- w1836
          }
          event "Stop": Value Change {
            n973 = event-data() -> ()  [unwired: 1 in, 5 out]
            n974 = local read "Stop"() -> (w1899:bool)
          }
          event "Inject Sample": Value Change {
            n975 = event-data() -> ()  [unwired: 1 in, 5 out]
            n976 = case shown="True" "Inject Sample" {
              tunnel: w1901 -> [w1903 w1904]
              frame False {
                n977 = call "Write to pump 2.vi"("String to write"="STP", "VISA resource name"=w1903) -> ()  [unwired: 8 in, 2 out]
              }
              frame True {
                n978 = local read "Normal \nRate (ul/hr)  3"() -> (w1905:dbl)
                n979 = Number To Fractional String(number=w1905) -> (F-format string=w1908:string)  [unwired: 3 in]
                n980 = String Subset(string=w1908, length (rest)=6 ("length (rest)")) -> (substring=w1906:string)  [unwired: 1 in]
                n981 = flat-sequence {
                  tunnel: "RUN " -> [w1920]
                  tunnel: [w1922] -> _
                  tunnel: [w1921] -> _
                  tunnel: w1904 -> [w1919]
                  frame #0 {
                    n982 = call "Write to pump 2.vi"("String to write"=w1920, "VISA resource name"=w1919) -> ("error out"=w1921:errorcluster, "VISA resource name out"=w1922:refnum<visa-resource-name>)  [unwired: 8 in]
                  }
                }
                n983 = Concatenate Strings("RAT", w1906, "UH" ("string")) -> ()  [unwired: 1 out]
                n984 = local read "Normal \nVolume (ul) 3"() -> (w1914:dbl)
                n985 = Divide(x=w1914, y=1000.0) -> (x/y=w1909:dbl)
                n986 = Number To Fractional String(number=w1909) -> (F-format string=w1912:string)  [unwired: 3 in]
                n987 = String Subset(string=w1912, length (rest)=6 ("length (rest)")) -> (substring=w1910:string)  [unwired: 1 in]
                n988 = Concatenate Strings("TGT", w1910) -> ()  [unwired: 1 out]
              }
            }
          }
          event "Normal \nRate (ul/hr)  3": Value Change {
            n989 = event-data() -> ()  [unwired: 1 in, 5 out]
            n990 = Number To Fractional String(number="Normal \nRate (ul/hr)  3") -> (F-format string=w1926:string)  [unwired: 3 in]
            n991 = String Subset(string=w1926, length (rest)=6 ("length (rest)")) -> (substring=w1924:string)  [unwired: 1 in]
            n992 = Concatenate Strings("RAT", w1924, "UH") -> (w1927:string)
            n993 = call "Write to pump 2.vi"("String to write"=w1927, "VISA resource name"=w1928) -> ()  [unwired: 8 in, 2 out]
          }
          event "Clear Volume": Value Change {
            n994 = event-data() -> ()  [unwired: 1 in, 5 out]
            n995 = Divide(x="Normal \nVolume (ul) 3", y=1000.0) -> (x/y=w1946:dbl)
            n996 = Number To Fractional String(number=w1946) -> (F-format string=w1949:string)  [unwired: 3 in]
            n997 = String Subset(string=w1949, length (rest)=6 ("length (rest)")) -> (substring=w1947:string)  [unwired: 1 in]
            n998 = flat-sequence {
              tunnel: [w1956] -> w1944
              tunnel: [w1955] -> w1943
              tunnel: w1933 -> [w1954]
              tunnel: w1932 -> [w1953]
              tunnel: [w1958] -> w1941
              tunnel: [w1957] -> w1942
              tunnel: w1938 -> [w1959]
              tunnel: w1944 -> [w1958]
              tunnel: w1943 -> [w1957]
              tunnel: w1942 -> [w1963]
              tunnel: w1941 -> [w1964]
              tunnel: [w1962] -> _
              tunnel: [w1961] -> _
              tunnel: w1931 -> [w1960]
              frame #0 {
                n999 = call "Write to pump 2.vi"("String to write"=w1953, "VISA resource name"=w1954) -> ("error out"=w1955:errorcluster, "VISA resource name out"=w1956:refnum<visa-resource-name>)  [unwired: 8 in]
              }
              frame #1 {
                n1000 = Wait (ms)(milliseconds to wait=w1959) -> ()  [unwired: 1 out]
              }
              frame #2 {
                n1001 = call "Write to pump 2.vi"("error in (no error)"=w1963, "String to write"=w1960, "VISA resource name"=w1964) -> ("error out"=w1961:errorcluster, "VISA resource name out"=w1962:refnum<visa-resource-name>)  [unwired: 7 in]
              }
            }
            n1002 = local read "Write Wait"() -> (w1938:i32)
            n1003 = Concatenate Strings("TGT", w1947) -> (w1932:string)
            n1004 = local read "Normal \nRate (ul/hr)  3"() -> (w1934:dbl)
            n1005 = local write "Clear Volume"(FALSE ("Clear Volume")) -> ()
            n1006 = Number To Fractional String(number=w1934) -> (F-format string=w1937:string)  [unwired: 3 in]
            n1007 = String Subset(string=w1937, length (rest)=6 ("length (rest)")) -> (substring=w1935:string)  [unwired: 1 in]
            n1008 = Concatenate Strings("RAT", w1935, "UH" ("string")) -> (w1931:string)
          }
        }
        n1009 = node-c288() -> ()  [unwired: 1 in, 1 out]
      }
      n1010 = node-c288(w1818) -> ()  [unwired: 1 out]
    }
  }
  n1011 = local write "Tether"(FALSE ("Tether")) -> ()
  n1012 = local read "Path"() -> (w81:path)
  n1013 = node-c288(i64 50 ("Period"), 2 ("Processor")) -> (w87:T12)  [unwired: 2 in]
  n1014 = VISA Close(VISA resource name=w19) -> (error out=w104:errorcluster)  [unwired: 1 in]
  n1015 = timed-loop {
    timing: w87 -> [_]
    timing-out: [_] -> w86
    tunnel: w81 -> [w1972]
    stop <- w1971 stop-if-true
    n1016 = node-c288() -> ()  [unwired: 1 in, 1 out]
    n1017 = event shown="[5] \"Raster scan\": Value Change" {
      selector: _ -> [_ _ _ _ _ _ _ _ _]
      dyn-events: _ -> [_ _ _ _ _ _ _ _ _]
      timeout: _ -> [_ _ _ _ _ _ _ _ _]
      tunnel: w1972 -> [_ w1976 _ _ _ _ _ _ _]
      tunnel: [_ _ w1996 _ _ _ _ _ _] -> w1971
      event Timeout {
        n1018 = event-data() -> ()  [unwired: 1 in, 2 out]
      }
      event "Read Cal": Value Change {
        n1019 = event-data() -> ()  [unwired: 1 in, 6 out]
        n1020 = Path To String(path=w1976) -> (string=w1975:string)
        n1021 = Format Date/Time String(time format string (%c)="%y%m%d") -> (date/time string=w1977:string)  [unwired: 2 in]
        n1022 = Concatenate Strings(w1975, "\\" ("string"), w1977, "\\" ("string"), "current.cal") -> (w1995:string)
        n1023 = String To Path(string=w1995) -> (path=w1994:path)
        n1024 = Open/Create/Replace File(file path (use dialog)=w1994, operation (0:open)=T9."open", access (0:read/write)=enum16{"read/write", "read-only", "write-only"}."read-only") -> (refnum out=w1990:refnum<file>, error out=w1991:errorcluster)  [unwired: 3 in, 1 out]
        n1025 = Deny Access(4:w1991, 7:w1990) -> (0:w1989:errorcluster, 3:w1988:refnum<file>)  [unwired: 1 in]
        n1026 = Read from Binary File(5:0.0, 8:w1989, 9:T10."big-endian, network order" ("byte order (0:big-endian, network order)"), 10:12 ("count"), 11:w1988) -> (0:w1984:errorcluster, 2:w1982:dbl[], 3:w1985:refnum<file>)  [unwired: 1 in, 1 out]
        n1027 = Array To Cluster(array=w1982) -> (cluster=→"Cal values":T17)
        n1028 = Close File(refnum=w1985, error in=w1984) -> ()  [unwired: 2 out]
        n1029 = local write "Read Cal"(FALSE ("Read Cal")) -> ()
      }
      event "Stop": Value Change {
        n1030 = event-data() -> ("NewVal"=w1996:bool)  [unwired: 1 in, 5 out]
      }
      event "Trap position": Value Change {
        # "Need to rotate so X and Y don't get mixed up."
        n1031 = event-data() -> ()  [unwired: 1 in, 6 out]
        n1032 = local read "Mirror task"() -> (w1997:refnum<k21>)
        n1033 = Cluster To Array(cluster="Trap position") -> (array=w2000:dbl[])
        n1034 = Rotate 1D Array(1:w2000, 2:1 ("n")) -> (0:w1998:dbl[])
        n1035 = call-poly <vilib>:"DAQmx Write.vi"("task/channels in"=w1997, "data"=w1998) -> ("task out"=w2003:refnum<k21>, "error out"=w2002:errorcluster)  [unwired: 11 in, 1 out]
        n1036 = call <vilib>:"DAQmx Stop Task.vi"("task/channels in"=w2003, "error in"=w2002) -> ("error out"=w2001:errorcluster)  [unwired: 12 in, 1 out]
        n1037 = call <vilib>:"Simple Error Handler.vi"("error in (no error)"=w2001) -> ()  [unwired: 4 in, 5 out]
      }
      event "Trap delta": Value Change {
        n1038 = event-data() -> ()  [unwired: 1 in, 6 out]
        n1039 = local read "Pulling direction"() -> (w2006:bool)
        n1040 = local read "Fixed Y"() -> (w2010:dbl)
        n1041 = local read "Fixed X"() -> (w2009:dbl)
        n1042 = Select(t=w2010, s=w2006, f=w2009) -> (s? t:f=w2008:dbl)
        n1043 = Add(x="Trap delta", y=w2008) -> (x+y=w2005:dbl)
        n1044 = case shown="True" w2006 {
          tunnel: w2005 -> [w2011 w2012]
          frame False {
            n1045 = property on="X" class="DigNum (strict)"("Val(Sgnl)"=w2011) -> ()  [unwired: 2 in, 2 out]
          }
          frame True {
            n1046 = property on="Y" class="DigNum (strict)"("Val(Sgnl)"=w2012) -> ()  [unwired: 2 in, 2 out]
          }
        }
      }
      event "Raster scan": Value Change {
        w2049 = T15 1 items=["no dialog", "OK message", "continue or stop message", "OK message + warnings", "continue/stop + warnings"] ("type of dialog (OK msg:1)")
        w2034 = 0.0 ("minimum value")
        w2033 = 10.0 ("maximum value")
        # "Grab offset in pulling\ndirection and add to \ndelta values"
        # "Send offset in direction\nof not-pulling to DAQ"
        n1047 = event-data() -> ()  [unwired: 1 in, 6 out]
        n1048 = local read "Min delta"() -> (w2038:dbl)
        n1049 = local read "Max delta"() -> (w2036:dbl)
        n1050 = call-poly <vilib>:"DAQmx Create Virtual Channel.vi"("maximum value"=w2033, "minimum value"=w2034, "physical channels"=tag "Dev1/ao0") -> ("task out"=w2054:refnum<k21>, "error out"=w2053:errorcluster)  [unwired: 11 in]
        n1051 = local read "Fixed Y"() -> (w2042:dbl)
        n1052 = local read "Fixed X"() -> (w2043:dbl)
        n1053 = local read "Conv Y (nm/V)"() -> (w2029:dbl)
        n1054 = local read "Conv X (nm/V)"() -> (w2031:dbl)
        n1055 = local read "Speed (ms)"() -> (w2021:i32)
        n1056 = Subtract(x=w2036, y=w2038) -> (x-y=w2027:dbl)
        n1057 = Divide(x=w2021, y=2) -> (x/y=w2019:dbl)
        n1058 = Select(t=w2043, s="Pulling direction", f=w2042) -> (s? t:f=w2045:dbl)
        n1059 = Select(t=w2042, s="Pulling direction", f=w2043) -> (s? t:f=w2039:dbl)
        n1060 = Select(t=w2029, s="Pulling direction", f=w2031) -> (s? t:f=w2028:dbl)
        n1061 = Divide(x=w2027, y=w2019) -> (x/y=w2026:dbl)
        n1062 = call-poly <vilib>:"DAQmx Create Virtual Channel.vi"("task in"=w2054, "maximum value"=w2033, "minimum value"=w2034, "physical channels"=tag "Dev1/ao1", "error in"=w2053) -> ("task out"=w2048:refnum<k21>, "error out"=w2047:errorcluster)  [unwired: 9 in]
        n1063 = Multiply(x=w2027, y=w2028) -> (x*y=w2024:dbl)
        "Scan Range (nm)" <- w2024
        n1064 = Add(x=w2039, y=w2036) -> (x+y=w2041:dbl)
        n1065 = Divide(x=w2019, y=1000) -> (x/y=w2023:dbl)
        n1066 = Add(x=w2039, y=w2038) -> (x+y=w2040:dbl)
        n1067 = Divide(x=w2024, y=w2023) -> (x/y=→"Scan Speed (nm/s)":dbl)
        n1068 = node-c288(i64 1 ("Period")) -> (w2058:T12)  [unwired: 3 in]
        n1069 = timed-loop {
          tunnel: "Pulling direction" -> [w2080]
          tunnel: w2026 -> [w2076]
          tunnel: w2040 -> [w2079]
          tunnel: w2045 -> [w2068]
          tunnel: w2048 -> [w2078]
          tunnel: w2047 -> [w2077]
          tunnel: w2041 -> [w2075]
          tunnel: [w2072] -> w2052
          tunnel: [w2071] -> w2051
          tunnel: [w2066] -> w2013
          timing: w2058 -> [_]
          timing-out: [_] -> w2057
          tunnel: w2019 -> [w2067]
          tunnel: "Trap delta\nafter" -> [w2063]
          tunnel: [w2063] -> w2044
          i -> [w2070]
          stop <- w2066 stop-if-true
          n1070 = node-c288() -> ()  [unwired: 1 in, 1 out]
          n1071 = flat-sequence {
            tunnel: [w2089] -> w2074
            tunnel: [w2088] -> w2073
            tunnel: w2080 -> [w2087]
            tunnel: w2076 -> [w2094]
            tunnel: w2079 -> [w2093]
            tunnel: w2068 -> [w2092]
            tunnel: w2078 -> [w2091]
            tunnel: w2077 -> [w2090]
            tunnel: w2067 -> [w2086]
            tunnel: w2076 -> [w2125]
            tunnel: w2075 -> [w2124]
            tunnel: w2074 -> [w2131]
            tunnel: w2073 -> [w2130]
            tunnel: [w2129] -> w2072
            tunnel: [w2128] -> w2071
            tunnel: w2068 -> [w2126]
            frame #0 {
              n1072 = node-c288(i64 1 ("Period")) -> (w2085:T12)  [unwired: 3 in]
              n1073 = timed-loop {
                tunnel: w2094 -> [w2114]
                tunnel: w2093 -> [w2112]
                tunnel: w2092 -> [w2097]
                tunnel: w2091 -> [w2111]
                tunnel: w2090 -> [w2110]
                tunnel: [w2104] -> w2089
                tunnel: [w2105] -> w2088
                tunnel: w2087 -> [w2108]
                tunnel: w2086 -> [w2106]
                timing: w2085 -> [_]
                timing-out: [_] -> w2084
                i -> [w2102]
                stop <- w2107 stop-if-true
                n1074 = node-c288() -> ()  [unwired: 1 in, 1 out]
                n1075 = Multiply(x=w2114, y=w2102) -> (x*y=w2113:dbl)
                n1076 = Add(x=w2112, y=w2113) -> (x+y=w2098:dbl)
                n1077 = local read "Stop saving"() -> (w2095:bool)
                n1078 = local read "Stop raster"() -> (w2096:bool)
                n1079 = Build Array(w2097, w2098) -> (w2099:dbl[])
                n1080 = Build Array(w2098, w2097) -> (w2101:dbl[])
                n1081 = Greater Or Equal?(x=w2102, y=w2106) -> (x >= y?=w2103:bool)
                n1082 = Select(t=w2099, s=w2108, f=w2101) -> (s? t:f=w2100:dbl[])
                n1083 = Compound Arithmetic op=OR(w2103, w2096, w2095) -> (w2107:bool)
                n1084 = call-poly <vilib>:"DAQmx Write.vi"("task/channels in"=w2111, "auto start"=TRUE, "data"=w2100, "error in"=w2110) -> ("task out"=w2104:refnum<k21>, "error out"=w2105:errorcluster)  [unwired: 9 in, 1 out]
                n1085 = node-c288() -> ()  [unwired: 1 in, 1 out]
              }
              n1086 = node-c288(w2084) -> ()  [unwired: 1 out]
            }
            frame #1 {
              n1087 = local read "Pulling direction"() -> (w2127:bool)
              n1088 = node-c288(i64 1 ("Period")) -> (w2123:T12)  [unwired: 3 in]
              n1089 = timed-loop {
                tunnel: w2125 -> [w2142]
                tunnel: w2124 -> [w2145]
                tunnel: w2126 -> [w2136]
                tunnel: w2131 -> [w2154]
                tunnel: w2130 -> [w2146]
                tunnel: [w2138] -> w2129
                tunnel: [w2148] -> w2128
                tunnel: w2127 -> [w2150]
                timing: w2123 -> [_]
                timing-out: [_] -> w2122
                i -> [w2143]
                stop <- w2144 stop-if-true
                n1090 = node-c288() -> ()  [unwired: 1 in, 1 out]
                n1091 = Multiply(x=w2142, y=w2143) -> (x*y=w2141:dbl)
                n1092 = Subtract(x=w2145, y=w2141) -> (x-y=w2140:dbl)
                n1093 = Build Array(w2136, w2140) -> (w2149:dbl[])
                n1094 = local read "Speed (ms)"() -> (w2133:i32)
                n1095 = Build Array(w2140, w2136) -> (w2139:dbl[])
                n1096 = Select(t=w2149, s=w2150, f=w2139) -> (s? t:f=w2137:dbl[])
                n1097 = Divide(x=w2133, y=2) -> (x/y=w2132:dbl)
                n1098 = local read "Stop raster"() -> (w2152:bool)
                n1099 = local read "Stop saving"() -> (w2135:bool)
                n1100 = Decrement(x=w2132) -> (x-1=w2147:dbl)
                n1101 = call-poly <vilib>:"DAQmx Write.vi"("task/channels in"=w2154, "auto start"=TRUE, "data"=w2137, "error in"=w2146) -> ("task out"=w2138:refnum<k21>, "error out"=w2148:errorcluster)  [unwired: 9 in, 1 out]
                n1102 = Greater Or Equal?(x=w2143, y=w2147) -> (x >= y?=w2153:bool)
                n1103 = node-c288() -> ()  [unwired: 1 in, 1 out]
                n1104 = Compound Arithmetic op=OR(w2153, w2152, w2135) -> (w2144:bool)
              }
              n1105 = node-c288(w2122) -> ()  [unwired: 1 out]
            }
          }
          n1106 = local read "# scans"() -> (w2062:i32)
          n1107 = local read "Stop saving"() -> (w2061:bool)
          n1108 = Decrement(x=w2062) -> (x-1=w2064:i32)
          n1109 = Greater Or Equal?(x=w2070, y=w2064) -> (x >= y?=w2069:bool)
          n1110 = Compound Arithmetic op=OR(w2069, "Stop raster", w2061) -> (w2066:bool)
          n1111 = node-c288() -> ()  [unwired: 1 in, 1 out]
        }
        n1112 = node-c288(w2057) -> ()  [unwired: 1 out]
        n1113 = local read "Saving"() -> (w2014:bool)
        n1114 = call <vilib>:"DAQmx Clear Task.vi"("task in"=w2052, "error in"=w2051) -> ("error out"=w2050:errorcluster)  [unwired: 13 in]
        n1115 = Not(x=w2013) -> (.not. x?=w2046:bool)
        n1116 = Not(x=w2013) -> (.not. x?=w2037:bool)
        n1117 = And(x=w2014, y=w2013) -> (x .and. y?=w2015:bool)
        n1118 = property on="Trap delta" class="DigNum (strict)"("Val(Sgnl)"=w2044) -> ()  [unwired: 2 in, 2 out]
        n1119 = call <vilib>:"Simple Error Handler.vi"("type of dialog (OK msg:1)"=w2049, "error in (no error)"=w2050) -> ()  [unwired: 3 in, 5 out]
        n1120 = local write "Stop raster"(w2046) -> ()
        n1121 = local write "Raster scanning..."(w2037) -> ()
        n1122 = case shown="True" w2015 {
          frame False {
          }
          frame True {
            n1123 = property on="Stop saving" class="Bool (strict)"("Val(Sgnl)"=TRUE ("Value (Signaling)")) -> ()  [unwired: 2 in, 2 out]
          }
        }
        n1124 = And(x=w2013, y="Flow on\nafter raster?") -> (x .and. y?=w2016:bool)
        n1125 = case shown="True" w2016 {
          frame False {
          }
          frame True {
            n1126 = property on="Inject Sample" class="Bool (strict)"("Val(Sgnl)"=TRUE ("Value (Signaling)")) -> ()  [unwired: 2 in, 2 out]
          }
        }
        "Raster scanning..." <- TRUE ("Raster scanning...")
      }
      event "Fish": Value Change {
        n1127 = event-data() -> ()  [unwired: 1 in, 6 out]
        n1128 = local read "Fish"() -> (w2165:bool)
        n1129 = case shown="True" w2165 {
          frame False {
          }
          frame True {
            w2174 = 0.0 ("minimum value")
            w2175 = 10.0 ("maximum value")
            # "Grab offset in pulling\ndirection and add to \ndelta values"
            n1130 = call-poly <vilib>:"DAQmx Create Virtual Channel.vi"("maximum value"=w2175, "minimum value"=w2174, "physical channels"=tag "Dev1/ao0") -> ("task out"=w2179:refnum<k21>, "error out"=w2178:errorcluster)  [unwired: 11 in]
            n1131 = call-poly <vilib>:"DAQmx Create Virtual Channel.vi"("task in"=w2179, "maximum value"=w2175, "minimum value"=w2174, "physical channels"=tag "Dev1/ao1", "error in"=w2178) -> ("task out"=w2173:refnum<k21>, "error out"=w2172:errorcluster)  [unwired: 9 in]
            n1132 = node-c288(i64 1 ("Period")) -> (w2181:T12)  [unwired: 3 in]
            n1133 = timed-loop {
              timing: w2181 -> [_]
              timing-out: [_] -> w2180
              tunnel: w2173 -> [w2231]
              tunnel: w2172 -> [w2230]
              tunnel: [w2229] -> w2168
              tunnel: [w2228] -> w2167
              tunnel: [w2196] -> w2170
              tunnel: [w2210] -> w2166
              i -> [w2214]
              stop <- w2210 stop-if-true
              # "Send offset in direction\nof not-pulling to DAQ"
              n1134 = node-c288() -> ()  [unwired: 1 in, 1 out]
              n1135 = local read "Pulling direction"() -> (w2198:bool)
              n1136 = local read "Fixed Y"() -> (w2200:dbl)
              n1137 = local read "Fixed X"() -> (w2201:dbl)
              n1138 = Select(t=w2200, s=w2198, f=w2201) -> (s? t:f=w2202:dbl)
              n1139 = Add(x=w2202, y="Max fish\ndelta (V)") -> (x+y=w2204:dbl)
              n1140 = Subtract(x="Max fish\ndelta (V)", y="Min fish\ndelta (V)") -> (x-y=w2206:dbl)
              n1141 = Select(t=w2201, s=w2198, f=w2200) -> (s? t:f=w2199:dbl)
              n1142 = Divide(x=w2206, y="Fish Speed (ms)") -> (x/y=w2207:dbl)
              n1143 = flat-sequence {
                tunnel: w2198 -> [w2250]
                tunnel: w2199 -> [w2249]
                tunnel: w2231 -> [w2248]
                tunnel: w2230 -> [w2247]
                tunnel: w2207 -> [w2246]
                tunnel: w2204 -> [w2245]
                tunnel: "Fish Speed (ms)" -> [w2240]
                tunnel: [w2244] -> w2227
                tunnel: [w2243] -> w2226
                tunnel: [w2242] -> w2225
                tunnel: [w2241] -> w2224
                tunnel: [w2234] -> w2213
                tunnel: [w2233] -> w2197
                tunnel: [w2232] -> w2194
                tunnel: [w2297] -> w2223
                tunnel: w2227 -> [w2297]
                tunnel: [w2296] -> w2222
                tunnel: w2226 -> [w2296]
                tunnel: [w2295] -> w2221
                tunnel: w2225 -> [w2295]
                tunnel: [w2294] -> w2220
                tunnel: w2224 -> [w2294]
                tunnel: w2213 -> [w2293]
                tunnel: [w2293] -> w2212
                tunnel: w2197 -> [w2292]
                tunnel: [w2291] -> w2195
                tunnel: w2194 -> [w2291]
                tunnel: w2223 -> [w2308]
                tunnel: w2222 -> [w2307]
                tunnel: w2221 -> [w2306]
                tunnel: w2220 -> [w2305]
                tunnel: w2209 -> [w2304]
                tunnel: [w2303] -> w2229
                tunnel: [w2302] -> w2228
                tunnel: w2212 -> [w2301]
                tunnel: [w2300] -> w2196
                tunnel: w2195 -> [w2299]
                frame #0 {
                  n1144 = local read "Mean force (pN)"() -> (w2239:dbl)
                  n1145 = local read "Cutoff force (pN)"() -> (w2238:dbl)
                  n1146 = Less Or Equal?(x=w2239, y=w2238) -> (x <= y?=w2236:bool)
                  n1147 = And(x="Fish", y=w2236) -> (x .and. y?=w2237:bool)
                  n1148 = case shown="True" w2237 {
                    selector: w2237 -> [w2252 _]
                    tunnel: w2250 -> [w2255 w2271]
                    tunnel: w2249 -> [_ w2270]
                    tunnel: w2248 -> [w2257 w2269]
                    tunnel: w2247 -> [w2256 w2268]
                    tunnel: w2246 -> [w2254 w2267]
                    tunnel: w2245 -> [w2253 w2266]
                    tunnel: [w2257 w2265] -> w2244
                    tunnel: [w2256 w2264] -> w2243
                    tunnel: [w2255 w2263] -> w2242
                    tunnel: [w2253 w2262] -> w2232
                    tunnel: [w2254 w2261] -> w2241
                    tunnel: w2240 -> [_ w2260]
                    tunnel: [w2252 w2259] -> w2234
                    tunnel: [FALSE w2258] -> w2233
                    frame False {
                    }
                    frame True {
                      n1149 = while {
                        tunnel: w2271 -> [w2280]
                        tunnel: w2270 -> [w2279]
                        tunnel: w2269 -> [w2287]
                        tunnel: w2268 -> [w2286]
                        tunnel: w2267 -> [w2278]
                        tunnel: w2266 -> [w2284]
                        tunnel: [w2282] -> w2265
                        tunnel: [w2281] -> w2264
                        tunnel: [w2280] -> w2263
                        tunnel: [w2279] -> w2262
                        tunnel: [w2278] -> w2261
                        tunnel: w2260 -> [w2277]
                        tunnel: [w2272] -> w2259
                        tunnel: [w2272] -> w2258
                        i -> [w2276]
                        stop <- w2273 stop-if-true
                        n1150 = Multiply(x=w2278, y=w2276) -> (x*y=w2285:dbl)
                        n1151 = Subtract(x=w2284, y=w2285) -> (x-y=w2283:dbl)
                        n1152 = Build Array(w2279, w2283) -> (w2290:dbl[])
                        n1153 = Build Array(w2283, w2279) -> (w2289:dbl[])
                        n1154 = Greater Or Equal?(x=w2276, y=w2277) -> (x >= y?=w2272:bool)
                        n1155 = Select(t=w2290, s=w2280, f=w2289) -> (s? t:f=w2288:dbl[])
                        n1156 = local read "Fish"() -> (w2274:bool)
                        n1157 = Not(x=w2274) -> (.not. x?=w2275:bool)
                        n1158 = call-poly <vilib>:"DAQmx Write.vi"("task/channels in"=w2287, "data"=w2288, "error in"=w2286) -> ("task out"=w2282:refnum<k21>, "error out"=w2281:errorcluster)  [unwired: 10 in, 1 out]
                        n1159 = Compound Arithmetic op=OR(w2272, w2275) -> (w2273:bool)
                      }
                    }
                  }
                }
                frame #1 {
                  n1160 = case shown="True" w2292 {
                    frame False {
                    }
                    frame True {
                      n1161 = Wait (ms)(milliseconds to wait="Wait (ms)") -> ()  [unwired: 1 out]
                    }
                  }
                }
                frame #2 {
                  n1162 = case shown="True" w2301 {
                    tunnel: w2308 -> [w2311 w2320]
                    tunnel: w2307 -> [w2310 w2319]
                    tunnel: w2306 -> [_ w2318]
                    tunnel: w2305 -> [_ w2317]
                    tunnel: w2304 -> [_ w2316]
                    tunnel: [w2311 w2315] -> w2303
                    tunnel: [w2310 w2314] -> w2302
                    tunnel: [FALSE w2313] -> w2300
                    tunnel: w2299 -> [_ w2312]
                    frame False {
                    }
                    frame True {
                      n1163 = while {
                        tunnel: w2320 -> [w2348]
                        tunnel: w2319 -> [w2347]
                        tunnel: w2318 -> [w2330]
                        tunnel: w2317 -> [w2345]
                        tunnel: w2316 -> [w2344]
                        tunnel: [w2340] -> w2315
                        tunnel: [w2339] -> w2314
                        tunnel: [w2326] -> w2313
                        tunnel: w2312 -> [w2322]
                        i -> [w2331]
                        stop <- w2336 stop-if-true
                        # "If tether formed,\nimmediately change\nto new delta."
                        n1164 = local read "Fixed Y"() -> (w2321:dbl)
                        n1165 = local read "Fixed X"() -> (w2329:dbl)
                        n1166 = local read "Cutoff force (pN)"() -> (w2332:dbl)
                        n1167 = Multiply(x=w2345, y=w2331) -> (x*y=w2346:dbl)
                        n1168 = local read "Mean force (pN)"() -> (w2333:dbl)
                        n1169 = Add(x=w2344, y=w2346) -> (x+y=w2324:dbl)
                        n1170 = Select(t=w2321, s=w2330, f=w2329) -> (s? t:f=w2328:dbl)
                        n1171 = Greater?(x=w2333, y=w2332) -> (0:w2326:bool)
                        n1172 = Add(x=w2328, y="Delta after tether") -> (x+y=w2325:dbl)
                        n1173 = Select(t=w2325, s=w2326, f=w2324) -> (s? t:f=w2323:dbl)
                        n1174 = local read "Fish Speed (ms)"() -> (w2338:i32)
                        n1175 = Build Array(w2322, w2323) -> (w2343:dbl[])
                        n1176 = Build Array(w2323, w2322) -> (w2342:dbl[])
                        n1177 = Select(t=w2343, s=w2330, f=w2342) -> (s? t:f=w2341:dbl[])
                        n1178 = local read "Fish"() -> (w2335:bool)
                        n1179 = Greater Or Equal?(x=w2331, y=w2338) -> (x >= y?=w2337:bool)
                        n1180 = Not(x=w2335) -> (.not. x?=w2334:bool)
                        n1181 = call-poly <vilib>:"DAQmx Write.vi"("task/channels in"=w2348, "data"=w2341, "error in"=w2347) -> ("task out"=w2340:refnum<k21>, "error out"=w2339:errorcluster)  [unwired: 10 in, 1 out]
                        n1182 = Compound Arithmetic op=OR(w2337, w2334, w2326) -> (w2336:bool)
                      }
                    }
                  }
                }
              }
              n1183 = Add(x=w2202, y="Min fish\ndelta (V)") -> (x+y=w2209:dbl)
              n1184 = Decrement(x="# attempts") -> (x-1=w2218:dbl)
              n1185 = Greater Or Equal?(x=w2214, y=w2218) -> (x >= y?=w2217:bool)
              n1186 = local read "Mean force (pN)"() -> (w2216:dbl)
              n1187 = Greater?(x=w2216, y="Cutoff force (pN)") -> (0:w2211:bool)
              n1188 = Compound Arithmetic op=OR(w2196, w2211, w2217) -> (w2210:bool)
              n1189 = case shown="True" w2196 {
                frame False {
                }
                frame True {
                  n1190 = call <vilib>:"Beep.vi"() -> ()  [unwired: 12 in]
                }
              }
              n1191 = node-c288() -> ()  [unwired: 1 in, 1 out]
              "Tether" <- w2196
              "Attempt #" <- w2214
            }
            n1192 = node-c288(w2180) -> ()  [unwired: 1 out]
            n1193 = flat-sequence {
              tunnel: w2170 -> [w2188]
              tunnel: [w2188] -> w2169
              tunnel: w2168 -> [w2185]
              tunnel: w2167 -> [w2184]
              tunnel: w2166 -> [w2183]
              tunnel: w2169 -> [w2190]
              frame #0 {
                w2187 = T15 1 items=["no dialog", "OK message", "continue or stop message", "OK message + warnings", "continue/stop + warnings"] ("type of dialog (OK msg:1)")
                n1194 = call <vilib>:"DAQmx Clear Task.vi"("task in"=w2185, "error in"=w2184) -> ("error out"=w2186:errorcluster)  [unwired: 13 in]
                n1195 = Not(x=w2183) -> (.not. x?=w2182:bool)
                n1196 = local write "Fish"(w2182) -> ()
                n1197 = call <vilib>:"Simple Error Handler.vi"("type of dialog (OK msg:1)"=w2187, "error in (no error)"=w2186) -> ()  [unwired: 3 in, 5 out]
              }
              frame #1 {
                n1198 = And(x=w2190, y="Raster after\n tether?") -> (x .and. y?=w2191:bool)
                n1199 = case shown="True" w2191 {
                  selector: w2191 -> [_ w2193]
                  frame False {
                  }
                  frame True {
                    n1200 = property on="Raster scan" class="Bool (strict)"("Val(Sgnl)"=w2193) -> ()  [unwired: 2 in, 2 out]
                    n1201 = property on="Inject Sample" class="Bool (strict)"("Val(Sgnl)"=FALSE ("Value (Signaling)")) -> ()  [unwired: 2 in, 2 out]
                  }
                }
              }
            }
          }
        }
      }
      event "Load param": Value Change {
        n1202 = event-data() -> ()  [unwired: 1 in, 6 out]
        n1203 = property on="Scan Parameters" class="Arr (strict)"() -> ("Index Values"=w2364:u32[])  [unwired: 2 in, 2 out]
        n1204 = Index Array(array=w2364, index=0) -> (element=w2361:u32)
        n1205 = Index Array(array="Scan Parameters", index=w2361) -> (element=w2360:T18)
        n1206 = Unbundle(w2360) -> ("Max delta 2"=w2359:dbl, "Min delta 2"=w2355:dbl, "Speed (ms) 2"=w2358:i32, "# scans 2"=w2357:i32)  [unwired: 1 out]
        n1207 = property on="Max delta" class="DigNum (strict)"("Val(Sgnl)"=w2359) -> ()  [unwired: 2 in, 2 out]
        n1208 = local write "Load param"(FALSE ("Load param")) -> ()
        n1209 = property on="# scans" class="DigNum (strict)"("Val(Sgnl)"=w2357) -> ()  [unwired: 2 in, 2 out]
        n1210 = property on="Speed (ms)" class="DigNum (strict)"("Val(Sgnl)"=w2358) -> ()  [unwired: 2 in, 2 out]
        n1211 = property on="Min delta" class="DigNum (strict)"("Val(Sgnl)"=w2355) -> ()  [unwired: 2 in, 2 out]
      }
      event "Averaging Number": Value Change {
        n1212 = event-data() -> ()  [unwired: 1 in, 6 out]
        n1213 = local read "# Samples/channel (in)"() -> (w2368:i32)
        n1214 = local read "Averaging Number"() -> (w2366:i32)
        n1215 = Quotient & Remainder(x=w2368, y=w2366) -> (floor(x/y)=w2367:i32)  [unwired: 1 out]
        n1216 = Multiply(x=w2367, y=w2366) -> (x*y=w2365:i32)
        n1217 = local write "# Samples/channel (in)"(w2365) -> ()
      }
    }
    n1218 = node-c288() -> ()  [unwired: 1 in, 1 out]
  }
  n1219 = call <vilib>:"Simple Error Handler.vi"("error in (no error)"=w104) -> ()  [unwired: 4 in, 5 out]
  n1220 = node-c288() -> (w84:T12)  [unwired: 4 in]
  n1221 = timed-loop {
    timing: w84 -> [_]
    timing-out: [_] -> w83
    stop <- w2371 stop-if-true
    n1222 = node-c288() -> ()  [unwired: 1 in, 1 out]
    n1223 = event shown="[1] \"Stop\": Value Change" {
      selector: _ -> [_ _]
      dyn-events: _ -> [_ _]
      timeout: _ -> [_ _]
      tunnel: [_ "Stop"] -> w2371
      event Timeout {
        n1224 = event-data() -> ()  [unwired: 1 in, 2 out]
      }
      event "Stop": Value Change {
        n1225 = event-data() -> ()  [unwired: 1 in, 4 out]
      }
    }
    n1226 = node-c288() -> ()  [unwired: 1 in, 1 out]
  }
  n1227 = case shown="True" w73 {
    tunnel: w78 -> [_ w2377]
    tunnel: w77 -> [_ w2376]
    tunnel: w76 -> [_ w2375]
    frame False {
    }
    frame True {
      w2379 = T15 3 items=["no dialog", "OK message", "continue or stop message", "OK message + warnings", "continue/stop + warnings"] ("type of dialog (OK msg:1)")
      w2378 = T15 3 items=["no dialog", "OK message", "continue or stop message", "OK message + warnings", "continue/stop + warnings"] ("type of dialog (OK msg:1)")
      n1228 = call <vilib>:"DAQmx Clear Task.vi"("task in"=w2377, "error in"=w2375) -> ("error out"=w2380:errorcluster)  [unwired: 13 in]
      n1229 = call <vilib>:"DAQmx Clear Task.vi"("task in"=w2376) -> ("error out"=w2381:errorcluster)  [unwired: 14 in]
      n1230 = call <vilib>:"Simple Error Handler.vi"("type of dialog (OK msg:1)"=w2379, "error in (no error)"=w2380) -> ()  [unwired: 3 in, 5 out]
      n1231 = call <vilib>:"Simple Error Handler.vi"("type of dialog (OK msg:1)"=w2378, "error in (no error)"=w2381) -> ()  [unwired: 3 in, 5 out]
    }
  }
  n1232 = case shown="\"Force Feedback\", Default" "?" {
    frame "Force Feedback", Default {
    }
    frame "Raster scan" {
    }
  }
  n1233 = node-c288(w83) -> ()  [unwired: 1 out]
  n1234 = node-c288(w86) -> ()  [unwired: 1 out]
  n1235 = local write "Pause Mouse/Mirror Connection"(FALSE ("Pause Mouse/Mirror Connection")) -> ()
  n1236 = local write "Stop"(FALSE ("Stop all")) -> ()
  "CoordinatesMousePressed" <- T4 {"Horizontal"=0, "Vertical"=0} ("Coords when pressed")
  "Deflection" <- T4 {"Horizontal"=0, "Vertical"=0} ("Coords when pressed")
